vi "单体采集信息.vi"(0 "can卡类型":u8, 1 "设备索引号":u8, 2 "CAN端口":u8, 3 "VIC_Receive":refnum<vi>, 4 "数据":refnum<vi>, 5 "数据位置":refnum<vi>) -> ()   [LabVIEW 2013]
panel:
  out "Life:":dbl=25.0
  in  "213":bool
  in  "一次置位":bool
  in  "刷新":bool
  out "VCI_Receive 2":T1
  in  "板号":u8
  out "电池信息":T2
  in  "电池信息读取":bool
  out "时间":string
  in  "充电均衡":u32(colorbox)=6618880
  in  "放电均衡":u32(colorbox)=16711680
  out "均衡信息":string[][](table)=[["第1串", "1", "单体检测其它故障", "第25串", "1", "单体检测其它故障", "第49串", "1", "单体检测其它故障", "第73串", "1", "单体检测其它故障", "第97串", "1", "单体检测其它故障", "第121串", "1", "单体检测其它故障", "第145串", "1", "单体检测其它故障", "第169串", "1", "单体检测其它故障", "第193串", "1", "单体检测其它故障", "第217串", "1", "单体检测其它故障", "第241串", "1", "单体检测其它故障", "第265串", "1", "单体检测其它故障", "第289串", "1", "单体检测其它故障", ""], ["第2串", "", "", "第26串", "", "", "第50串", "", "", "第74串", "", "", "第98串", "", "", "第122串", "", "", "第146串", "", "", "第170串", "", "", "第194串", "", "", "第218串", "", "", "第242串", "", "", "第266串", "", "", "第290串", "", "", ""], ["第3串", "", "", "第27串", "", "", "第51串", "", "", "第75串", "", "", "第99串", "", "", "第123串", "", "", "第147串", "", "", "第171串", "", "", "第195串", "", "", "第219串", "", "", "第243串", "", "", "第267串", "", "", "第291串", "", "", ""], ["第4串", "", "", "第28串", "", "", "第52串", "", "", "第76串", "", "", "第100串", "", "", "第124串", "", "", "第148串", "", "", "第172串", "", "", "第196串", "", "", "第220串", "", "", "第244串", "", "", "第268串", "", "", "第292串", "", "", ""], ["第5串", "", "", "第29串", "", "", "第53串", "", "", "第77串", "", "", "第101串", "", "", "第125串", "", "", "第149串", "", "", "第173串", "", "", "第197串", "", "", "第221串", "", "", "第245串", "", "", "第269串", "", "", "第293串", "", "", ""], ["第6串", "", "", "第30串", "", "", "第54串", "", "", "第78串", "", "", "第102串", "", "", "第126串", "", "", "第150串", "", "", "第174串", "", "", "第198串", "", "", "第222串", "", "", "第246串", "", "", "第270串", "", "", "第294串", "", "", ""], ["第7串", "", "", "第31串", "", "", "第55串", "", "", "第79串", "", "", "第103串", "", "", "第127串", "", "", "第151串", "", "", "第175串", "", "", "第199串", "", "", "第223串", "", "", "第247串", "", "", "第271串", "", "", "第295串", "", "", ""], ["第8串", "", "", "第32串", "", "", "第56串", "", "", "第80串", "", "", "第104串", "", "", "第128串", "", "", "第152串", "", "", "第176串", "", "", "第200串", "", "", "第224串", "", "", "第248串", "", "", "第272串", "", "", "第296串", "", "", ""], ["第9串", "", "", "第33串", "", "", "第57串", "", "", "第81串", "", "", "第105串", "", "", "第129串", "", "", "第153串", "", "", "第177串", "", "", "第201串", "", "", "第225串", "", "", "第249串", "", "", "第273串", "", "", "第297串", "", "", ""], ["第10串", "", "", "第34串", "", "", "第58串", "", "", "第82串", "", "", "第106串", "", "", "第130串", "", "", "第154串", "", "", "第178串", "", "", "第202串", "", "", "第226串", "", "", "第250串", "", "", "第274串", "", "", "第298串", "", "", ""], ["第11串", "", "", "第35串", "", "", "第59串", "", "", "第83串", "", "", "第107串", "", "", "第131串", "", "", "第155串", "", "", "第179串", "", "", "第203串", "", "", "第227串", "", "", "第251串", "", "", "第275串", "", "", "第299串", "", "", ""], ["第12串", "", "", "第36串", "", "", "第60串", "", "", "第84串", "", "", "第108串", "", "", "第132串", "", "", "第156串", "", "", "第180串", "", "", "第204串", "", "", "第228串", "", "", "第252串", "", "", "第276串", "", "", "第300串", "", "", ""], ["第13串", "", "", "第37串", "", "", "第61串", "", "", "第85串", "", "", "第109串", "", "", "第133串", "", "", "第157串", "", "", "第181串", "", "", "第205串", "", "", "第229串", "", "", "第253串", "", "", "第277串", "", "", "", "", "", ""], ["第14串", "", "", "第38串", "", "", "第62串", "", "", "第86串", "", "", "第110串", "", "", "第134串", "", "", "第158串", "", "", "第182串", "", "", "第206串", "", "", "第230串", "", "", "第254串", "", "", "第278串", "", "", "", "", "", ""], ["第15串", "", "", "第39串", "", "", "第63串", "", "", "第87串", "", "", "第111串", "", "", "第135串", "", "", "第159串", "", "", "第183串", "", "", "第207串", "", "", "第231串", "", "", "第255串", "", "", "第279串", "", "", "", "", "", ""], ["第16串", "", "", "第40串", "", "", "第64串", "", "", "第88串", "", "", "第112串", "", "", "第136串", "", "", "第160串", "", "", "第184串", "", "", "第208串", "", "", "第232串", "", "", "第256串", "", "", "第280串", "", "", "", "", "", ""], ["第17串", "", "", "第41串", "", "", "第65串", "", "", "第89串", "", "", "第113串", "", "", "第137串", "", "", "第161串", "", "", "第185串", "", "", "第209串", "", "", "第233串", "", "", "第257串", "", "", "第281串", "", "", "", "", "", ""], ["第18串", "", "", "第42串", "", "", "第66串", "", "", "第90串", "", "", "第114串", "", "", "第138串", "", "", "第162串", "", "", "第186串", "", "", "第210串", "", "", "第234串", "", "", "第258串", "", "", "第282串", "", "", "", "", "", ""], ["第19串", "", "", "第43串", "", "", "第67串", "", "", "第91串", "", "", "第115串", "", "", "第139串", "", "", "第163串", "", "", "第187串", "", "", "第211串", "", "", "第235串", "", "", "第259串", "", "", "第283串", "", "", "", "", "", ""], ["第20串", "", "", "第44串", "", "", "第68串", "", "", "第92串", "", "", "第116串", "", "", "第140串", "", "", "第164串", "", "", "第188串", "", "", "第212串", "", "", "第236串", "", "", "第260串", "", "", "第284串", "", "", "", "", "", ""], ["第21串", "", "", "第45串", "", "", "第69串", "", "", "第93串", "", "", "第117串", "", "", "第141串", "", "", "第165串", "", "", "第189串", "", "", "第213串", "", "", "第237串", "", "", "第261串", "", "", "第285串", "", "", "", "", "", ""], ["第22串", "", "", "第46串", "", "", "第70串", "", "", "第94串", "", "", "第118串", "", "", "第142串", "", "", "第166串", "", "", "第190串", "", "", "第214串", "", "", "第238串", "", "", "第262串", "", "", "第286串", "", "", "", "", "", ""], ["第23串", "", "", "第47串", "", "", "第71串", "", "", "第95串", "", "", "第119串", "", "", "第143串", "", "", "第167串", "", "", "第191串", "", "", "第215串", "", "", "第239串", "", "", "第263串", "", "", "第287串", "", "", "", "", "", ""], ["第24串", "", "", "第48串", "", "", "第72串", "", "", "第96串", "", "", "第120串", "", "", "第144串", "", "", "第168串", "", "", "第192串", "", "", "第216串", "", "", "第240串", "", "", "第264串", "", "", "第288串", "", "", "", "", "", ""]]
  out "SOC":string[][](table)=[["第1串", "", "", "第25串", "", "", "第49串", "", "", "第73串", "", "", "第97串", "", "", "第121串", "", "", "第145串", "", "", "第169串", "", "", "第193串", "", "", "第217串", "", "", "第241串", "", "", "第265串", "", "", "第289串", "", "", ""], ["第2串", "", "", "第26串", "", "", "第50串", "", "", "第74串", "", "", "第98串", "", "", "第122串", "", "", "第146串", "", "", "第170串", "", "", "第194串", "", "", "第218串", "", "", "第242串", "", "", "第266串", "", "", "第290串", "", "", ""], ["第3串", "", "", "第27串", "", "", "第51串", "", "", "第75串", "", "", "第99串", "", "", "第123串", "", "", "第147串", "", "", "第171串", "", "", "第195串", "", "", "第219串", "", "", "第243串", "", "", "第267串", "", "", "第291串", "", "", ""], ["第4串", "", "", "第28串", "", "", "第52串", "", "", "第76串", "", "", "第100串", "", "", "第124串", "", "", "第148串", "", "", "第172串", "", "", "第196串", "", "", "第220串", "", "", "第244串", "", "", "第268串", "", "", "第292串", "", "", ""], ["第5串", "", "", "第29串", "", "", "第53串", "", "", "第77串", "", "", "第101串", "", "", "第125串", "", "", "第149串", "", "", "第173串", "", "", "第197串", "", "", "第221串", "", "", "第245串", "", "", "第269串", "", "", "第293串", "", "", ""], ["第6串", "", "", "第30串", "", "", "第54串", "", "", "第78串", "", "", "第102串", "", "", "第126串", "", "", "第150串", "", "", "第174串", "", "", "第198串", "", "", "第222串", "", "", "第246串", "", "", "第270串", "", "", "第294串", "", "", ""], ["第7串", "", "", "第31串", "", "", "第55串", "", "", "第79串", "", "", "第103串", "", "", "第127串", "", "", "第151串", "", "", "第175串", "", "", "第199串", "", "", "第223串", "", "", "第247串", "", "", "第271串", "", "", "第295串", "", "", ""], ["第8串", "", "", "第32串", "", "", "第56串", "", "", "第80串", "", "", "第104串", "", "", "第128串", "", "", "第152串", "", "", "第176串", "", "", "第200串", "", "", "第224串", "", "", "第248串", "", "", "第272串", "", "", "第296串", "", "", ""], ["第9串", "", "", "第33串", "", "", "第57串", "", "", "第81串", "", "", "第105串", "", "", "第129串", "", "", "第153串", "", "", "第177串", "", "", "第201串", "", "", "第225串", "", "", "第249串", "", "", "第273串", "", "", "第297串", "", "", ""], ["第10串", "", "", "第34串", "", "", "第58串", "", "", "第82串", "", "", "第106串", "", "", "第130串", "", "", "第154串", "", "", "第178串", "", "", "第202串", "", "", "第226串", "", "", "第250串", "", "", "第274串", "", "", "第298串", "", "", ""], ["第11串", "", "", "第35串", "", "", "第59串", "", "", "第83串", "", "", "第107串", "", "", "第131串", "", "", "第155串", "", "", "第179串", "", "", "第203串", "", "", "第227串", "", "", "第251串", "", "", "第275串", "", "", "第299串", "", "", ""], ["第12串", "", "", "第36串", "", "", "第60串", "", "", "第84串", "", "", "第108串", "", "", "第132串", "", "", "第156串", "", "", "第180串", "", "", "第204串", "", "", "第228串", "", "", "第252串", "", "", "第276串", "", "", "第300串", "", "", ""], ["第13串", "", "", "第37串", "", "", "第61串", "", "", "第85串", "", "", "第109串", "", "", "第133串", "", "", "第157串", "", "", "第181串", "", "", "第205串", "", "", "第229串", "", "", "第253串", "", "", "第277串", "", "", "", "", "", ""], ["第14串", "", "", "第38串", "", "", "第62串", "", "", "第86串", "", "", "第110串", "", "", "第134串", "", "", "第158串", "", "", "第182串", "", "", "第206串", "", "", "第230串", "", "", "第254串", "", "", "第278串", "", "", "", "", "", ""], ["第15串", "", "", "第39串", "", "", "第63串", "", "", "第87串", "", "", "第111串", "", "", "第135串", "", "", "第159串", "", "", "第183串", "", "", "第207串", "", "", "第231串", "", "", "第255串", "", "", "第279串", "", "", "", "", "", ""], ["第16串", "", "", "第40串", "", "", "第64串", "", "", "第88串", "", "", "第112串", "", "", "第136串", "", "", "第160串", "", "", "第184串", "", "", "第208串", "", "", "第232串", "", "", "第256串", "", "", "第280串", "", "", "", "", "", ""], ["第17串", "", "", "第41串", "", "", "第65串", "", "", "第89串", "", "", "第113串", "", "", "第137串", "", "", "第161串", "", "", "第185串", "", "", "第209串", "", "", "第233串", "", "", "第257串", "", "", "第281串", "", "", "", "", "", ""], ["第18串", "", "", "第42串", "", "", "第66串", "", "", "第90串", "", "", "第114串", "", "", "第138串", "", "", "第162串", "", "", "第186串", "", "", "第210串", "", "", "第234串", "", "", "第258串", "", "", "第282串", "", "", "", "", "", ""], ["第19串", "", "", "第43串", "", "", "第67串", "", "", "第91串", "", "", "第115串", "", "", "第139串", "", "", "第163串", "", "", "第187串", "", "", "第211串", "", "", "第235串", "", "", "第259串", "", "", "第283串", "", "", "", "", "", ""], ["第20串", "", "", "第44串", "", "", "第68串", "", "", "第92串", "", "", "第116串", "", "", "第140串", "", "", "第164串", "", "", "第188串", "", "", "第212串", "", "", "第236串", "", "", "第260串", "", "", "第284串", "", "", "", "", "", ""], ["第21串", "", "", "第45串", "", "", "第69串", "", "", "第93串", "", "", "第117串", "", "", "第141串", "", "", "第165串", "", "", "第189串", "", "", "第213串", "", "", "第237串", "", "", "第261串", "", "", "第285串", "", "", "", "", "", ""], ["第22串", "", "", "第46串", "", "", "第70串", "", "", "第94串", "", "", "第118串", "", "", "第142串", "", "", "第166串", "", "", "第190串", "", "", "第214串", "", "", "第238串", "", "", "第262串", "", "", "第286串", "", "", "", "", "", ""], ["第23串", "", "", "第47串", "", "", "第71串", "", "", "第95串", "", "", "第119串", "", "", "第143串", "", "", "第167串", "", "", "第191串", "", "", "第215串", "", "", "第239串", "", "", "第263串", "", "", "第287串", "", "", "", "", "", ""], ["第24串", "", "", "第48串", "", "", "第72串", "", "", "第96串", "", "", "第120串", "", "", "第144串", "", "", "第168串", "", "", "第192串", "", "", "第216串", "", "", "第240串", "", "", "第264串", "", "", "第288串", "", "", "", "", "", ""]]
  out "内阻":string[][](table)=[["第1串", "", "", "第25串", "", "", "第49串", "", "", "第73串", "", "", "第97串", "", "", "第121串", "", "", "第145串", "", "", "第169串", "", "", "第193串", "", "", "第217串", "", "", "第241串", "", "", "第265串", "", "", "第289串", "", "", ""], ["第2串", "", "", "第26串", "", "", "第50串", "", "", "第74串", "", "", "第98串", "", "", "第122串", "", "", "第146串", "", "", "第170串", "", "", "第194串", "", "", "第218串", "", "", "第242串", "", "", "第266串", "", "", "第290串", "", "", ""], ["第3串", "", "", "第27串", "", "", "第51串", "", "", "第75串", "", "", "第99串", "", "", "第123串", "", "", "第147串", "", "", "第171串", "", "", "第195串", "", "", "第219串", "", "", "第243串", "", "", "第267串", "", "", "第291串", "", "", ""], ["第4串", "", "", "第28串", "", "", "第52串", "", "", "第76串", "", "", "第100串", "", "", "第124串", "", "", "第148串", "", "", "第172串", "", "", "第196串", "", "", "第220串", "", "", "第244串", "", "", "第268串", "", "", "第292串", "", "", ""], ["第5串", "", "", "第29串", "", "", "第53串", "", "", "第77串", "", "", "第101串", "", "", "第125串", "", "", "第149串", "", "", "第173串", "", "", "第197串", "", "", "第221串", "", "", "第245串", "", "", "第269串", "", "", "第293串", "", "", ""], ["第6串", "", "", "第30串", "", "", "第54串", "", "", "第78串", "", "", "第102串", "", "", "第126串", "", "", "第150串", "", "", "第174串", "", "", "第198串", "", "", "第222串", "", "", "第246串", "", "", "第270串", "", "", "第294串", "", "", ""], ["第7串", "", "", "第31串", "", "", "第55串", "", "", "第79串", "", "", "第103串", "", "", "第127串", "", "", "第151串", "", "", "第175串", "", "", "第199串", "", "", "第223串", "", "", "第247串", "", "", "第271串", "", "", "第295串", "", "", ""], ["第8串", "", "", "第32串", "", "", "第56串", "", "", "第80串", "", "", "第104串", "", "", "第128串", "", "", "第152串", "", "", "第176串", "", "", "第200串", "", "", "第224串", "", "", "第248串", "", "", "第272串", "", "", "第296串", "", "", ""], ["第9串", "", "", "第33串", "", "", "第57串", "", "", "第81串", "", "", "第105串", "", "", "第129串", "", "", "第153串", "", "", "第177串", "", "", "第201串", "", "", "第225串", "", "", "第249串", "", "", "第273串", "", "", "第297串", "", "", ""], ["第10串", "", "", "第34串", "", "", "第58串", "", "", "第82串", "", "", "第106串", "", "", "第130串", "", "", "第154串", "", "", "第178串", "", "", "第202串", "", "", "第226串", "", "", "第250串", "", "", "第274串", "", "", "第298串", "", "", ""], ["第11串", "", "", "第35串", "", "", "第59串", "", "", "第83串", "", "", "第107串", "", "", "第131串", "", "", "第155串", "", "", "第179串", "", "", "第203串", "", "", "第227串", "", "", "第251串", "", "", "第275串", "", "", "第299串", "", "", ""], ["第12串", "", "", "第36串", "", "", "第60串", "", "", "第84串", "", "", "第108串", "", "", "第132串", "", "", "第156串", "", "", "第180串", "", "", "第204串", "", "", "第228串", "", "", "第252串", "", "", "第276串", "", "", "第300串", "", "", ""], ["第13串", "", "", "第37串", "", "", "第61串", "", "", "第85串", "", "", "第109串", "", "", "第133串", "", "", "第157串", "", "", "第181串", "", "", "第205串", "", "", "第229串", "", "", "第253串", "", "", "第277串", "", "", "", "", "", ""], ["第14串", "", "", "第38串", "", "", "第62串", "", "", "第86串", "", "", "第110串", "", "", "第134串", "", "", "第158串", "", "", "第182串", "", "", "第206串", "", "", "第230串", "", "", "第254串", "", "", "第278串", "", "", "", "", "", ""], ["第15串", "", "", "第39串", "", "", "第63串", "", "", "第87串", "", "", "第111串", "", "", "第135串", "", "", "第159串", "", "", "第183串", "", "", "第207串", "", "", "第231串", "", "", "第255串", "", "", "第279串", "", "", "", "", "", ""], ["第16串", "", "", "第40串", "", "", "第64串", "", "", "第88串", "", "", "第112串", "", "", "第136串", "", "", "第160串", "", "", "第184串", "", "", "第208串", "", "", "第232串", "", "", "第256串", "", "", "第280串", "", "", "", "", "", ""], ["第17串", "", "", "第41串", "", "", "第65串", "", "", "第89串", "", "", "第113串", "", "", "第137串", "", "", "第161串", "", "", "第185串", "", "", "第209串", "", "", "第233串", "", "", "第257串", "", "", "第281串", "", "", "", "", "", ""], ["第18串", "", "", "第42串", "", "", "第66串", "", "", "第90串", "", "", "第114串", "", "", "第138串", "", "", "第162串", "", "", "第186串", "", "", "第210串", "", "", "第234串", "", "", "第258串", "", "", "第282串", "", "", "", "", "", ""], ["第19串", "", "", "第43串", "", "", "第67串", "", "", "第91串", "", "", "第115串", "", "", "第139串", "", "", "第163串", "", "", "第187串", "", "", "第211串", "", "", "第235串", "", "", "第259串", "", "", "第283串", "", "", "", "", "", ""], ["第20串", "", "", "第44串", "", "", "第68串", "", "", "第92串", "", "", "第116串", "", "", "第140串", "", "", "第164串", "", "", "第188串", "", "", "第212串", "", "", "第236串", "", "", "第260串", "", "", "第284串", "", "", "", "", "", ""], ["第21串", "", "", "第45串", "", "", "第69串", "", "", "第93串", "", "", "第117串", "", "", "第141串", "", "", "第165串", "", "", "第189串", "", "", "第213串", "", "", "第237串", "", "", "第261串", "", "", "第285串", "", "", "", "", "", ""], ["第22串", "", "", "第46串", "", "", "第70串", "", "", "第94串", "", "", "第118串", "", "", "第142串", "", "", "第166串", "", "", "第190串", "", "", "第214串", "", "", "第238串", "", "", "第262串", "", "", "第286串", "", "", "", "", "", ""], ["第23串", "", "", "第47串", "", "", "第71串", "", "", "第95串", "", "", "第119串", "", "", "第143串", "", "", "第167串", "", "", "第191串", "", "", "第215串", "", "", "第239串", "", "", "第263串", "", "", "第287串", "", "", "", "", "", ""], ["第24串", "", "", "第48串", "", "", "第72串", "", "", "第96串", "", "", "第120串", "", "", "第144串", "", "", "第168串", "", "", "第192串", "", "", "第216串", "", "", "第240串", "", "", "第264串", "", "", "第288串", "", "", "", "", "", ""]]
  out "温度表格":string[][](table)=[["第1串", "", "", "第25串", "", "", "第49串", "", "", "第73串", "", "", "第97串", "", "", "第121串", "", "", "第145串", "", "", "第169串", "", "", "第193串", "", "", "第217串", "", "", "第241串", "", "", "第265串", "", "", "第289串", "", "", ""], ["第2串", "", "", "第26串", "", "", "第50串", "", "", "第74串", "", "", "第98串", "", "", "第122串", "", "", "第146串", "", "", "第170串", "", "", "第194串", "", "", "第218串", "", "", "第242串", "", "", "第266串", "", "", "第290串", "", "", ""], ["第3串", "", "", "第27串", "", "", "第51串", "", "", "第75串", "", "", "第99串", "", "", "第123串", "", "", "第147串", "", "", "第171串", "", "", "第195串", "", "", "第219串", "", "", "第243串", "", "", "第267串", "", "", "第291串", "", "", ""], ["第4串", "", "", "第28串", "", "", "第52串", "", "", "第76串", "", "", "第100串", "", "", "第124串", "", "", "第148串", "", "", "第172串", "", "", "第196串", "", "", "第220串", "", "", "第244串", "", "", "第268串", "", "", "第292串", "", "", ""], ["第5串", "", "", "第29串", "", "", "第53串", "", "", "第77串", "", "", "第101串", "", "", "第125串", "", "", "第149串", "", "", "第173串", "", "", "第197串", "", "", "第221串", "", "", "第245串", "", "", "第269串", "", "", "第293串", "", "", ""], ["第6串", "", "", "第30串", "", "", "第54串", "", "", "第78串", "", "", "第102串", "", "", "第126串", "", "", "第150串", "", "", "第174串", "", "", "第198串", "", "", "第222串", "", "", "第246串", "", "", "第270串", "", "", "第294串", "", "", ""], ["第7串", "", "", "第31串", "", "", "第55串", "", "", "第79串", "", "", "第103串", "", "", "第127串", "", "", "第151串", "", "", "第175串", "", "", "第199串", "", "", "第223串", "", "", "第247串", "", "", "第271串", "", "", "第295串", "", "", ""], ["第8串", "", "", "第32串", "", "", "第56串", "", "", "第80串", "", "", "第104串", "", "", "第128串", "", "", "第152串", "", "", "第176串", "", "", "第200串", "", "", "第224串", "", "", "第248串", "", "", "第272串", "", "", "第296串", "", "", ""], ["第9串", "", "", "第33串", "", "", "第57串", "", "", "第81串", "", "", "第105串", "", "", "第129串", "", "", "第153串", "", "", "第177串", "", "", "第201串", "", "", "第225串", "", "", "第249串", "", "", "第273串", "", "", "第297串", "", "", ""], ["第10串", "", "", "第34串", "", "", "第58串", "", "", "第82串", "", "", "第106串", "", "", "第130串", "", "", "第154串", "", "", "第178串", "", "", "第202串", "", "", "第226串", "", "", "第250串", "", "", "第274串", "", "", "第298串", "", "", ""], ["第11串", "", "", "第35串", "", "", "第59串", "", "", "第83串", "", "", "第107串", "", "", "第131串", "", "", "第155串", "", "", "第179串", "", "", "第203串", "", "", "第227串", "", "", "第251串", "", "", "第275串", "", "", "第299串", "", "", ""], ["第12串", "", "", "第36串", "", "", "第60串", "", "", "第84串", "", "", "第108串", "", "", "第132串", "", "", "第156串", "", "", "第180串", "", "", "第204串", "", "", "第228串", "", "", "第252串", "", "", "第276串", "", "", "第300串", "", "", ""], ["第13串", "", "", "第37串", "", "", "第61串", "", "", "第85串", "", "", "第109串", "", "", "第133串", "", "", "第157串", "", "", "第181串", "", "", "第205串", "", "", "第229串", "", "", "第253串", "", "", "第277串", "", "", "", "", "", ""], ["第14串", "", "", "第38串", "", "", "第62串", "", "", "第86串", "", "", "第110串", "", "", "第134串", "", "", "第158串", "", "", "第182串", "", "", "第206串", "", "", "第230串", "", "", "第254串", "", "", "第278串", "", "", "", "", "", ""], ["第15串", "", "", "第39串", "", "", "第63串", "", "", "第87串", "", "", "第111串", "", "", "第135串", "", "", "第159串", "", "", "第183串", "", "", "第207串", "", "", "第231串", "", "", "第255串", "", "", "第279串", "", "", "", "", "", ""], ["第16串", "", "", "第40串", "", "", "第64串", "", "", "第88串", "", "", "第112串", "", "", "第136串", "", "", "第160串", "", "", "第184串", "", "", "第208串", "", "", "第232串", "", "", "第256串", "", "", "第280串", "", "", "", "", "", ""], ["第17串", "", "", "第41串", "", "", "第65串", "", "", "第89串", "", "", "第113串", "", "", "第137串", "", "", "第161串", "", "", "第185串", "", "", "第209串", "", "", "第233串", "", "", "第257串", "", "", "第281串", "", "", "", "", "", ""], ["第18串", "", "", "第42串", "", "", "第66串", "", "", "第90串", "", "", "第114串", "", "", "第138串", "", "", "第162串", "", "", "第186串", "", "", "第210串", "", "", "第234串", "", "", "第258串", "", "", "第282串", "", "", "", "", "", ""], ["第19串", "", "", "第43串", "", "", "第67串", "", "", "第91串", "", "", "第115串", "", "", "第139串", "", "", "第163串", "", "", "第187串", "", "", "第211串", "", "", "第235串", "", "", "第259串", "", "", "第283串", "", "", "", "", "", ""], ["第20串", "", "", "第44串", "", "", "第68串", "", "", "第92串", "", "", "第116串", "", "", "第140串", "", "", "第164串", "", "", "第188串", "", "", "第212串", "", "", "第236串", "", "", "第260串", "", "", "第284串", "", "", "", "", "", ""], ["第21串", "", "", "第45串", "", "", "第69串", "", "", "第93串", "", "", "第117串", "", "", "第141串", "", "", "第165串", "", "", "第189串", "", "", "第213串", "", "", "第237串", "", "", "第261串", "", "", "第285串", "", "", "", "", "", ""], ["第22串", "", "", "第46串", "", "", "第70串", "", "", "第94串", "", "", "第118串", "", "", "第142串", "", "", "第166串", "", "", "第190串", "", "", "第214串", "", "", "第238串", "", "", "第262串", "", "", "第286串", "", "", "", "", "", ""], ["第23串", "", "", "第47串", "", "", "第71串", "", "", "第95串", "", "", "第119串", "", "", "第143串", "", "", "第167串", "", "", "第191串", "", "", "第215串", "", "", "第239串", "", "", "第263串", "", "", "第287串", "", "", "", "", "", ""], ["第24串", "", "", "第48串", "", "", "第72串", "", "", "第96串", "", "", "第120串", "", "", "第144串", "", "", "第168串", "", "", "第192串", "", "", "第216串", "", "", "第240串", "", "", "第264串", "", "", "第288串", "", "", "", "", "", ""]]
  in  "主界面选项":T3(radio)
  in  "电池信息选项":enum16{"电池信息", "历史信息"}(ring)
  out "位置":dbl[](array[numeric])
  out "输出数据":dbl[](array[numeric])
  in  "命令":u32=133
  in  "VCI_Receive":T1 {"Rsv3" max=0 format="%x"; "Rsv2" min=101 format="%x"; "Rsv1" format="%x"; "Data8" format="%x"; "Data7" format="%x"; "Data6" format="%x"; "Data5" format="%x"; "Data4" format="%x"; "Data3" format="%x"; "Data2" format="%x"; "Data1" format="%x"; "DataLen" format="%x"; "ExternFlag" format="%x"; "RemoteFlag" format="%x"; "SendType" format="%x"; "TimeFlag" format="%x"; "TimeStamp" format="%x"; "ID" format="%x"}
  out "状态":bool
  in  "停止":bool
  in  "选项卡控件":enum32{"单体电压", "单体温度", "单体内阻", "单体SOC"}(tab)
  in  "偏差":dbl=0.008 format="%.3f"
  in  "基准":dbl=3.3 format="%.3f"
  out "等待均衡":u32(colorbox)=16776770
  in  "故障信息选择按键 2":enum32{"单选选项2", "单选选项2 2", "单选选项2 3", "单选选项1"}(radio)=enum."单选选项1"
  out "电压选择":enum32{"1-96", "97-192", "193-288", "289-300"}(tab)
  out "1":T4={"1 102"={"第1串"=0.0, "第2串"=0.0, "第3串"=0.0, "第4串"=0.0, "第5串"=0.0, "第6串"=0.0, "第7串"=0.0, "第8串"=0.0, "第9串"=0.0, "第10串"=0.0, "第11串"=0.0, "第12串"=0.0, "第一串 2"=0.0, "第一串 4"=0.0, "第一串 6"=0.0, "第一串 8"=0.0, "第一串 10"=0.0, "第一串 12"=0.0, "第一串 14"=0.0, "第一串 16"=0.0, "第一串 18"=0.0, "第一串 20"=0.0, "第一串 22"=0.0, "第一串 24"=0.0}, "1 3"={"第13串"=0.0, "第14串"=0.0, "第15串"=0.0, "第16串"=0.0, "第17串"=0.0, "第18串"=0.0, "第19串"=0.0, "第20串"=0.0, "第21串"=0.0, "第22串"=0.0, "第23串"=0.0, "第24串"=0.0, "第一串 2"=0.0, "第一串 4"=0.0, "第一串 6"=0.0, "第一串 8"=0.0, "第一串 10"=0.0, "第一串 12"=0.0, "第一串 14"=0.0, "第一串 16"=0.0, "第一串 18"=0.0, "第一串 20"=0.0, "第一串 22"=0.0, "第一串 24"=0.0}, "1 4"={"第25串"=0.0, "第26串"=0.0, "第27串"=0.0, "第28串"=0.0, "第29串"=0.0, "第30串"=0.0, "第31串"=0.0, "第32串"=0.0, "第33串"=0.0, "第34串"=0.0, "第35串"=0.0, "第36串"=0.0, "第一串 2"=0.0, "第一串 4"=0.0, "第一串 6"=0.0, "第一串 8"=0.0, "第一串 10"=0.0, "第一串 12"=0.0, "第一串 14"=0.0, "第一串 16"=0.0, "第一串 18"=0.0, "第一串 20"=0.0, "第一串 22"=0.0, "第一串 24"=0.0}, "1 6"={"第37串"=0.0, "第38串"=0.0, "第39串"=0.0, "第40串"=0.0, "第41串"=0.0, "第42串"=0.0, "第43串"=0.0, "第44串"=0.0, "第45串"=0.0, "第46串"=0.0, "第47串"=0.0, "第48串"=0.0, "第一串 2"=0.0, "第一串 4"=0.0, "第一串 6"=0.0, "第一串 8"=0.0, "第一串 10"=0.0, "第一串 12"=0.0, "第一串 14"=0.0, "第一串 16"=0.0, "第一串 18"=0.0, "第一串 20"=0.0, "第一串 22"=0.0, "第一串 24"=0.0}, "1 7"={"第49串"=0.0, "第50串"=0.0, "第51串"=0.0, "第52串"=0.0, "第53串"=0.0, "第54串"=0.0, "第55串"=0.0, "第56串"=0.0, "第57串"=0.0, "第58串"=0.0, "第59串"=0.0, "第60串"=0.0, "第一串 2"=0.0, "第一串 4"=0.0, "第一串 6"=0.0, "第一串 8"=0.0, "第一串 10"=0.0, "第一串 12"=0.0, "第一串 14"=0.0, "第一串 16"=0.0, "第一串 18"=0.0, "第一串 20"=0.0, "第一串 22"=0.0, "第一串 24"=0.0}, "1 8"={"第61串"=0.0, "第62串"=0.0, "第63串"=0.0, "第64串"=0.0, "第65串"=0.0, "第66串"=0.0, "第67串"=0.0, "第68串"=0.0, "第69串"=0.0, "第70串"=0.0, "第71串"=0.0, "第72串"=0.0, "第一串 2"=0.0, "第一串 4"=0.0, "第一串 6"=0.0, "第一串 8"=0.0, "第一串 10"=0.0, "第一串 12"=0.0, "第一串 14"=0.0, "第一串 16"=0.0, "第一串 18"=0.0, "第一串 20"=0.0, "第一串 22"=0.0, "第一串 24"=0.0}, "1 9"={"第73串"=0.0, "第74串"=0.0, "第75串"=0.0, "第76串"=0.0, "第77串"=0.0, "第78串"=0.0, "第79串"=0.0, "第80串"=0.0, "第81串"=0.0, "第82串"=0.0, "第83串"=0.0, "第84串"=0.0, "第一串 2"=0.0, "第一串 4"=0.0, "第一串 6"=0.0, "第一串 8"=0.0, "第一串 10"=0.0, "第一串 12"=0.0, "第一串 14"=0.0, "第一串 16"=0.0, "第一串 18"=0.0, "第一串 20"=0.0, "第一串 22"=0.0, "第一串 24"=0.0}, "1 10"={"第85串"=0.0, "第86串"=0.0, "第87串"=0.0, "第88串"=0.0, "第89串"=0.0, "第90串"=0.0, "第91串"=0.0, "第92串"=0.0, "第93串"=0.0, "第94串"=0.0, "第95串"=0.0, "第96串"=0.0, "第一串 2"=0.0, "第一串 4"=0.0, "第一串 6"=0.0, "第一串 8"=0.0, "第一串 10"=0.0, "第一串 12"=0.0, "第一串 14"=0.0, "第一串 16"=0.0, "第一串 18"=0.0, "第一串 20"=0.0, "第一串 22"=0.0, "第一串 24"=0.0}, "1 12"={"充电1"=13816530, "充电1"=13816530, "充电1"=13816530, "充电1"=13816530, "充电1"=13816530, "充电1"=13816530, "充电1"=13816530, "充电1"=13816530, "充电1"=13816530, "充电1"=13816530, "充电1"=13816530, "充电1"=13816530}, "1 28"={"充电1"=13816530, "充电1"=13816530, "充电1"=13816530, "充电1"=13816530, "充电1"=13816530, "充电1"=13816530, "充电1"=13816530, "充电1"=13816530, "充电1"=13816530, "充电1"=13816530, "充电1"=13816530, "充电1"=13816530}, "1 25"={"充电1"=0, "充电1"=0, "充电1"=0, "充电1"=0, "充电1"=0, "充电1"=0, "充电1"=0, "充电1"=0, "充电1"=0, "充电1"=0, "充电1"=0, "充电1"=0}, "1 31"={"充电1"=0, "充电1"=0, "充电1"=0, "充电1"=0, "充电1"=0, "充电1"=0, "充电1"=0, "充电1"=0, "充电1"=0, "充电1"=0, "充电1"=0, "充电1"=0}, "1 16"={"充电1"=0, "充电1"=0, "充电1"=0, "充电1"=0, "充电1"=0, "充电1"=0, "充电1"=0, "充电1"=0, "充电1"=0, "充电1"=0, "充电1"=0, "充电1"=0}, "1 19"={"充电1"=0, "充电1"=0, "充电1"=0, "充电1"=0, "充电1"=0, "充电1"=0, "充电1"=0, "充电1"=0, "充电1"=0, "充电1"=0, "充电1"=0, "充电1"=0}, "1 22"={"充电1"=0, "充电1"=0, "充电1"=0, "充电1"=0, "充电1"=0, "充电1"=0, "充电1"=0, "充电1"=0, "充电1"=0, "充电1"=0, "充电1"=0, "充电1"=0}, "1 34"={"充电1"=0, "充电1"=0, "充电1"=0, "充电1"=0, "充电1"=0, "充电1"=0, "充电1"=0, "充电1"=0, "充电1"=0, "充电1"=0, "充电1"=0, "充电1"=0}, "1 11"={"充电1"=13816530, "充电1"=13816530, "充电1"=13816530, "充电1"=13816530, "充电1"=13816530, "充电1"=13816530, "充电1"=13816530, "充电1"=13816530, "充电1"=13816530, "充电1"=13816530, "充电1"=13816530, "充电1"=13816530}, "1 27"={"充电1"=0, "充电1"=0, "充电1"=0, "充电1"=0, "充电1"=0, "充电1"=0, "充电1"=0, "充电1"=0, "充电1"=0, "充电1"=0, "充电1"=0, "充电1"=0}, "1 24"={"充电1"=0, "充电1"=0, "充电1"=0, "充电1"=0, "充电1"=0, "充电1"=0, "充电1"=0, "充电1"=0, "充电1"=0, "充电1"=0, "充电1"=0, "充电1"=0}, "1 30"={"充电1"=0, "充电1"=0, "充电1"=0, "充电1"=0, "充电1"=0, "充电1"=0, "充电1"=0, "充电1"=0, "充电1"=0, "充电1"=0, "充电1"=0, "充电1"=0}, "1 15"={"充电1"=0, "充电1"=0, "充电1"=0, "充电1"=0, "充电1"=0, "充电1"=0, "充电1"=0, "充电1"=0, "充电1"=0, "充电1"=0, "充电1"=0, "充电1"=0}, "1 18"={"充电1"=0, "充电1"=0, "充电1"=0, "充电1"=0, "充电1"=0, "充电1"=0, "充电1"=0, "充电1"=0, "充电1"=0, "充电1"=0, "充电1"=0, "充电1"=0}, "1 21"={"充电1"=0, "充电1"=0, "充电1"=0, "充电1"=0, "充电1"=0, "充电1"=0, "充电1"=0, "充电1"=0, "充电1"=0, "充电1"=0, "充电1"=0, "充电1"=0}, "1 33"={"充电1"=0, "充电1"=0, "充电1"=0, "充电1"=0, "充电1"=0, "充电1"=0, "充电1"=0, "充电1"=0, "充电1"=0, "充电1"=0, "充电1"=0, "充电1"=0}, "1 13"={"均衡故障"=0, "均衡故障 2"=0.0, "均衡故障 3"=0.0, "均衡故障 4"=0.0, "均衡故障 5"=0.0, "均衡故障 6"=0.0, "均衡故障 7"=0.0, "均衡故障 8"=0.0, "均衡故障 9"=0.0, "均衡故障 10"=0.0, "均衡故障 11"=0.0, "均衡故障 12"=0.0}, "1 26"={"均衡故障"=0, "均衡故障 2"=0.0, "均衡故障 3"=0.0, "均衡故障 4"=0.0, "均衡故障 5"=0.0, "均衡故障 6"=0.0, "均衡故障 7"=0.0, "均衡故障 8"=0.0, "均衡故障 9"=0.0, "均衡故障 10"=0.0, "均衡故障 11"=0.0, "均衡故障 12"=0.0}, "1 23"={"均衡故障"=0, "均衡故障 2"=0.0, "均衡故障 3"=0.0, "均衡故障 4"=0.0, "均衡故障 5"=0.0, "均衡故障 6"=0.0, "均衡故障 7"=0.0, "均衡故障 8"=0.0, "均衡故障 9"=0.0, "均衡故障 10"=0.0, "均衡故障 11"=0.0, "均衡故障 12"=0.0}, "1 29"={"均衡故障"=0, "均衡故障 2"=0.0, "均衡故障 3"=0.0, "均衡故障 4"=0.0, "均衡故障 5"=0.0, "均衡故障 6"=0.0, "均衡故障 7"=0.0, "均衡故障 8"=0.0, "均衡故障 9"=0.0, "均衡故障 10"=0.0, "均衡故障 11"=0.0, "均衡故障 12"=0.0}, "1 14"={"均衡故障"=0, "均衡故障 2"=0.0, "均衡故障 3"=0.0, "均衡故障 4"=0.0, "均衡故障 5"=0.0, "均衡故障 6"=0.0, "均衡故障 7"=0.0, "均衡故障 8"=0.0, "均衡故障 9"=0.0, "均衡故障 10"=0.0, "均衡故障 11"=0.0, "均衡故障 12"=0.0}, "1 17"={"均衡故障"=0, "均衡故障 2"=0.0, "均衡故障 3"=0.0, "均衡故障 4"=0.0, "均衡故障 5"=0.0, "均衡故障 6"=0.0, "均衡故障 7"=0.0, "均衡故障 8"=0.0, "均衡故障 9"=0.0, "均衡故障 10"=0.0, "均衡故障 11"=0.0, "均衡故障 12"=0.0}, "1 20"={"均衡故障"=0, "均衡故障 2"=0.0, "均衡故障 3"=0.0, "均衡故障 4"=0.0, "均衡故障 5"=0.0, "均衡故障 6"=0.0, "均衡故障 7"=0.0, "均衡故障 8"=0.0, "均衡故障 9"=0.0, "均衡故障 10"=0.0, "均衡故障 11"=0.0, "均衡故障 12"=0.0}, "1 32"={"均衡故障"=0, "均衡故障 2"=0.0, "均衡故障 3"=0.0, "均衡故障 4"=0.0, "均衡故障 5"=0.0, "均衡故障 6"=0.0, "均衡故障 7"=0.0, "均衡故障 8"=0.0, "均衡故障 9"=0.0, "均衡故障 10"=0.0, "均衡故障 11"=0.0, "均衡故障 12"=0.0}} {"1 102"."第一串 24" format="%#.2f"; "1 102"."第12串" format="%.3f"; "1 102"."第一串 22" format="%#.2f"; "1 102"."第11串" format="%.3f"; "1 102"."第一串 20" format="%#.2f"; "1 102"."第10串" format="%.3f"; "1 102"."第一串 18" format="%#.2f"; "1 102"."第9串" format="%.3f"; "1 102"."第一串 16" format="%#.2f"; "1 102"."第8串" format="%.3f"; "1 102"."第一串 14" format="%#.2f"; "1 102"."第7串" format="%.3f"; "1 102"."第一串 12" format="%#.2f"; "1 102"."第6串" format="%.3f"; "1 102"."第一串 10" format="%#.2f"; "1 102"."第5串" format="%.3f"; "1 102"."第一串 8" format="%#.2f"; "1 102"."第4串" format="%.3f"; "1 102"."第一串 6" format="%#.2f"; "1 102"."第3串" format="%.3f"; "1 102"."第一串 4" format="%#.2f"; "1 102"."第2串" format="%.3f"; "1 102"."第一串 2" format="%#.2f"; "1 102"."第1串" format="%.3f"; "1 10"."第96串" format="%.3f"; "1 10"."第95串" format="%.3f"; "1 10"."第94串" format="%.3f"; "1 10"."第93串" format="%.3f"; "1 10"."第92串" format="%.3f"; "1 10"."第91串" format="%.3f"; "1 10"."第90串" format="%.3f"; "1 10"."第89串" format="%.3f"; "1 10"."第88串" format="%.3f"; "1 10"."第87串" format="%.3f"; "1 10"."第86串" format="%.3f"; "1 10"."第85串" format="%.3f"; "1 9"."第84串" format="%.3f"; "1 9"."第83串" format="%.3f"; "1 9"."第82串" format="%.3f"; "1 9"."第81串" format="%.3f"; "1 9"."第80串" format="%.3f"; "1 9"."第79串" format="%.3f"; "1 9"."第78串" format="%.3f"; "1 9"."第77串" format="%.3f"; "1 9"."第76串" format="%.3f"; "1 9"."第75串" format="%.3f"; "1 9"."第74串" format="%.3f"; "1 9"."第73串" format="%.3f"; "1 8"."第72串" format="%.3f"; "1 8"."第71串" format="%.3f"; "1 8"."第70串" format="%.3f"; "1 8"."第69串" format="%.3f"; "1 8"."第68串" format="%.3f"; "1 8"."第67串" format="%.3f"; "1 8"."第66串" format="%.3f"; "1 8"."第65串" format="%.3f"; "1 8"."第64串" format="%.3f"; "1 8"."第63串" format="%.3f"; "1 8"."第62串" format="%.3f"; "1 8"."第61串" format="%.3f"; "1 7"."第60串" format="%.3f"; "1 7"."第59串" format="%.3f"; "1 7"."第58串" format="%.3f"; "1 7"."第57串" format="%.3f"; "1 7"."第56串" format="%.3f"; "1 7"."第55串" format="%.3f"; "1 7"."第54串" format="%.3f"; "1 7"."第53串" format="%.3f"; "1 7"."第52串" format="%.3f"; "1 7"."第51串" format="%.3f"; "1 7"."第50串" format="%.3f"; "1 7"."第49串" format="%.3f"; "1 6"."第48串" format="%.3f"; "1 6"."第47串" format="%.3f"; "1 6"."第46串" format="%.3f"; "1 6"."第45串" format="%.3f"; "1 6"."第44串" format="%.3f"; "1 6"."第43串" format="%.3f"; "1 6"."第42串" format="%.3f"; "1 6"."第41串" format="%.3f"; "1 6"."第40串" format="%.3f"; "1 6"."第39串" format="%.3f"; "1 6"."第38串" format="%.3f"; "1 6"."第37串" format="%.3f"; "1 4"."第36串" format="%.3f"; "1 4"."第35串" format="%.3f"; "1 4"."第34串" format="%.3f"; "1 4"."第33串" format="%.3f"; "1 4"."第32串" format="%.3f"; "1 4"."第31串" format="%.3f"; "1 4"."第30串" format="%.3f"; "1 4"."第29串" format="%.3f"; "1 4"."第28串" format="%.3f"; "1 4"."第27串" format="%.3f"; "1 4"."第26串" format="%.3f"; "1 4"."第25串" format="%.3f"; "1 3"."第24串" format="%.3f"; "1 3"."第23串" format="%.3f"; "1 3"."第22串" format="%.3f"; "1 3"."第21串" format="%.3f"; "1 3"."第20串" format="%.3f"; "1 3"."第19串" format="%.3f"; "1 3"."第18串" format="%.3f"; "1 3"."第17串" format="%.3f"; "1 3"."第16串" format="%.3f"; "1 3"."第15串" format="%.3f"; "1 3"."第14串" format="%.3f"; "1 3"."第13串" format="%.3f"}
  out "2":T5={"1 26"={"第97串"=0.0, "第98串"=0.0, "第99串"=0.0, "第100串"=0.0, "第101串"=0.0, "第102串"=0.0, "第103串"=0.0, "第104串"=0.0, "第105串"=0.0, "第106串"=0.0, "第107串"=0.0, "第108串"=0.0, "第一串 2"=0.0, "第一串 4"=0.0, "第一串 6"=0.0, "第一串 8"=0.0, "第一串 10"=0.0, "第一串 12"=0.0, "第一串 14"=0.0, "第一串 16"=0.0, "第一串 18"=0.0, "第一串 20"=0.0, "第一串 22"=0.0, "第一串 24"=0.0}, "1 27"={"第109串"=0.0, "第110串"=0.0, "第111串"=0.0, "第112串"=0.0, "第113串"=0.0, "第114串"=0.0, "第115串"=0.0, "第116串"=0.0, "第117串"=0.0, "第118串"=0.0, "第119串"=0.0, "第120串"=0.0, "第一串 2"=0.0, "第一串 4"=0.0, "第一串 6"=0.0, "第一串 8"=0.0, "第一串 10"=0.0, "第一串 12"=0.0, "第一串 14"=0.0, "第一串 16"=0.0, "第一串 18"=0.0, "第一串 20"=0.0, "第一串 22"=0.0, "第一串 24"=0.0}, "1 28"={"第121串"=0.0, "第122串"=0.0, "第123串"=0.0, "第124串"=0.0, "第125串"=0.0, "第126串"=0.0, "第127串"=0.0, "第128串"=0.0, "第129串"=0.0, "第130串"=0.0, "第131串"=0.0, "第132串"=0.0, "第一串 2"=0.0, "第一串 4"=0.0, "第一串 6"=0.0, "第一串 8"=0.0, "第一串 10"=0.0, "第一串 12"=0.0, "第一串 14"=0.0, "第一串 16"=0.0, "第一串 18"=0.0, "第一串 20"=0.0, "第一串 22"=0.0, "第一串 24"=0.0}, "1 29"={"第133串"=0.0, "第134串"=0.0, "第135串"=0.0, "第136串"=0.0, "第137串"=0.0, "第138串"=0.0, "第139串"=0.0, "第140串"=0.0, "第141串"=0.0, "第142串"=0.0, "第143串"=0.0, "第144串"=0.0, "第一串 2"=0.0, "第一串 4"=0.0, "第一串 6"=0.0, "第一串 8"=0.0, "第一串 10"=0.0, "第一串 12"=0.0, "第一串 14"=0.0, "第一串 16"=0.0, "第一串 18"=0.0, "第一串 20"=0.0, "第一串 22"=0.0, "第一串 24"=0.0}, "1 30"={"第145串"=0.0, "第146串"=0.0, "第147串"=0.0, "第148串"=0.0, "第149串"=0.0, "第150串"=0.0, "第151串"=0.0, "第152串"=0.0, "第153串"=0.0, "第154串"=0.0, "第155串"=0.0, "第156串"=0.0, "第一串 2"=0.0, "第一串 4"=0.0, "第一串 6"=0.0, "第一串 8"=0.0, "第一串 10"=0.0, "第一串 12"=0.0, "第一串 14"=0.0, "第一串 16"=0.0, "第一串 18"=0.0, "第一串 20"=0.0, "第一串 22"=0.0, "第一串 24"=0.0}, "1 31"={"第157串"=0.0, "第158串"=0.0, "第159串"=0.0, "第160串"=0.0, "第161串"=0.0, "第162串"=0.0, "第163串"=0.0, "第164串"=0.0, "第165串"=0.0, "第166串"=0.0, "第167串"=0.0, "第168串"=0.0, "第一串 2"=0.0, "第一串 4"=0.0, "第一串 6"=0.0, "第一串 8"=0.0, "第一串 10"=0.0, "第一串 12"=0.0, "第一串 14"=0.0, "第一串 16"=0.0, "第一串 18"=0.0, "第一串 20"=0.0, "第一串 22"=0.0, "第一串 24"=0.0}, "1 32"={"第169串"=0.0, "第170串"=0.0, "第171串"=0.0, "第172串"=0.0, "第173串"=0.0, "第174串"=0.0, "第175串"=0.0, "第176串"=0.0, "第177串"=0.0, "第178串"=0.0, "第179串"=0.0, "第180串"=0.0, "第一串 2"=0.0, "第一串 4"=0.0, "第一串 6"=0.0, "第一串 8"=0.0, "第一串 10"=0.0, "第一串 12"=0.0, "第一串 14"=0.0, "第一串 16"=0.0, "第一串 18"=0.0, "第一串 20"=0.0, "第一串 22"=0.0, "第一串 24"=0.0}, "1 33"={"第181串"=0.0, "第182串"=0.0, "第183串"=0.0, "第184串"=0.0, "第185串"=0.0, "第186串"=0.0, "第187串"=0.0, "第188串"=0.0, "第189串"=0.0, "第190串"=0.0, "第191串"=0.0, "第192串"=0.0, "第一串 2"=0.0, "第一串 4"=0.0, "第一串 6"=0.0, "第一串 8"=0.0, "第一串 10"=0.0, "第一串 12"=0.0, "第一串 14"=0.0, "第一串 16"=0.0, "第一串 18"=0.0, "第一串 20"=0.0, "第一串 22"=0.0, "第一串 24"=0.0}, "1 16"={"充电1"=13816530, "充电1"=13816530, "充电1"=13816530, "充电1"=13816530, "充电1"=13816530, "充电1"=13816530, "充电1"=13816530, "充电1"=13816530, "充电1"=13816530, "充电1"=13816530, "充电1"=13816530, "充电1"=13816530}, "1 44"={"充电1"=13816530, "充电1"=13816530, "充电1"=13816530, "充电1"=13816530, "充电1"=13816530, "充电1"=13816530, "充电1"=13816530, "充电1"=13816530, "充电1"=13816530, "充电1"=13816530, "充电1"=13816530, "充电1"=13816530}, "1 36"={"充电1"=13816530, "充电1"=13816530, "充电1"=13816530, "充电1"=13816530, "充电1"=13816530, "充电1"=13816530, "充电1"=13816530, "充电1"=13816530, "充电1"=13816530, "充电1"=13816530, "充电1"=13816530, "充电1"=13816530}, "1 47"={"充电1"=13816530, "充电1"=13816530, "充电1"=13816530, "充电1"=13816530, "充电1"=13816530, "充电1"=13816530, "充电1"=13816530, "充电1"=13816530, "充电1"=13816530, "充电1"=13816530, "充电1"=13816530, "充电1"=13816530}, "1 19"={"充电1"=13816530, "充电1"=13816530, "充电1"=13816530, "充电1"=13816530, "充电1"=13816530, "充电1"=13816530, "充电1"=13816530, "充电1"=13816530, "充电1"=13816530, "充电1"=13816530, "充电1"=13816530, "充电1"=13816530}, "1 38"={"充电1"=13816530, "充电1"=13816530, "充电1"=13816530, "充电1"=13816530, "充电1"=13816530, "充电1"=13816530, "充电1"=13816530, "充电1"=13816530, "充电1"=13816530, "充电1"=13816530, "充电1"=13816530, "充电1"=13816530}, "1 41"={"充电1"=13816530, "充电1"=13816530, "充电1"=13816530, "充电1"=13816530, "充电1"=13816530, "充电1"=13816530, "充电1"=13816530, "充电1"=13816530, "充电1"=13816530, "充电1"=13816530, "充电1"=13816530, "充电1"=13816530}, "1 50"={"充电1"=13816530, "充电1"=13816530, "充电1"=13816530, "充电1"=13816530, "充电1"=13816530, "充电1"=13816530, "充电1"=13816530, "充电1"=13816530, "充电1"=13816530, "充电1"=13816530, "充电1"=13816530, "充电1"=13816530}, "1 15"={"充电1"=13816530, "充电1"=13816530, "充电1"=13816530, "充电1"=13816530, "充电1"=13816530, "充电1"=13816530, "充电1"=13816530, "充电1"=13816530, "充电1"=13816530, "充电1"=13816530, "充电1"=13816530, "充电1"=13816530}, "1 43"={"充电1"=13816530, "充电1"=13816530, "充电1"=13816530, "充电1"=13816530, "充电1"=13816530, "充电1"=13816530, "充电1"=13816530, "充电1"=13816530, "充电1"=13816530, "充电1"=13816530, "充电1"=13816530, "充电1"=13816530}, "1 35"={"充电1"=13816530, "充电1"=13816530, "充电1"=13816530, "充电1"=13816530, "充电1"=13816530, "充电1"=13816530, "充电1"=13816530, "充电1"=13816530, "充电1"=13816530, "充电1"=13816530, "充电1"=13816530, "充电1"=13816530}, "1 46"={"充电1"=13816530, "充电1"=13816530, "充电1"=13816530, "充电1"=13816530, "充电1"=13816530, "充电1"=13816530, "充电1"=13816530, "充电1"=13816530, "充电1"=13816530, "充电1"=13816530, "充电1"=13816530, "充电1"=13816530}, "1 18"={"充电1"=13816530, "充电1"=13816530, "充电1"=13816530, "充电1"=13816530, "充电1"=13816530, "充电1"=13816530, "充电1"=13816530, "充电1"=13816530, "充电1"=13816530, "充电1"=13816530, "充电1"=13816530, "充电1"=13816530}, "1 37"={"充电1"=13816530, "充电1"=13816530, "充电1"=13816530, "充电1"=13816530, "充电1"=13816530, "充电1"=13816530, "充电1"=13816530, "充电1"=13816530, "充电1"=13816530, "充电1"=13816530, "充电1"=13816530, "充电1"=13816530}, "1 40"={"充电1"=13816530, "充电1"=13816530, "充电1"=13816530, "充电1"=13816530, "充电1"=13816530, "充电1"=13816530, "充电1"=13816530, "充电1"=13816530, "充电1"=13816530, "充电1"=13816530, "充电1"=13816530, "充电1"=13816530}, "1 49"={"充电1"=13816530, "充电1"=13816530, "充电1"=13816530, "充电1"=13816530, "充电1"=13816530, "充电1"=13816530, "充电1"=13816530, "充电1"=13816530, "充电1"=13816530, "充电1"=13816530, "充电1"=13816530, "充电1"=13816530}, "1 14"={"均衡故障"=15, "均衡故障 2"=0.0, "均衡故障 3"=0.0, "均衡故障 4"=0.0, "均衡故障 5"=0.0, "均衡故障 6"=0.0, "均衡故障 7"=0.0, "均衡故障 8"=0.0, "均衡故障 9"=0.0, "均衡故障 10"=0.0, "均衡故障 11"=0.0, "均衡故障 12"=0.0}, "1 42"={"均衡故障"=15, "均衡故障 2"=0.0, "均衡故障 3"=0.0, "均衡故障 4"=0.0, "均衡故障 5"=0.0, "均衡故障 6"=0.0, "均衡故障 7"=0.0, "均衡故障 8"=0.0, "均衡故障 9"=0.0, "均衡故障 10"=0.0, "均衡故障 11"=0.0, "均衡故障 12"=0.0}, "1 34"={"均衡故障"=15, "均衡故障 2"=0.0, "均衡故障 3"=0.0, "均衡故障 4"=0.0, "均衡故障 5"=0.0, "均衡故障 6"=0.0, "均衡故障 7"=0.0, "均衡故障 8"=0.0, "均衡故障 9"=0.0, "均衡故障 10"=0.0, "均衡故障 11"=0.0, "均衡故障 12"=0.0}, "1 45"={"均衡故障"=15, "均衡故障 2"=0.0, "均衡故障 3"=0.0, "均衡故障 4"=0.0, "均衡故障 5"=0.0, "均衡故障 6"=0.0, "均衡故障 7"=0.0, "均衡故障 8"=0.0, "均衡故障 9"=0.0, "均衡故障 10"=0.0, "均衡故障 11"=0.0, "均衡故障 12"=0.0}, "1 17"={"均衡故障"=15, "均衡故障 2"=0.0, "均衡故障 3"=0.0, "均衡故障 4"=0.0, "均衡故障 5"=0.0, "均衡故障 6"=0.0, "均衡故障 7"=0.0, "均衡故障 8"=0.0, "均衡故障 9"=0.0, "均衡故障 10"=0.0, "均衡故障 11"=0.0, "均衡故障 12"=0.0}, "1 20"={"均衡故障"=15, "均衡故障 2"=0.0, "均衡故障 3"=0.0, "均衡故障 4"=0.0, "均衡故障 5"=0.0, "均衡故障 6"=0.0, "均衡故障 7"=0.0, "均衡故障 8"=0.0, "均衡故障 9"=0.0, "均衡故障 10"=0.0, "均衡故障 11"=0.0, "均衡故障 12"=0.0}, "1 39"={"均衡故障"=15, "均衡故障 2"=0.0, "均衡故障 3"=0.0, "均衡故障 4"=0.0, "均衡故障 5"=0.0, "均衡故障 6"=0.0, "均衡故障 7"=0.0, "均衡故障 8"=0.0, "均衡故障 9"=0.0, "均衡故障 10"=0.0, "均衡故障 11"=0.0, "均衡故障 12"=0.0}, "1 48"={"均衡故障"=15, "均衡故障 2"=0.0, "均衡故障 3"=0.0, "均衡故障 4"=0.0, "均衡故障 5"=0.0, "均衡故障 6"=0.0, "均衡故障 7"=0.0, "均衡故障 8"=0.0, "均衡故障 9"=0.0, "均衡故障 10"=0.0, "均衡故障 11"=0.0, "均衡故障 12"=0.0}} {"1 33"."第192串" format="%.3f"; "1 33"."第191串" format="%.3f"; "1 33"."第190串" format="%.3f"; "1 33"."第189串" format="%.3f"; "1 33"."第188串" format="%.3f"; "1 33"."第187串" format="%.3f"; "1 33"."第186串" format="%.3f"; "1 33"."第185串" format="%.3f"; "1 33"."第184串" format="%.3f"; "1 33"."第183串" format="%.3f"; "1 33"."第182串" format="%.3f"; "1 33"."第181串" format="%.3f"; "1 32"."第180串" format="%.3f"; "1 32"."第179串" format="%.3f"; "1 32"."第178串" format="%.3f"; "1 32"."第177串" format="%.3f"; "1 32"."第176串" format="%.3f"; "1 32"."第175串" format="%.3f"; "1 32"."第174串" format="%.3f"; "1 32"."第173串" format="%.3f"; "1 32"."第172串" format="%.3f"; "1 32"."第171串" format="%.3f"; "1 32"."第170串" format="%.3f"; "1 32"."第169串" format="%.3f"; "1 31"."第168串" format="%.3f"; "1 31"."第167串" format="%.3f"; "1 31"."第166串" format="%.3f"; "1 31"."第165串" format="%.3f"; "1 31"."第164串" format="%.3f"; "1 31"."第163串" format="%.3f"; "1 31"."第162串" format="%.3f"; "1 31"."第161串" format="%.3f"; "1 31"."第160串" format="%.3f"; "1 31"."第159串" format="%.3f"; "1 31"."第158串" format="%.3f"; "1 31"."第157串" format="%.3f"; "1 30"."第156串" format="%.3f"; "1 30"."第155串" format="%.3f"; "1 30"."第154串" format="%.3f"; "1 30"."第153串" format="%.3f"; "1 30"."第152串" format="%.3f"; "1 30"."第151串" format="%.3f"; "1 30"."第150串" format="%.3f"; "1 30"."第149串" format="%.3f"; "1 30"."第148串" format="%.3f"; "1 30"."第147串" format="%.3f"; "1 30"."第146串" format="%.3f"; "1 30"."第145串" format="%.3f"; "1 29"."第144串" format="%.3f"; "1 29"."第143串" format="%.3f"; "1 29"."第142串" format="%.3f"; "1 29"."第141串" format="%.3f"; "1 29"."第140串" format="%.3f"; "1 29"."第139串" format="%.3f"; "1 29"."第138串" format="%.3f"; "1 29"."第137串" format="%.3f"; "1 29"."第136串" format="%.3f"; "1 29"."第135串" format="%.3f"; "1 29"."第134串" format="%.3f"; "1 29"."第133串" format="%.3f"; "1 28"."第132串" format="%.3f"; "1 28"."第131串" format="%.3f"; "1 28"."第130串" format="%.3f"; "1 28"."第129串" format="%.3f"; "1 28"."第128串" format="%.3f"; "1 28"."第127串" format="%.3f"; "1 28"."第126串" format="%.3f"; "1 28"."第125串" format="%.3f"; "1 28"."第124串" format="%.3f"; "1 28"."第123串" format="%.3f"; "1 28"."第122串" format="%.3f"; "1 28"."第121串" format="%.3f"; "1 27"."第120串" format="%.3f"; "1 27"."第119串" format="%.3f"; "1 27"."第118串" format="%.3f"; "1 27"."第117串" format="%.3f"; "1 27"."第116串" format="%.3f"; "1 27"."第115串" format="%.3f"; "1 27"."第114串" format="%.3f"; "1 27"."第113串" format="%.3f"; "1 27"."第112串" format="%.3f"; "1 27"."第111串" format="%.3f"; "1 27"."第110串" format="%.3f"; "1 27"."第109串" format="%.3f"; "1 26"."第一串 24" format="%#.2f"; "1 26"."第108串" format="%.3f"; "1 26"."第一串 22" format="%#.2f"; "1 26"."第107串" format="%.3f"; "1 26"."第一串 20" format="%#.2f"; "1 26"."第106串" format="%.3f"; "1 26"."第一串 18" format="%#.2f"; "1 26"."第105串" format="%.3f"; "1 26"."第一串 16" format="%#.2f"; "1 26"."第104串" format="%.3f"; "1 26"."第一串 14" format="%#.2f"; "1 26"."第103串" format="%.3f"; "1 26"."第一串 12" format="%#.2f"; "1 26"."第102串" format="%.3f"; "1 26"."第一串 10" format="%#.2f"; "1 26"."第101串" format="%.3f"; "1 26"."第一串 8" format="%#.2f"; "1 26"."第100串" format="%.3f"; "1 26"."第一串 6" format="%#.2f"; "1 26"."第99串" format="%.3f"; "1 26"."第一串 4" format="%#.2f"; "1 26"."第98串" format="%.3f"; "1 26"."第一串 2" format="%#.2f"; "1 26"."第97串" format="%.3f"}
  out "3":T6={"1 18"={"第193串"=0.0, "第194串"=0.0, "第195串"=0.0, "第196串"=0.0, "第197串"=0.0, "第198串"=0.0, "第199串"=0.0, "第200串"=0.0, "第201串"=0.0, "第202串"=0.0, "第203串"=0.0, "第204串"=0.0, "第一串 2"=0.0, "第一串 4"=0.0, "第一串 6"=0.0, "第一串 8"=0.0, "第一串 10"=0.0, "第一串 12"=0.0, "第一串 14"=0.0, "第一串 16"=0.0, "第一串 18"=0.0, "第一串 20"=0.0, "第一串 22"=0.0, "第一串 24"=0.0}, "1 19"={"第205串"=0.0, "第206串"=0.0, "第207串"=0.0, "第208串"=0.0, "第209串"=0.0, "第210串"=0.0, "第211串"=0.0, "第212串"=0.0, "第213串"=0.0, "第214串"=0.0, "第215串"=0.0, "第216串"=0.0, "第一串 2"=0.0, "第一串 4"=0.0, "第一串 6"=0.0, "第一串 8"=0.0, "第一串 10"=0.0, "第一串 12"=0.0, "第一串 14"=0.0, "第一串 16"=0.0, "第一串 18"=0.0, "第一串 20"=0.0, "第一串 22"=0.0, "第一串 24"=0.0}, "1 20"={"第217串"=0.0, "第218串"=0.0, "第219串"=0.0, "第220串"=0.0, "第221串"=0.0, "第222串"=0.0, "第223串"=0.0, "第224串"=0.0, "第225串"=0.0, "第226串"=0.0, "第227串"=0.0, "第228串"=0.0, "第一串 2"=0.0, "第一串 4"=0.0, "第一串 6"=0.0, "第一串 8"=0.0, "第一串 10"=0.0, "第一串 12"=0.0, "第一串 14"=0.0, "第一串 16"=0.0, "第一串 18"=0.0, "第一串 20"=0.0, "第一串 22"=0.0, "第一串 24"=0.0}, "1 21"={"第229串"=0.0, "第230串"=0.0, "第231串"=0.0, "第232串"=0.0, "第233串"=0.0, "第234串"=0.0, "第235串"=0.0, "第236串"=0.0, "第237串"=0.0, "第238串"=0.0, "第239串"=0.0, "第240串"=0.0, "第一串 2"=0.0, "第一串 4"=0.0, "第一串 6"=0.0, "第一串 8"=0.0, "第一串 10"=0.0, "第一串 12"=0.0, "第一串 14"=0.0, "第一串 16"=0.0, "第一串 18"=0.0, "第一串 20"=0.0, "第一串 22"=0.0, "第一串 24"=0.0}, "1 22"={"第241串"=0.0, "第242串"=0.0, "第243串"=0.0, "第244串"=0.0, "第245串"=0.0, "第246串"=0.0, "第247串"=0.0, "第248串"=0.0, "第249串"=0.0, "第250串"=0.0, "第251串"=0.0, "第252串"=0.0, "第一串 2"=0.0, "第一串 4"=0.0, "第一串 6"=0.0, "第一串 8"=0.0, "第一串 10"=0.0, "第一串 12"=0.0, "第一串 14"=0.0, "第一串 16"=0.0, "第一串 18"=0.0, "第一串 20"=0.0, "第一串 22"=0.0, "第一串 24"=0.0}, "1 23"={"第253串"=0.0, "第254串"=0.0, "第255串"=0.0, "第256串"=0.0, "第257串"=0.0, "第258串"=0.0, "第259串"=0.0, "第260串"=0.0, "第261串"=0.0, "第262串"=0.0, "第263串"=0.0, "第264串"=0.0, "第一串 2"=0.0, "第一串 4"=0.0, "第一串 6"=0.0, "第一串 8"=0.0, "第一串 10"=0.0, "第一串 12"=0.0, "第一串 14"=0.0, "第一串 16"=0.0, "第一串 18"=0.0, "第一串 20"=0.0, "第一串 22"=0.0, "第一串 24"=0.0}, "1 24"={"第265串"=0.0, "第266串"=0.0, "第267串"=0.0, "第268串"=0.0, "第269串"=0.0, "第270串"=0.0, "第271串"=0.0, "第272串"=0.0, "第273串"=0.0, "第274串"=0.0, "第275串"=0.0, "第276串"=0.0, "第一串 2"=0.0, "第一串 4"=0.0, "第一串 6"=0.0, "第一串 8"=0.0, "第一串 10"=0.0, "第一串 12"=0.0, "第一串 14"=0.0, "第一串 16"=0.0, "第一串 18"=0.0, "第一串 20"=0.0, "第一串 22"=0.0, "第一串 24"=0.0}, "1 25"={"第277串"=0.0, "第278串"=0.0, "第279串"=0.0, "第280串"=0.0, "第281串"=0.0, "第282串"=0.0, "第283串"=0.0, "第284串"=0.0, "第285串"=0.0, "第286串"=0.0, "第287串"=0.0, "第288串"=0.0, "第一串 2"=0.0, "第一串 4"=0.0, "第一串 6"=0.0, "第一串 8"=0.0, "第一串 10"=0.0, "第一串 12"=0.0, "第一串 14"=0.0, "第一串 16"=0.0, "第一串 18"=0.0, "第一串 20"=0.0, "第一串 22"=0.0, "第一串 24"=0.0}, "1 12"={"充电1"=13816530, "充电1"=13816530, "充电1"=13816530, "充电1"=13816530, "充电1"=13816530, "充电1"=13816530, "充电1"=13816530, "充电1"=13816530, "充电1"=13816530, "充电1"=13816530, "充电1"=13816530, "充电1"=13816530}, "1 39"={"充电1"=13816530, "充电1"=13816530, "充电1"=13816530, "充电1"=13816530, "充电1"=13816530, "充电1"=13816530, "充电1"=13816530, "充电1"=13816530, "充电1"=13816530, "充电1"=13816530, "充电1"=13816530, "充电1"=13816530}, "1 28"={"充电1"=13816530, "充电1"=13816530, "充电1"=13816530, "充电1"=13816530, "充电1"=13816530, "充电1"=13816530, "充电1"=13816530, "充电1"=13816530, "充电1"=13816530, "充电1"=13816530, "充电1"=13816530, "充电1"=13816530}, "1 42"={"充电1"=13816530, "充电1"=13816530, "充电1"=13816530, "充电1"=13816530, "充电1"=13816530, "充电1"=13816530, "充电1"=13816530, "充电1"=13816530, "充电1"=13816530, "充电1"=13816530, "充电1"=13816530, "充电1"=13816530}, "1 16"={"充电1"=13816530, "充电1"=13816530, "充电1"=13816530, "充电1"=13816530, "充电1"=13816530, "充电1"=13816530, "充电1"=13816530, "充电1"=13816530, "充电1"=13816530, "充电1"=13816530, "充电1"=13816530, "充电1"=13816530}, "1 30"={"充电1"=13816530, "充电1"=13816530, "充电1"=13816530, "充电1"=13816530, "充电1"=13816530, "充电1"=13816530, "充电1"=13816530, "充电1"=13816530, "充电1"=13816530, "充电1"=13816530, "充电1"=13816530, "充电1"=13816530}, "1 33"={"充电1"=13816530, "充电1"=13816530, "充电1"=13816530, "充电1"=13816530, "充电1"=13816530, "充电1"=13816530, "充电1"=13816530, "充电1"=13816530, "充电1"=13816530, "充电1"=13816530, "充电1"=13816530, "充电1"=13816530}, "1 36"={"充电1"=13816530, "充电1"=13816530, "充电1"=13816530, "充电1"=13816530, "充电1"=13816530, "充电1"=13816530, "充电1"=13816530, "充电1"=13816530, "充电1"=13816530, "充电1"=13816530, "充电1"=13816530, "充电1"=13816530}, "1 11"={"充电1"=13816530, "充电1"=13816530, "充电1"=13816530, "充电1"=13816530, "充电1"=13816530, "充电1"=13816530, "充电1"=13816530, "充电1"=13816530, "充电1"=13816530, "充电1"=13816530, "充电1"=13816530, "充电1"=13816530}, "1 38"={"充电1"=13816530, "充电1"=13816530, "充电1"=13816530, "充电1"=13816530, "充电1"=13816530, "充电1"=13816530, "充电1"=13816530, "充电1"=13816530, "充电1"=13816530, "充电1"=13816530, "充电1"=13816530, "充电1"=13816530}, "1 27"={"充电1"=13816530, "充电1"=13816530, "充电1"=13816530, "充电1"=13816530, "充电1"=13816530, "充电1"=13816530, "充电1"=13816530, "充电1"=13816530, "充电1"=13816530, "充电1"=13816530, "充电1"=13816530, "充电1"=13816530}, "1 41"={"充电1"=13816530, "充电1"=13816530, "充电1"=13816530, "充电1"=13816530, "充电1"=13816530, "充电1"=13816530, "充电1"=13816530, "充电1"=13816530, "充电1"=13816530, "充电1"=13816530, "充电1"=13816530, "充电1"=13816530}, "1 15"={"充电1"=13816530, "充电1"=13816530, "充电1"=13816530, "充电1"=13816530, "充电1"=13816530, "充电1"=13816530, "充电1"=13816530, "充电1"=13816530, "充电1"=13816530, "充电1"=13816530, "充电1"=13816530, "充电1"=13816530}, "1 29"={"充电1"=13816530, "充电1"=13816530, "充电1"=13816530, "充电1"=13816530, "充电1"=13816530, "充电1"=13816530, "充电1"=13816530, "充电1"=13816530, "充电1"=13816530, "充电1"=13816530, "充电1"=13816530, "充电1"=13816530}, "1 32"={"充电1"=13816530, "充电1"=13816530, "充电1"=13816530, "充电1"=13816530, "充电1"=13816530, "充电1"=13816530, "充电1"=13816530, "充电1"=13816530, "充电1"=13816530, "充电1"=13816530, "充电1"=13816530, "充电1"=13816530}, "1 35"={"充电1"=13816530, "充电1"=13816530, "充电1"=13816530, "充电1"=13816530, "充电1"=13816530, "充电1"=13816530, "充电1"=13816530, "充电1"=13816530, "充电1"=13816530, "充电1"=13816530, "充电1"=13816530, "充电1"=13816530}, "1 13"={"均衡故障"=0, "均衡故障 2"=0.0, "均衡故障 3"=0.0, "均衡故障 4"=0.0, "均衡故障 5"=0.0, "均衡故障 6"=0.0, "均衡故障 7"=0.0, "均衡故障 8"=0.0, "均衡故障 9"=0.0, "均衡故障 10"=0.0, "均衡故障 11"=0.0, "均衡故障 12"=0.0}, "1 37"={"均衡故障"=0, "均衡故障 2"=0.0, "均衡故障 3"=0.0, "均衡故障 4"=0.0, "均衡故障 5"=0.0, "均衡故障 6"=0.0, "均衡故障 7"=0.0, "均衡故障 8"=0.0, "均衡故障 9"=0.0, "均衡故障 10"=0.0, "均衡故障 11"=0.0, "均衡故障 12"=0.0}, "1 26"={"均衡故障"=0, "均衡故障 2"=0.0, "均衡故障 3"=0.0, "均衡故障 4"=0.0, "均衡故障 5"=0.0, "均衡故障 6"=0.0, "均衡故障 7"=0.0, "均衡故障 8"=0.0, "均衡故障 9"=0.0, "均衡故障 10"=0.0, "均衡故障 11"=0.0, "均衡故障 12"=0.0}, "1 40"={"均衡故障"=0, "均衡故障 2"=0.0, "均衡故障 3"=0.0, "均衡故障 4"=0.0, "均衡故障 5"=0.0, "均衡故障 6"=0.0, "均衡故障 7"=0.0, "均衡故障 8"=0.0, "均衡故障 9"=0.0, "均衡故障 10"=0.0, "均衡故障 11"=0.0, "均衡故障 12"=0.0}, "1 14"={"均衡故障"=0, "均衡故障 2"=0.0, "均衡故障 3"=0.0, "均衡故障 4"=0.0, "均衡故障 5"=0.0, "均衡故障 6"=0.0, "均衡故障 7"=0.0, "均衡故障 8"=0.0, "均衡故障 9"=0.0, "均衡故障 10"=0.0, "均衡故障 11"=0.0, "均衡故障 12"=0.0}, "1 17"={"均衡故障"=0, "均衡故障 2"=0.0, "均衡故障 3"=0.0, "均衡故障 4"=0.0, "均衡故障 5"=0.0, "均衡故障 6"=0.0, "均衡故障 7"=0.0, "均衡故障 8"=0.0, "均衡故障 9"=0.0, "均衡故障 10"=0.0, "均衡故障 11"=0.0, "均衡故障 12"=0.0}, "1 31"={"均衡故障"=0, "均衡故障 2"=0.0, "均衡故障 3"=0.0, "均衡故障 4"=0.0, "均衡故障 5"=0.0, "均衡故障 6"=0.0, "均衡故障 7"=0.0, "均衡故障 8"=0.0, "均衡故障 9"=0.0, "均衡故障 10"=0.0, "均衡故障 11"=0.0, "均衡故障 12"=0.0}, "1 34"={"均衡故障"=0, "均衡故障 2"=0.0, "均衡故障 3"=0.0, "均衡故障 4"=0.0, "均衡故障 5"=0.0, "均衡故障 6"=0.0, "均衡故障 7"=0.0, "均衡故障 8"=0.0, "均衡故障 9"=0.0, "均衡故障 10"=0.0, "均衡故障 11"=0.0, "均衡故障 12"=0.0}} {"1 25"."第288串" format="%.3f"; "1 25"."第287串" format="%.3f"; "1 25"."第286串" format="%.3f"; "1 25"."第285串" format="%.3f"; "1 25"."第284串" format="%.3f"; "1 25"."第283串" format="%.3f"; "1 25"."第282串" format="%.3f"; "1 25"."第281串" format="%.3f"; "1 25"."第280串" format="%.3f"; "1 25"."第279串" format="%.3f"; "1 25"."第278串" format="%.3f"; "1 25"."第277串" format="%.3f"; "1 24"."第276串" format="%.3f"; "1 24"."第275串" format="%.3f"; "1 24"."第274串" format="%.3f"; "1 24"."第273串" format="%.3f"; "1 24"."第272串" format="%.3f"; "1 24"."第271串" format="%.3f"; "1 24"."第270串" format="%.3f"; "1 24"."第269串" format="%.3f"; "1 24"."第268串" format="%.3f"; "1 24"."第267串" format="%.3f"; "1 24"."第266串" format="%.3f"; "1 24"."第265串" format="%.3f"; "1 23"."第264串" format="%.3f"; "1 23"."第263串" format="%.3f"; "1 23"."第262串" format="%.3f"; "1 23"."第261串" format="%.3f"; "1 23"."第260串" format="%.3f"; "1 23"."第259串" format="%.3f"; "1 23"."第258串" format="%.3f"; "1 23"."第257串" format="%.3f"; "1 23"."第256串" format="%.3f"; "1 23"."第255串" format="%.3f"; "1 23"."第254串" format="%.3f"; "1 23"."第253串" format="%.3f"; "1 22"."第252串" format="%.3f"; "1 22"."第251串" format="%.3f"; "1 22"."第250串" format="%.3f"; "1 22"."第249串" format="%.3f"; "1 22"."第248串" format="%.3f"; "1 22"."第247串" format="%.3f"; "1 22"."第246串" format="%.3f"; "1 22"."第245串" format="%.3f"; "1 22"."第244串" format="%.3f"; "1 22"."第243串" format="%.3f"; "1 22"."第242串" format="%.3f"; "1 22"."第241串" format="%.3f"; "1 21"."第240串" format="%.3f"; "1 21"."第239串" format="%.3f"; "1 21"."第238串" format="%.3f"; "1 21"."第237串" format="%.3f"; "1 21"."第236串" format="%.3f"; "1 21"."第235串" format="%.3f"; "1 21"."第234串" format="%.3f"; "1 21"."第233串" format="%.3f"; "1 21"."第232串" format="%.3f"; "1 21"."第231串" format="%.3f"; "1 21"."第230串" format="%.3f"; "1 21"."第229串" format="%.3f"; "1 20"."第228串" format="%.3f"; "1 20"."第227串" format="%.3f"; "1 20"."第226串" format="%.3f"; "1 20"."第225串" format="%.3f"; "1 20"."第224串" format="%.3f"; "1 20"."第223串" format="%.3f"; "1 20"."第222串" format="%.3f"; "1 20"."第221串" format="%.3f"; "1 20"."第220串" format="%.3f"; "1 20"."第219串" format="%.3f"; "1 20"."第218串" format="%.3f"; "1 20"."第217串" format="%.3f"; "1 19"."第216串" format="%.3f"; "1 19"."第215串" format="%.3f"; "1 19"."第214串" format="%.3f"; "1 19"."第213串" format="%.3f"; "1 19"."第212串" format="%.3f"; "1 19"."第211串" format="%.3f"; "1 19"."第210串" format="%.3f"; "1 19"."第209串" format="%.3f"; "1 19"."第208串" format="%.3f"; "1 19"."第207串" format="%.3f"; "1 19"."第206串" format="%.3f"; "1 19"."第205串" format="%.3f"; "1 18"."第一串 24" format="%#.2f"; "1 18"."第204串" format="%.3f"; "1 18"."第一串 22" format="%#.2f"; "1 18"."第203串" format="%.3f"; "1 18"."第一串 20" format="%#.2f"; "1 18"."第202串" format="%.3f"; "1 18"."第一串 18" format="%#.2f"; "1 18"."第201串" format="%.3f"; "1 18"."第一串 16" format="%#.2f"; "1 18"."第200串" format="%.3f"; "1 18"."第一串 14" format="%#.2f"; "1 18"."第199串" format="%.3f"; "1 18"."第一串 12" format="%#.2f"; "1 18"."第198串" format="%.3f"; "1 18"."第一串 10" format="%#.2f"; "1 18"."第197串" format="%.3f"; "1 18"."第一串 8" format="%#.2f"; "1 18"."第196串" format="%.3f"; "1 18"."第一串 6" format="%#.2f"; "1 18"."第195串" format="%.3f"; "1 18"."第一串 4" format="%#.2f"; "1 18"."第194串" format="%.3f"; "1 18"."第一串 2" format="%#.2f"; "1 18"."第193串" format="%.3f"}
  out "1 5":T7 {"第一串 24" format="%#.2f"; "第300串" format="%.3f"; "第一串 22" format="%#.2f"; "第299串" format="%.3f"; "第一串 20" format="%#.2f"; "第298串" format="%.3f"; "第一串 18" format="%#.2f"; "第297串" format="%.3f"; "第一串 16" format="%#.2f"; "第296串" format="%.3f"; "第一串 14" format="%#.2f"; "第295串" format="%.3f"; "第一串 12" format="%#.2f"; "第294串" format="%.3f"; "第一串 10" format="%#.2f"; "第293串" format="%.3f"; "第一串 8" format="%#.2f"; "第292串" format="%.3f"; "第一串 6" format="%#.2f"; "第291串" format="%.3f"; "第一串 4" format="%#.2f"; "第290串" format="%.3f"; "第一串 2" format="%#.2f"; "第289串" format="%.3f"}
  out "1 13":T8
  out "放电均衡":T9={"充电1"=13816530, "充电1"=13816530, "充电1"=13816530, "充电1"=13816530, "充电1"=13816530, "充电1"=13816530, "充电1"=13816530, "充电1"=13816530, "充电1"=13816530, "充电1"=13816530, "充电1"=13816530, "充电1"=13816530}
  out "充电均衡":T9={"充电1"=13816530, "充电1"=13816530, "充电1"=13816530, "充电1"=13816530, "充电1"=13816530, "充电1"=13816530, "充电1"=13816530, "充电1"=13816530, "充电1"=13816530, "充电1"=13816530, "充电1"=13816530, "充电1"=13816530}
  out "放电均衡":u32(colorbox)=6618880
  out "充电均衡":u32(colorbox)=16860
  in  "布尔":bool caption="判定"
  in  "故障信息选择按键 3":enum32{"单选选项2", "单选选项2 2", "单选选项2 3", "单选选项1"}(radio)=enum."单选选项1"
  out "电压选择 2":enum32{"1-96", "97-192", "193-288", "289-300"}(tab)
  out "4":T10 {"1 102"."第一串 24" format="%#.2f"; "1 102"."第12串" format="%#.2f"; "1 102"."第一串 22" format="%#.2f"; "1 102"."第11串" format="%#.2f"; "1 102"."第一串 20" format="%#.2f"; "1 102"."第10串" format="%#.2f"; "1 102"."第一串 18" format="%#.2f"; "1 102"."第9串" format="%#.2f"; "1 102"."第一串 16" format="%#.2f"; "1 102"."第8串" format="%#.2f"; "1 102"."第一串 14" format="%#.2f"; "1 102"."第7串" format="%#.2f"; "1 102"."第一串 12" format="%#.2f"; "1 102"."第6串" format="%#.2f"; "1 102"."第一串 10" format="%#.2f"; "1 102"."第5串" format="%#.2f"; "1 102"."第一串 8" format="%#.2f"; "1 102"."第4串" format="%#.2f"; "1 102"."第一串 6" format="%#.2f"; "1 102"."第3串" format="%#.2f"; "1 102"."第一串 4" format="%#.2f"; "1 102"."第2串" format="%#.2f"; "1 102"."第一串 2" format="%#.2f"; "1 102"."第1串" format="%#.2f"}
  out "5":T11 {"1 26"."第一串 24" format="%#.2f"; "1 26"."第108串" format="%#.2f"; "1 26"."第一串 22" format="%#.2f"; "1 26"."第107串" format="%#.2f"; "1 26"."第一串 20" format="%#.2f"; "1 26"."第106串" format="%#.2f"; "1 26"."第一串 18" format="%#.2f"; "1 26"."第105串" format="%#.2f"; "1 26"."第一串 16" format="%#.2f"; "1 26"."第104串" format="%#.2f"; "1 26"."第一串 14" format="%#.2f"; "1 26"."第103串" format="%#.2f"; "1 26"."第一串 12" format="%#.2f"; "1 26"."第102串" format="%#.2f"; "1 26"."第一串 10" format="%#.2f"; "1 26"."第101串" format="%#.2f"; "1 26"."第一串 8" format="%#.2f"; "1 26"."第100串" format="%#.2f"; "1 26"."第一串 6" format="%#.2f"; "1 26"."第99串" format="%#.2f"; "1 26"."第一串 4" format="%#.2f"; "1 26"."第98串" format="%#.2f"; "1 26"."第一串 2" format="%#.2f"; "1 26"."第97串" format="%#.2f"}
  out "6":T12 {"1 18"."第一串 24" format="%#.2f"; "1 18"."第204串" format="%#.2f"; "1 18"."第一串 22" format="%#.2f"; "1 18"."第203串" format="%#.2f"; "1 18"."第一串 20" format="%#.2f"; "1 18"."第202串" format="%#.2f"; "1 18"."第一串 18" format="%#.2f"; "1 18"."第201串" format="%#.2f"; "1 18"."第一串 16" format="%#.2f"; "1 18"."第200串" format="%#.2f"; "1 18"."第一串 14" format="%#.2f"; "1 18"."第199串" format="%#.2f"; "1 18"."第一串 12" format="%#.2f"; "1 18"."第198串" format="%#.2f"; "1 18"."第一串 10" format="%#.2f"; "1 18"."第197串" format="%#.2f"; "1 18"."第一串 8" format="%#.2f"; "1 18"."第196串" format="%#.2f"; "1 18"."第一串 6" format="%#.2f"; "1 18"."第195串" format="%#.2f"; "1 18"."第一串 4" format="%#.2f"; "1 18"."第194串" format="%#.2f"; "1 18"."第一串 2" format="%#.2f"; "1 18"."第193串" format="%#.2f"}
  out "1 6":T7 {"第一串 24" format="%#.2f"; "第300串" format="%#.2f"; "第一串 22" format="%#.2f"; "第299串" format="%#.2f"; "第一串 20" format="%#.2f"; "第298串" format="%#.2f"; "第一串 18" format="%#.2f"; "第297串" format="%#.2f"; "第一串 16" format="%#.2f"; "第296串" format="%#.2f"; "第一串 14" format="%#.2f"; "第295串" format="%#.2f"; "第一串 12" format="%#.2f"; "第294串" format="%#.2f"; "第一串 10" format="%#.2f"; "第293串" format="%#.2f"; "第一串 8" format="%#.2f"; "第292串" format="%#.2f"; "第一串 6" format="%#.2f"; "第291串" format="%#.2f"; "第一串 4" format="%#.2f"; "第290串" format="%#.2f"; "第一串 2" format="%#.2f"; "第289串" format="%#.2f"}
  in  "偏差":dbl=2.0 format="%#.0f"
  in  "基准":dbl=25.0 format="%#.0f"
  in  "布尔 2":bool caption="判定"
  in  "故障信息选择按键 4":enum32{"单选选项2", "单选选项2 2", "单选选项2 3", "单选选项1"}(radio)=enum."单选选项1"
  out "电压选择 3":enum32{"1-96", "97-192", "193-288", "289-300"}(tab)
  out "1 106":T13 {"1 102"."第一串 24" format="%#.2f"; "1 102"."第12串" format="%#.2f"; "1 102"."第一串 22" format="%#.2f"; "1 102"."第11串" format="%#.2f"; "1 102"."第一串 20" format="%#.2f"; "1 102"."第10串" format="%#.2f"; "1 102"."第一串 18" format="%#.2f"; "1 102"."第9串" format="%#.2f"; "1 102"."第一串 16" format="%#.2f"; "1 102"."第8串" format="%#.2f"; "1 102"."第一串 14" format="%#.2f"; "1 102"."第7串" format="%#.2f"; "1 102"."第一串 12" format="%#.2f"; "1 102"."第6串" format="%#.2f"; "1 102"."第一串 10" format="%#.2f"; "1 102"."第5串" format="%#.2f"; "1 102"."第一串 8" format="%#.2f"; "1 102"."第4串" format="%#.2f"; "1 102"."第一串 6" format="%#.2f"; "1 102"."第3串" format="%#.2f"; "1 102"."第一串 4" format="%#.2f"; "1 102"."第2串" format="%#.2f"; "1 102"."第一串 2" format="%#.2f"; "1 102"."第1串" format="%#.2f"}
  out "1 107":T11 {"1 26"."第一串 24" format="%#.2f"; "1 26"."第108串" format="%#.2f"; "1 26"."第一串 22" format="%#.2f"; "1 26"."第107串" format="%#.2f"; "1 26"."第一串 20" format="%#.2f"; "1 26"."第106串" format="%#.2f"; "1 26"."第一串 18" format="%#.2f"; "1 26"."第105串" format="%#.2f"; "1 26"."第一串 16" format="%#.2f"; "1 26"."第104串" format="%#.2f"; "1 26"."第一串 14" format="%#.2f"; "1 26"."第103串" format="%#.2f"; "1 26"."第一串 12" format="%#.2f"; "1 26"."第102串" format="%#.2f"; "1 26"."第一串 10" format="%#.2f"; "1 26"."第101串" format="%#.2f"; "1 26"."第一串 8" format="%#.2f"; "1 26"."第100串" format="%#.2f"; "1 26"."第一串 6" format="%#.2f"; "1 26"."第99串" format="%#.2f"; "1 26"."第一串 4" format="%#.2f"; "1 26"."第98串" format="%#.2f"; "1 26"."第一串 2" format="%#.2f"; "1 26"."第97串" format="%#.2f"}
  out "1 28":T12 {"1 18"."第一串 24" format="%#.2f"; "1 18"."第204串" format="%#.2f"; "1 18"."第一串 22" format="%#.2f"; "1 18"."第203串" format="%#.2f"; "1 18"."第一串 20" format="%#.2f"; "1 18"."第202串" format="%#.2f"; "1 18"."第一串 18" format="%#.2f"; "1 18"."第201串" format="%#.2f"; "1 18"."第一串 16" format="%#.2f"; "1 18"."第200串" format="%#.2f"; "1 18"."第一串 14" format="%#.2f"; "1 18"."第199串" format="%#.2f"; "1 18"."第一串 12" format="%#.2f"; "1 18"."第198串" format="%#.2f"; "1 18"."第一串 10" format="%#.2f"; "1 18"."第197串" format="%#.2f"; "1 18"."第一串 8" format="%#.2f"; "1 18"."第196串" format="%#.2f"; "1 18"."第一串 6" format="%#.2f"; "1 18"."第195串" format="%#.2f"; "1 18"."第一串 4" format="%#.2f"; "1 18"."第194串" format="%#.2f"; "1 18"."第一串 2" format="%#.2f"; "1 18"."第193串" format="%#.2f"}
  out "1 7":T7 {"第一串 24" format="%#.2f"; "第300串" format="%#.2f"; "第一串 22" format="%#.2f"; "第299串" format="%#.2f"; "第一串 20" format="%#.2f"; "第298串" format="%#.2f"; "第一串 18" format="%#.2f"; "第297串" format="%#.2f"; "第一串 16" format="%#.2f"; "第296串" format="%#.2f"; "第一串 14" format="%#.2f"; "第295串" format="%#.2f"; "第一串 12" format="%#.2f"; "第294串" format="%#.2f"; "第一串 10" format="%#.2f"; "第293串" format="%#.2f"; "第一串 8" format="%#.2f"; "第292串" format="%#.2f"; "第一串 6" format="%#.2f"; "第291串" format="%#.2f"; "第一串 4" format="%#.2f"; "第290串" format="%#.2f"; "第一串 2" format="%#.2f"; "第289串" format="%#.2f"}
  in  "故障信息选择按键 5":enum32{"单选选项2", "单选选项2 2", "单选选项2 3", "单选选项1"}(radio)=enum."单选选项1"
  out "电压选择 4":enum32{"1-96", "97-192", "193-288", "289-300"}(tab)
  out "1 108":T13 {"1 102"."第一串 24" format="%#.2f"; "1 102"."第12串" format="%#.2f"; "1 102"."第一串 22" format="%#.2f"; "1 102"."第11串" format="%#.2f"; "1 102"."第一串 20" format="%#.2f"; "1 102"."第10串" format="%#.2f"; "1 102"."第一串 18" format="%#.2f"; "1 102"."第9串" format="%#.2f"; "1 102"."第一串 16" format="%#.2f"; "1 102"."第8串" format="%#.2f"; "1 102"."第一串 14" format="%#.2f"; "1 102"."第7串" format="%#.2f"; "1 102"."第一串 12" format="%#.2f"; "1 102"."第6串" format="%#.2f"; "1 102"."第一串 10" format="%#.2f"; "1 102"."第5串" format="%#.2f"; "1 102"."第一串 8" format="%#.2f"; "1 102"."第4串" format="%#.2f"; "1 102"."第一串 6" format="%#.2f"; "1 102"."第3串" format="%#.2f"; "1 102"."第一串 4" format="%#.2f"; "1 102"."第2串" format="%#.2f"; "1 102"."第一串 2" format="%#.2f"; "1 102"."第1串" format="%#.2f"}
  out "1 109":T11 {"1 26"."第一串 24" format="%#.2f"; "1 26"."第108串" format="%#.2f"; "1 26"."第一串 22" format="%#.2f"; "1 26"."第107串" format="%#.2f"; "1 26"."第一串 20" format="%#.2f"; "1 26"."第106串" format="%#.2f"; "1 26"."第一串 18" format="%#.2f"; "1 26"."第105串" format="%#.2f"; "1 26"."第一串 16" format="%#.2f"; "1 26"."第104串" format="%#.2f"; "1 26"."第一串 14" format="%#.2f"; "1 26"."第103串" format="%#.2f"; "1 26"."第一串 12" format="%#.2f"; "1 26"."第102串" format="%#.2f"; "1 26"."第一串 10" format="%#.2f"; "1 26"."第101串" format="%#.2f"; "1 26"."第一串 8" format="%#.2f"; "1 26"."第100串" format="%#.2f"; "1 26"."第一串 6" format="%#.2f"; "1 26"."第99串" format="%#.2f"; "1 26"."第一串 4" format="%#.2f"; "1 26"."第98串" format="%#.2f"; "1 26"."第一串 2" format="%#.2f"; "1 26"."第97串" format="%#.2f"}
  out "1 29":T12 {"1 18"."第一串 24" format="%#.2f"; "1 18"."第204串" format="%#.2f"; "1 18"."第一串 22" format="%#.2f"; "1 18"."第203串" format="%#.2f"; "1 18"."第一串 20" format="%#.2f"; "1 18"."第202串" format="%#.2f"; "1 18"."第一串 18" format="%#.2f"; "1 18"."第201串" format="%#.2f"; "1 18"."第一串 16" format="%#.2f"; "1 18"."第200串" format="%#.2f"; "1 18"."第一串 14" format="%#.2f"; "1 18"."第199串" format="%#.2f"; "1 18"."第一串 12" format="%#.2f"; "1 18"."第198串" format="%#.2f"; "1 18"."第一串 10" format="%#.2f"; "1 18"."第197串" format="%#.2f"; "1 18"."第一串 8" format="%#.2f"; "1 18"."第196串" format="%#.2f"; "1 18"."第一串 6" format="%#.2f"; "1 18"."第195串" format="%#.2f"; "1 18"."第一串 4" format="%#.2f"; "1 18"."第194串" format="%#.2f"; "1 18"."第一串 2" format="%#.2f"; "1 18"."第193串" format="%#.2f"}
  out "1 8":T7 {"第一串 24" format="%#.2f"; "第300串" format="%#.2f"; "第一串 22" format="%#.2f"; "第299串" format="%#.2f"; "第一串 20" format="%#.2f"; "第298串" format="%#.2f"; "第一串 18" format="%#.2f"; "第297串" format="%#.2f"; "第一串 16" format="%#.2f"; "第296串" format="%#.2f"; "第一串 14" format="%#.2f"; "第295串" format="%#.2f"; "第一串 12" format="%#.2f"; "第294串" format="%#.2f"; "第一串 10" format="%#.2f"; "第293串" format="%#.2f"; "第一串 8" format="%#.2f"; "第292串" format="%#.2f"; "第一串 6" format="%#.2f"; "第291串" format="%#.2f"; "第一串 4" format="%#.2f"; "第290串" format="%#.2f"; "第一串 2" format="%#.2f"; "第289串" format="%#.2f"}
  out "单选选项2":bool
  # "主板详细信息"
  # "主板详细信息"
  # "监控上位机"
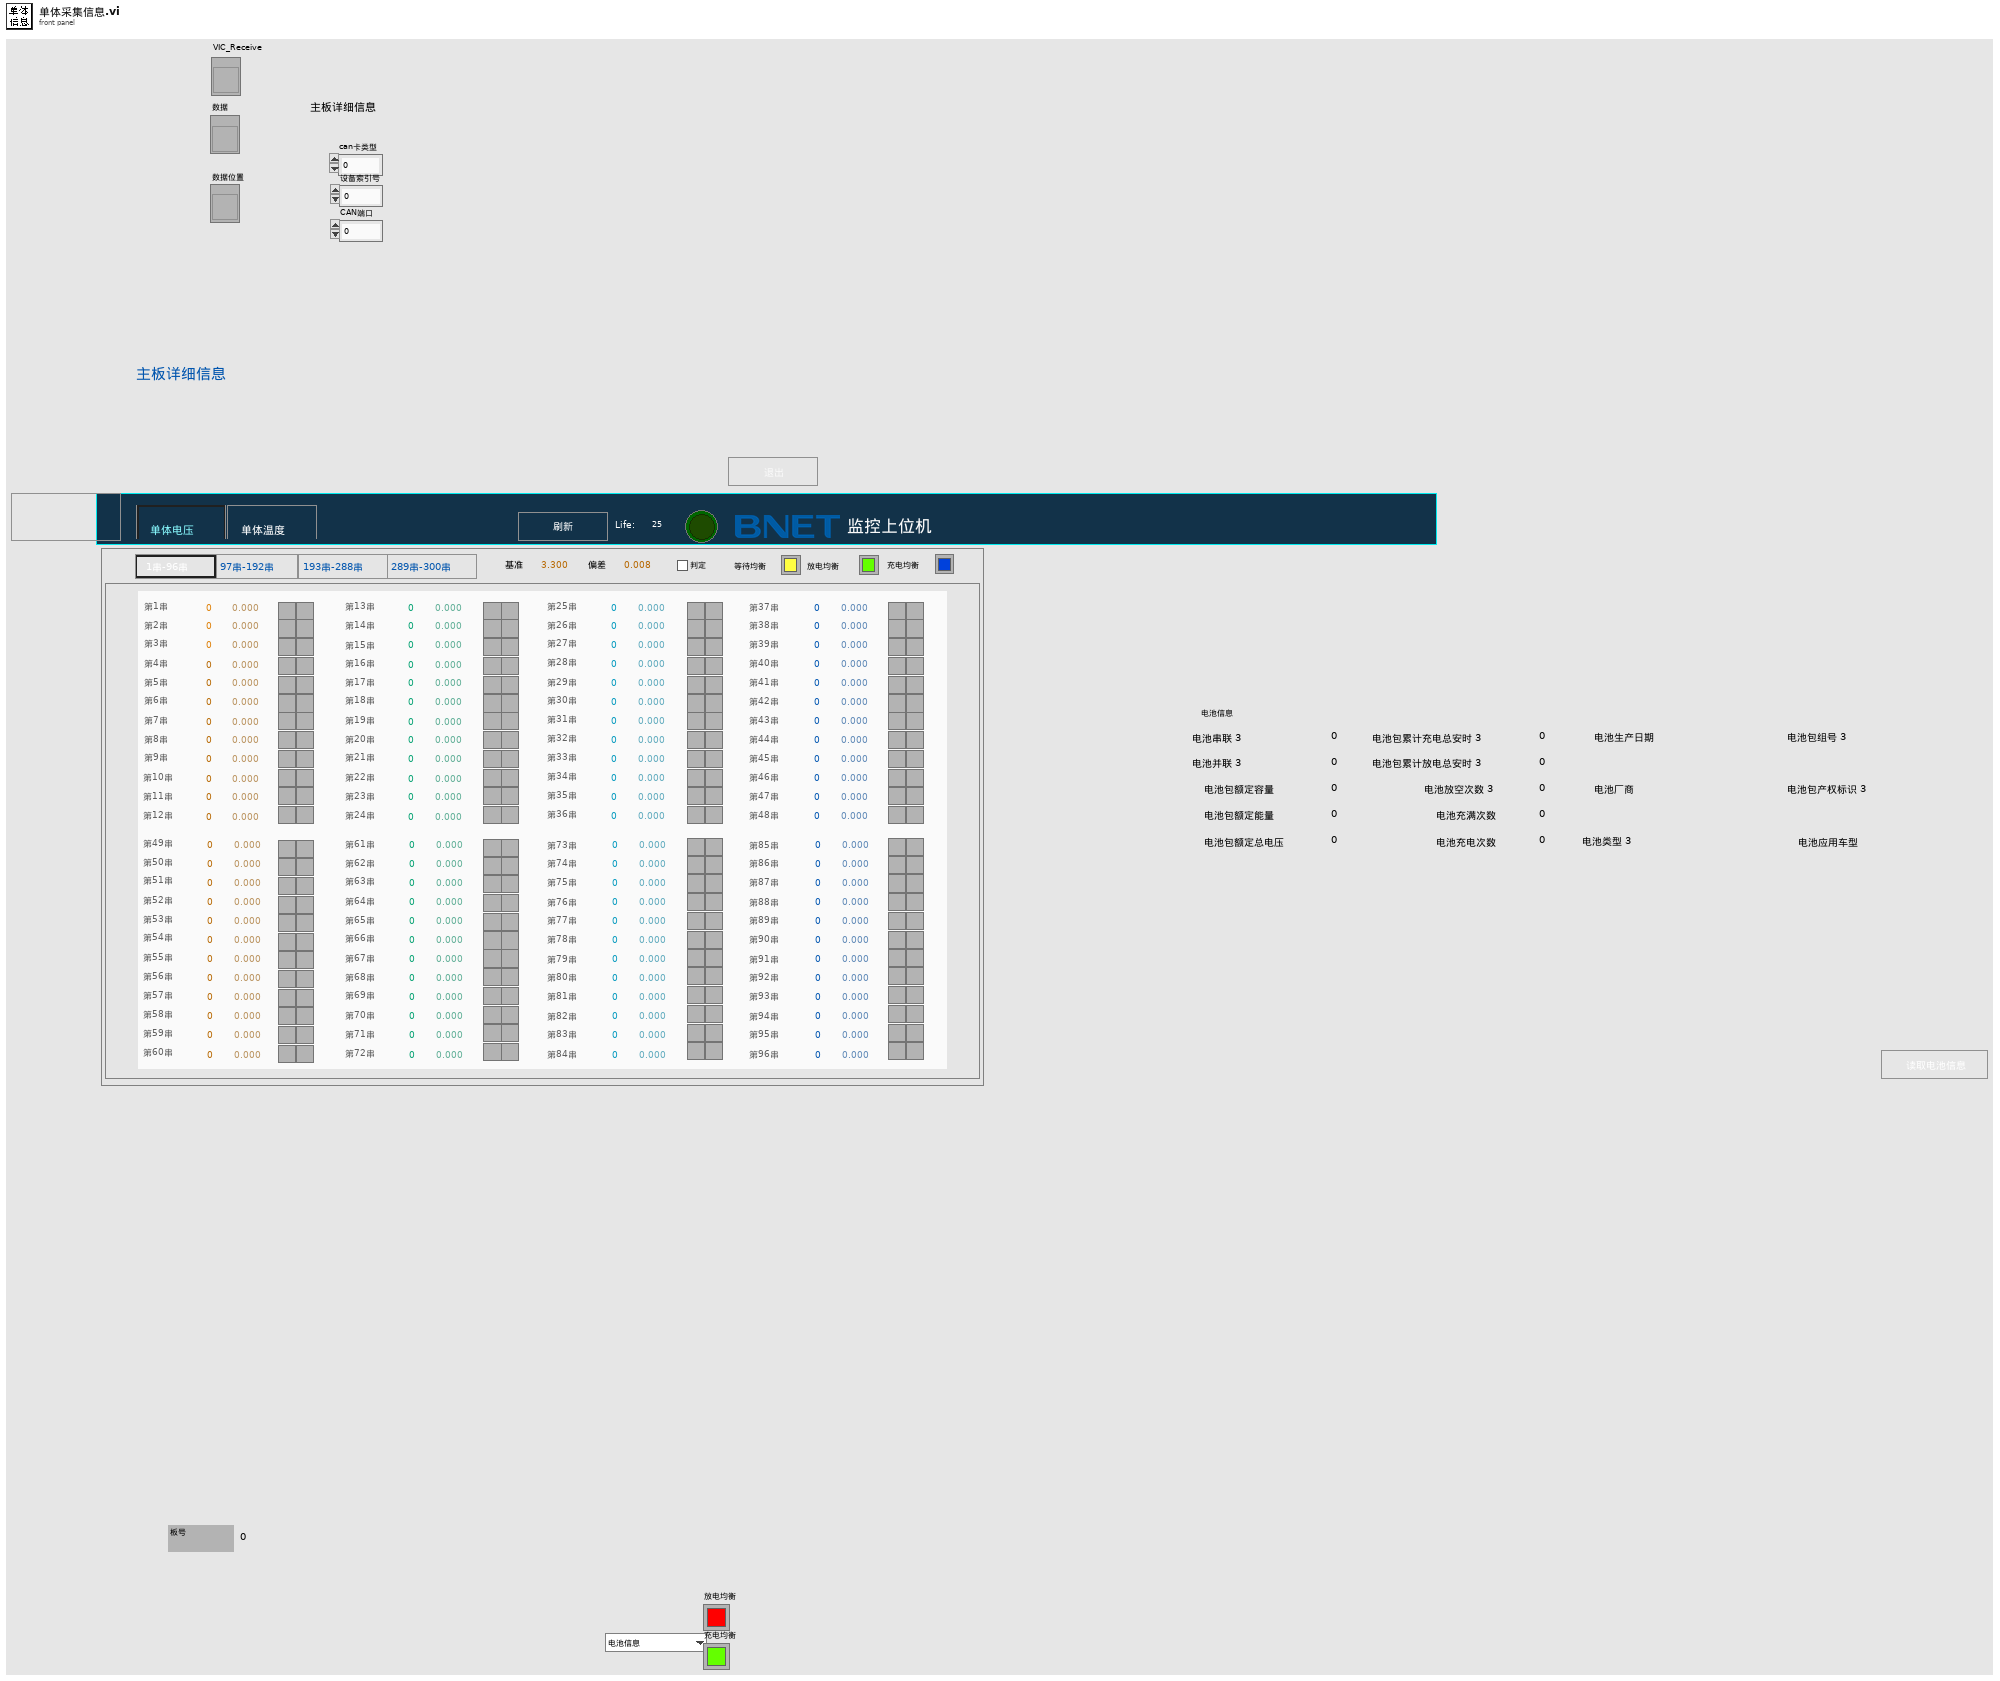
[diagram p1: front panel]
types:
  T1 = cluster{"ID":u32, "TimeStamp":u32, "TimeFlag":u8, "SendType":u8, "RemoteFlag":u8, "ExternFlag":u8, "DataLen":u8, "Data1":u8, "Data2":u8, "Data3":u8, "Data4":u8, "Data5":u8, "Data6":u8, "Data7":u8, "Data8":u8, "Rsv1":u8, "Rsv2":u8, "Rsv3":u8}
  T2 = cluster{"电池串联 3":dbl, "电池并联 3":dbl, "电池包累计放电总安时 3":dbl, "电池包额定容量":dbl, "电池包额定能量":dbl, "电池包额定总电压":dbl, "电池包累计充电总安时 3":dbl, "电池充满次数":dbl, "电池放空次数 3":dbl, "电池充电次数":dbl, "电池生产日期":string, "电池厂商":string, "电池类型 3":string, "电池包组号 3":string, "电池包产权标识 3":string, "电池应用车型":string}
  T3 = enum32{"单选选项2 5", "单选选项2 6", "单选选项2 7", "单选选项2 8"}
  T4 = cluster{"1 102":cluster{"第1串":dbl, "第2串":dbl, "第3串":dbl, "第4串":dbl, "第5串":dbl, "第6串":dbl, "第7串":dbl, "第8串":dbl, "第9串":dbl, "第10串":dbl, "第11串":dbl, "第12串":dbl, "第一串 2":dbl, "第一串 4":dbl, "第一串 6":dbl, "第一串 8":dbl, "第一串 10":dbl, "第一串 12":dbl, "第一串 14":dbl, "第一串 16":dbl, "第一串 18":dbl, "第一串 20":dbl, "第一串 22":dbl, "第一串 24":dbl}, "1 3":cluster{"第13串":dbl, "第14串":dbl, "第15串":dbl, "第16串":dbl, "第17串":dbl, "第18串":dbl, "第19串":dbl, "第20串":dbl, "第21串":dbl, "第22串":dbl, "第23串":dbl, "第24串":dbl, "第一串 2":dbl, "第一串 4":dbl, "第一串 6":dbl, "第一串 8":dbl, "第一串 10":dbl, "第一串 12":dbl, "第一串 14":dbl, "第一串 16":dbl, "第一串 18":dbl, "第一串 20":dbl, "第一串 22":dbl, "第一串 24":dbl}, "1 4":cluster{"第25串":dbl, "第26串":dbl, "第27串":dbl, "第28串":dbl, "第29串":dbl, "第30串":dbl, "第31串":dbl, "第32串":dbl, "第33串":dbl, "第34串":dbl, "第35串":dbl, "第36串":dbl, "第一串 2":dbl, "第一串 4":dbl, "第一串 6":dbl, "第一串 8":dbl, "第一串 10":dbl, "第一串 12":dbl, "第一串 14":dbl, "第一串 16":dbl, "第一串 18":dbl, "第一串 20":dbl, "第一串 22":dbl, "第一串 24":dbl}, "1 6":cluster{"第37串":dbl, "第38串":dbl, "第39串":dbl, "第40串":dbl, "第41串":dbl, "第42串":dbl, "第43串":dbl, "第44串":dbl, "第45串":dbl, "第46串":dbl, "第47串":dbl, "第48串":dbl, "第一串 2":dbl, "第一串 4":dbl, "第一串 6":dbl, "第一串 8":dbl, "第一串 10":dbl, "第一串 12":dbl, "第一串 14":dbl, "第一串 16":dbl, "第一串 18":dbl, "第一串 20":dbl, "第一串 22":dbl, "第一串 24":dbl}, "1 7":cluster{"第49串":dbl, "第50串":dbl, "第51串":dbl, "第52串":dbl, "第53串":dbl, "第54串":dbl, "第55串":dbl, "第56串":dbl, "第57串":dbl, "第58串":dbl, "第59串":dbl, "第60串":dbl, "第一串 2":dbl, "第一串 4":dbl, "第一串 6":dbl, "第一串 8":dbl, "第一串 10":dbl, "第一串 12":dbl, "第一串 14":dbl, "第一串 16":dbl, "第一串 18":dbl, "第一串 20":dbl, "第一串 22":dbl, "第一串 24":dbl}, "1 8":cluster{"第61串":dbl, "第62串":dbl, "第63串":dbl, "第64串":dbl, "第65串":dbl, "第66串":dbl, "第67串":dbl, "第68串":dbl, "第69串":dbl, "第70串":dbl, "第71串":dbl, "第72串":dbl, "第一串 2":dbl, "第一串 4":dbl, "第一串 6":dbl, "第一串 8":dbl, "第一串 10":dbl, "第一串 12":dbl, "第一串 14":dbl, "第一串 16":dbl, "第一串 18":dbl, "第一串 20":dbl, "第一串 22":dbl, "第一串 24":dbl}, "1 9":cluster{"第73串":dbl, "第74串":dbl, "第75串":dbl, "第76串":dbl, "第77串":dbl, "第78串":dbl, "第79串":dbl, "第80串":dbl, "第81串":dbl, "第82串":dbl, "第83串":dbl, "第84串":dbl, "第一串 2":dbl, "第一串 4":dbl, "第一串 6":dbl, "第一串 8":dbl, "第一串 10":dbl, "第一串 12":dbl, "第一串 14":dbl, "第一串 16":dbl, "第一串 18":dbl, "第一串 20":dbl, "第一串 22":dbl, "第一串 24":dbl}, "1 10":cluster{"第85串":dbl, "第86串":dbl, "第87串":dbl, "第88串":dbl, "第89串":dbl, "第90串":dbl, "第91串":dbl, "第92串":dbl, "第93串":dbl, "第94串":dbl, "第95串":dbl, "第96串":dbl, "第一串 2":dbl, "第一串 4":dbl, "第一串 6":dbl, "第一串 8":dbl, "第一串 10":dbl, "第一串 12":dbl, "第一串 14":dbl, "第一串 16":dbl, "第一串 18":dbl, "第一串 20":dbl, "第一串 22":dbl, "第一串 24":dbl}, "1 12":cluster{"充电1":u32, "充电1":u32, "充电1":u32, "充电1":u32, "充电1":u32, "充电1":u32, "充电1":u32, "充电1":u32, "充电1":u32, "充电1":u32, "充电1":u32, "充电1":u32}, "1 28":cluster{"充电1":u32, "充电1":u32, "充电1":u32, "充电1":u32, "充电1":u32, "充电1":u32, "充电1":u32, "充电1":u32, "充电1":u32, "充电1":u32, "充电1":u32, "充电1":u32}, "1 25":cluster{"充电1":u32, "充电1":u32, "充电1":u32, "充电1":u32, "充电1":u32, "充电1":u32, "充电1":u32, "充电1":u32, "充电1":u32, "充电1":u32, "充电1":u32, "充电1":u32}, "1 31":cluster{"充电1":u32, "充电1":u32, "充电1":u32, "充电1":u32, "充电1":u32, "充电1":u32, "充电1":u32, "充电1":u32, "充电1":u32, "充电1":u32, "充电1":u32, "充电1":u32}, "1 16":cluster{"充电1":u32, "充电1":u32, "充电1":u32, "充电1":u32, "充电1":u32, "充电1":u32, "充电1":u32, "充电1":u32, "充电1":u32, "充电1":u32, "充电1":u32, "充电1":u32}, "1 19":cluster{"充电1":u32, "充电1":u32, "充电1":u32, "充电1":u32, "充电1":u32, "充电1":u32, "充电1":u32, "充电1":u32, "充电1":u32, "充电1":u32, "充电1":u32, "充电1":u32}, "1 22":cluster{"充电1":u32, "充电1":u32, "充电1":u32, "充电1":u32, "充电1":u32, "充电1":u32, "充电1":u32, "充电1":u32, "充电1":u32, "充电1":u32, "充电1":u32, "充电1":u32}, "1 34":cluster{"充电1":u32, "充电1":u32, "充电1":u32, "充电1":u32, "充电1":u32, "充电1":u32, "充电1":u32, "充电1":u32, "充电1":u32, "充电1":u32, "充电1":u32, "充电1":u32}, "1 11":cluster{"充电1":u32, "充电1":u32, "充电1":u32, "充电1":u32, "充电1":u32, "充电1":u32, "充电1":u32, "充电1":u32, "充电1":u32, "充电1":u32, "充电1":u32, "充电1":u32}, "1 27":cluster{"充电1":u32, "充电1":u32, "充电1":u32, "充电1":u32, "充电1":u32, "充电1":u32, "充电1":u32, "充电1":u32, "充电1":u32, "充电1":u32, "充电1":u32, "充电1":u32}, "1 24":cluster{"充电1":u32, "充电1":u32, "充电1":u32, "充电1":u32, "充电1":u32, "充电1":u32, "充电1":u32, "充电1":u32, "充电1":u32, "充电1":u32, "充电1":u32, "充电1":u32}, "1 30":cluster{"充电1":u32, "充电1":u32, "充电1":u32, "充电1":u32, "充电1":u32, "充电1":u32, "充电1":u32, "充电1":u32, "充电1":u32, "充电1":u32, "充电1":u32, "充电1":u32}, "1 15":cluster{"充电1":u32, "充电1":u32, "充电1":u32, "充电1":u32, "充电1":u32, "充电1":u32, "充电1":u32, "充电1":u32, "充电1":u32, "充电1":u32, "充电1":u32, "充电1":u32}, "1 18":cluster{"充电1":u32, "充电1":u32, "充电1":u32, "充电1":u32, "充电1":u32, "充电1":u32, "充电1":u32, "充电1":u32, "充电1":u32, "充电1":u32, "充电1":u32, "充电1":u32}, "1 21":cluster{"充电1":u32, "充电1":u32, "充电1":u32, "充电1":u32, "充电1":u32, "充电1":u32, "充电1":u32, "充电1":u32, "充电1":u32, "充电1":u32, "充电1":u32, "充电1":u32}, "1 33":cluster{"充电1":u32, "充电1":u32, "充电1":u32, "充电1":u32, "充电1":u32, "充电1":u32, "充电1":u32, "充电1":u32, "充电1":u32, "充电1":u32, "充电1":u32, "充电1":u32}, "1 13":cluster{"均衡故障":i32, "均衡故障 2":dbl, "均衡故障 3":dbl, "均衡故障 4":dbl, "均衡故障 5":dbl, "均衡故障 6":dbl, "均衡故障 7":dbl, "均衡故障 8":dbl, "均衡故障 9":dbl, "均衡故障 10":dbl, "均衡故障 11":dbl, "均衡故障 12":dbl}, "1 26":cluster{"均衡故障":i32, "均衡故障 2":dbl, "均衡故障 3":dbl, "均衡故障 4":dbl, "均衡故障 5":dbl, "均衡故障 6":dbl, "均衡故障 7":dbl, "均衡故障 8":dbl, "均衡故障 9":dbl, "均衡故障 10":dbl, "均衡故障 11":dbl, "均衡故障 12":dbl}, "1 23":cluster{"均衡故障":i32, "均衡故障 2":dbl, "均衡故障 3":dbl, "均衡故障 4":dbl, "均衡故障 5":dbl, "均衡故障 6":dbl, "均衡故障 7":dbl, "均衡故障 8":dbl, "均衡故障 9":dbl, "均衡故障 10":dbl, "均衡故障 11":dbl, "均衡故障 12":dbl}, "1 29":cluster{"均衡故障":i32, "均衡故障 2":dbl, "均衡故障 3":dbl, "均衡故障 4":dbl, "均衡故障 5":dbl, "均衡故障 6":dbl, "均衡故障 7":dbl, "均衡故障 8":dbl, "均衡故障 9":dbl, "均衡故障 10":dbl, "均衡故障 11":dbl, "均衡故障 12":dbl}, "1 14":cluster{"均衡故障":i32, "均衡故障 2":dbl, "均衡故障 3":dbl, "均衡故障 4":dbl, "均衡故障 5":dbl, "均衡故障 6":dbl, "均衡故障 7":dbl, "均衡故障 8":dbl, "均衡故障 9":dbl, "均衡故障 10":dbl, "均衡故障 11":dbl, "均衡故障 12":dbl}, "1 17":cluster{"均衡故障":i32, "均衡故障 2":dbl, "均衡故障 3":dbl, "均衡故障 4":dbl, "均衡故障 5":dbl, "均衡故障 6":dbl, "均衡故障 7":dbl, "均衡故障 8":dbl, "均衡故障 9":dbl, "均衡故障 10":dbl, "均衡故障 11":dbl, "均衡故障 12":dbl}, "1 20":cluster{"均衡故障":i32, "均衡故障 2":dbl, "均衡故障 3":dbl, "均衡故障 4":dbl, "均衡故障 5":dbl, "均衡故障 6":dbl, "均衡故障 7":dbl, "均衡故障 8":dbl, "均衡故障 9":dbl, "均衡故障 10":dbl, "均衡故障 11":dbl, "均衡故障 12":dbl}, "1 32":cluster{"均衡故障":i32, "均衡故障 2":dbl, "均衡故障 3":dbl, "均衡故障 4":dbl, "均衡故障 5":dbl, "均衡故障 6":dbl, "均衡故障 7":dbl, "均衡故障 8":dbl, "均衡故障 9":dbl, "均衡故障 10":dbl, "均衡故障 11":dbl, "均衡故障 12":dbl}}
  T5 = cluster{"1 26":cluster{"第97串":dbl, "第98串":dbl, "第99串":dbl, "第100串":dbl, "第101串":dbl, "第102串":dbl, "第103串":dbl, "第104串":dbl, "第105串":dbl, "第106串":dbl, "第107串":dbl, "第108串":dbl, "第一串 2":dbl, "第一串 4":dbl, "第一串 6":dbl, "第一串 8":dbl, "第一串 10":dbl, "第一串 12":dbl, "第一串 14":dbl, "第一串 16":dbl, "第一串 18":dbl, "第一串 20":dbl, "第一串 22":dbl, "第一串 24":dbl}, "1 27":cluster{"第109串":dbl, "第110串":dbl, "第111串":dbl, "第112串":dbl, "第113串":dbl, "第114串":dbl, "第115串":dbl, "第116串":dbl, "第117串":dbl, "第118串":dbl, "第119串":dbl, "第120串":dbl, "第一串 2":dbl, "第一串 4":dbl, "第一串 6":dbl, "第一串 8":dbl, "第一串 10":dbl, "第一串 12":dbl, "第一串 14":dbl, "第一串 16":dbl, "第一串 18":dbl, "第一串 20":dbl, "第一串 22":dbl, "第一串 24":dbl}, "1 28":cluster{"第121串":dbl, "第122串":dbl, "第123串":dbl, "第124串":dbl, "第125串":dbl, "第126串":dbl, "第127串":dbl, "第128串":dbl, "第129串":dbl, "第130串":dbl, "第131串":dbl, "第132串":dbl, "第一串 2":dbl, "第一串 4":dbl, "第一串 6":dbl, "第一串 8":dbl, "第一串 10":dbl, "第一串 12":dbl, "第一串 14":dbl, "第一串 16":dbl, "第一串 18":dbl, "第一串 20":dbl, "第一串 22":dbl, "第一串 24":dbl}, "1 29":cluster{"第133串":dbl, "第134串":dbl, "第135串":dbl, "第136串":dbl, "第137串":dbl, "第138串":dbl, "第139串":dbl, "第140串":dbl, "第141串":dbl, "第142串":dbl, "第143串":dbl, "第144串":dbl, "第一串 2":dbl, "第一串 4":dbl, "第一串 6":dbl, "第一串 8":dbl, "第一串 10":dbl, "第一串 12":dbl, "第一串 14":dbl, "第一串 16":dbl, "第一串 18":dbl, "第一串 20":dbl, "第一串 22":dbl, "第一串 24":dbl}, "1 30":cluster{"第145串":dbl, "第146串":dbl, "第147串":dbl, "第148串":dbl, "第149串":dbl, "第150串":dbl, "第151串":dbl, "第152串":dbl, "第153串":dbl, "第154串":dbl, "第155串":dbl, "第156串":dbl, "第一串 2":dbl, "第一串 4":dbl, "第一串 6":dbl, "第一串 8":dbl, "第一串 10":dbl, "第一串 12":dbl, "第一串 14":dbl, "第一串 16":dbl, "第一串 18":dbl, "第一串 20":dbl, "第一串 22":dbl, "第一串 24":dbl}, "1 31":cluster{"第157串":dbl, "第158串":dbl, "第159串":dbl, "第160串":dbl, "第161串":dbl, "第162串":dbl, "第163串":dbl, "第164串":dbl, "第165串":dbl, "第166串":dbl, "第167串":dbl, "第168串":dbl, "第一串 2":dbl, "第一串 4":dbl, "第一串 6":dbl, "第一串 8":dbl, "第一串 10":dbl, "第一串 12":dbl, "第一串 14":dbl, "第一串 16":dbl, "第一串 18":dbl, "第一串 20":dbl, "第一串 22":dbl, "第一串 24":dbl}, "1 32":cluster{"第169串":dbl, "第170串":dbl, "第171串":dbl, "第172串":dbl, "第173串":dbl, "第174串":dbl, "第175串":dbl, "第176串":dbl, "第177串":dbl, "第178串":dbl, "第179串":dbl, "第180串":dbl, "第一串 2":dbl, "第一串 4":dbl, "第一串 6":dbl, "第一串 8":dbl, "第一串 10":dbl, "第一串 12":dbl, "第一串 14":dbl, "第一串 16":dbl, "第一串 18":dbl, "第一串 20":dbl, "第一串 22":dbl, "第一串 24":dbl}, "1 33":cluster{"第181串":dbl, "第182串":dbl, "第183串":dbl, "第184串":dbl, "第185串":dbl, "第186串":dbl, "第187串":dbl, "第188串":dbl, "第189串":dbl, "第190串":dbl, "第191串":dbl, "第192串":dbl, "第一串 2":dbl, "第一串 4":dbl, "第一串 6":dbl, "第一串 8":dbl, "第一串 10":dbl, "第一串 12":dbl, "第一串 14":dbl, "第一串 16":dbl, "第一串 18":dbl, "第一串 20":dbl, "第一串 22":dbl, "第一串 24":dbl}, "1 16":cluster{"充电1":u32, "充电1":u32, "充电1":u32, "充电1":u32, "充电1":u32, "充电1":u32, "充电1":u32, "充电1":u32, "充电1":u32, "充电1":u32, "充电1":u32, "充电1":u32}, "1 44":cluster{"充电1":u32, "充电1":u32, "充电1":u32, "充电1":u32, "充电1":u32, "充电1":u32, "充电1":u32, "充电1":u32, "充电1":u32, "充电1":u32, "充电1":u32, "充电1":u32}, "1 36":cluster{"充电1":u32, "充电1":u32, "充电1":u32, "充电1":u32, "充电1":u32, "充电1":u32, "充电1":u32, "充电1":u32, "充电1":u32, "充电1":u32, "充电1":u32, "充电1":u32}, "1 47":cluster{"充电1":u32, "充电1":u32, "充电1":u32, "充电1":u32, "充电1":u32, "充电1":u32, "充电1":u32, "充电1":u32, "充电1":u32, "充电1":u32, "充电1":u32, "充电1":u32}, "1 19":cluster{"充电1":u32, "充电1":u32, "充电1":u32, "充电1":u32, "充电1":u32, "充电1":u32, "充电1":u32, "充电1":u32, "充电1":u32, "充电1":u32, "充电1":u32, "充电1":u32}, "1 38":cluster{"充电1":u32, "充电1":u32, "充电1":u32, "充电1":u32, "充电1":u32, "充电1":u32, "充电1":u32, "充电1":u32, "充电1":u32, "充电1":u32, "充电1":u32, "充电1":u32}, "1 41":cluster{"充电1":u32, "充电1":u32, "充电1":u32, "充电1":u32, "充电1":u32, "充电1":u32, "充电1":u32, "充电1":u32, "充电1":u32, "充电1":u32, "充电1":u32, "充电1":u32}, "1 50":cluster{"充电1":u32, "充电1":u32, "充电1":u32, "充电1":u32, "充电1":u32, "充电1":u32, "充电1":u32, "充电1":u32, "充电1":u32, "充电1":u32, "充电1":u32, "充电1":u32}, "1 15":cluster{"充电1":u32, "充电1":u32, "充电1":u32, "充电1":u32, "充电1":u32, "充电1":u32, "充电1":u32, "充电1":u32, "充电1":u32, "充电1":u32, "充电1":u32, "充电1":u32}, "1 43":cluster{"充电1":u32, "充电1":u32, "充电1":u32, "充电1":u32, "充电1":u32, "充电1":u32, "充电1":u32, "充电1":u32, "充电1":u32, "充电1":u32, "充电1":u32, "充电1":u32}, "1 35":cluster{"充电1":u32, "充电1":u32, "充电1":u32, "充电1":u32, "充电1":u32, "充电1":u32, "充电1":u32, "充电1":u32, "充电1":u32, "充电1":u32, "充电1":u32, "充电1":u32}, "1 46":cluster{"充电1":u32, "充电1":u32, "充电1":u32, "充电1":u32, "充电1":u32, "充电1":u32, "充电1":u32, "充电1":u32, "充电1":u32, "充电1":u32, "充电1":u32, "充电1":u32}, "1 18":cluster{"充电1":u32, "充电1":u32, "充电1":u32, "充电1":u32, "充电1":u32, "充电1":u32, "充电1":u32, "充电1":u32, "充电1":u32, "充电1":u32, "充电1":u32, "充电1":u32}, "1 37":cluster{"充电1":u32, "充电1":u32, "充电1":u32, "充电1":u32, "充电1":u32, "充电1":u32, "充电1":u32, "充电1":u32, "充电1":u32, "充电1":u32, "充电1":u32, "充电1":u32}, "1 40":cluster{"充电1":u32, "充电1":u32, "充电1":u32, "充电1":u32, "充电1":u32, "充电1":u32, "充电1":u32, "充电1":u32, "充电1":u32, "充电1":u32, "充电1":u32, "充电1":u32}, "1 49":cluster{"充电1":u32, "充电1":u32, "充电1":u32, "充电1":u32, "充电1":u32, "充电1":u32, "充电1":u32, "充电1":u32, "充电1":u32, "充电1":u32, "充电1":u32, "充电1":u32}, "1 14":cluster{"均衡故障":i32, "均衡故障 2":dbl, "均衡故障 3":dbl, "均衡故障 4":dbl, "均衡故障 5":dbl, "均衡故障 6":dbl, "均衡故障 7":dbl, "均衡故障 8":dbl, "均衡故障 9":dbl, "均衡故障 10":dbl, "均衡故障 11":dbl, "均衡故障 12":dbl}, "1 42":cluster{"均衡故障":i32, "均衡故障 2":dbl, "均衡故障 3":dbl, "均衡故障 4":dbl, "均衡故障 5":dbl, "均衡故障 6":dbl, "均衡故障 7":dbl, "均衡故障 8":dbl, "均衡故障 9":dbl, "均衡故障 10":dbl, "均衡故障 11":dbl, "均衡故障 12":dbl}, "1 34":cluster{"均衡故障":i32, "均衡故障 2":dbl, "均衡故障 3":dbl, "均衡故障 4":dbl, "均衡故障 5":dbl, "均衡故障 6":dbl, "均衡故障 7":dbl, "均衡故障 8":dbl, "均衡故障 9":dbl, "均衡故障 10":dbl, "均衡故障 11":dbl, "均衡故障 12":dbl}, "1 45":cluster{"均衡故障":i32, "均衡故障 2":dbl, "均衡故障 3":dbl, "均衡故障 4":dbl, "均衡故障 5":dbl, "均衡故障 6":dbl, "均衡故障 7":dbl, "均衡故障 8":dbl, "均衡故障 9":dbl, "均衡故障 10":dbl, "均衡故障 11":dbl, "均衡故障 12":dbl}, "1 17":cluster{"均衡故障":i32, "均衡故障 2":dbl, "均衡故障 3":dbl, "均衡故障 4":dbl, "均衡故障 5":dbl, "均衡故障 6":dbl, "均衡故障 7":dbl, "均衡故障 8":dbl, "均衡故障 9":dbl, "均衡故障 10":dbl, "均衡故障 11":dbl, "均衡故障 12":dbl}, "1 20":cluster{"均衡故障":i32, "均衡故障 2":dbl, "均衡故障 3":dbl, "均衡故障 4":dbl, "均衡故障 5":dbl, "均衡故障 6":dbl, "均衡故障 7":dbl, "均衡故障 8":dbl, "均衡故障 9":dbl, "均衡故障 10":dbl, "均衡故障 11":dbl, "均衡故障 12":dbl}, "1 39":cluster{"均衡故障":i32, "均衡故障 2":dbl, "均衡故障 3":dbl, "均衡故障 4":dbl, "均衡故障 5":dbl, "均衡故障 6":dbl, "均衡故障 7":dbl, "均衡故障 8":dbl, "均衡故障 9":dbl, "均衡故障 10":dbl, "均衡故障 11":dbl, "均衡故障 12":dbl}, "1 48":cluster{"均衡故障":i32, "均衡故障 2":dbl, "均衡故障 3":dbl, "均衡故障 4":dbl, "均衡故障 5":dbl, "均衡故障 6":dbl, "均衡故障 7":dbl, "均衡故障 8":dbl, "均衡故障 9":dbl, "均衡故障 10":dbl, "均衡故障 11":dbl, "均衡故障 12":dbl}}
  T6 = cluster{"1 18":cluster{"第193串":dbl, "第194串":dbl, "第195串":dbl, "第196串":dbl, "第197串":dbl, "第198串":dbl, "第199串":dbl, "第200串":dbl, "第201串":dbl, "第202串":dbl, "第203串":dbl, "第204串":dbl, "第一串 2":dbl, "第一串 4":dbl, "第一串 6":dbl, "第一串 8":dbl, "第一串 10":dbl, "第一串 12":dbl, "第一串 14":dbl, "第一串 16":dbl, "第一串 18":dbl, "第一串 20":dbl, "第一串 22":dbl, "第一串 24":dbl}, "1 19":cluster{"第205串":dbl, "第206串":dbl, "第207串":dbl, "第208串":dbl, "第209串":dbl, "第210串":dbl, "第211串":dbl, "第212串":dbl, "第213串":dbl, "第214串":dbl, "第215串":dbl, "第216串":dbl, "第一串 2":dbl, "第一串 4":dbl, "第一串 6":dbl, "第一串 8":dbl, "第一串 10":dbl, "第一串 12":dbl, "第一串 14":dbl, "第一串 16":dbl, "第一串 18":dbl, "第一串 20":dbl, "第一串 22":dbl, "第一串 24":dbl}, "1 20":cluster{"第217串":dbl, "第218串":dbl, "第219串":dbl, "第220串":dbl, "第221串":dbl, "第222串":dbl, "第223串":dbl, "第224串":dbl, "第225串":dbl, "第226串":dbl, "第227串":dbl, "第228串":dbl, "第一串 2":dbl, "第一串 4":dbl, "第一串 6":dbl, "第一串 8":dbl, "第一串 10":dbl, "第一串 12":dbl, "第一串 14":dbl, "第一串 16":dbl, "第一串 18":dbl, "第一串 20":dbl, "第一串 22":dbl, "第一串 24":dbl}, "1 21":cluster{"第229串":dbl, "第230串":dbl, "第231串":dbl, "第232串":dbl, "第233串":dbl, "第234串":dbl, "第235串":dbl, "第236串":dbl, "第237串":dbl, "第238串":dbl, "第239串":dbl, "第240串":dbl, "第一串 2":dbl, "第一串 4":dbl, "第一串 6":dbl, "第一串 8":dbl, "第一串 10":dbl, "第一串 12":dbl, "第一串 14":dbl, "第一串 16":dbl, "第一串 18":dbl, "第一串 20":dbl, "第一串 22":dbl, "第一串 24":dbl}, "1 22":cluster{"第241串":dbl, "第242串":dbl, "第243串":dbl, "第244串":dbl, "第245串":dbl, "第246串":dbl, "第247串":dbl, "第248串":dbl, "第249串":dbl, "第250串":dbl, "第251串":dbl, "第252串":dbl, "第一串 2":dbl, "第一串 4":dbl, "第一串 6":dbl, "第一串 8":dbl, "第一串 10":dbl, "第一串 12":dbl, "第一串 14":dbl, "第一串 16":dbl, "第一串 18":dbl, "第一串 20":dbl, "第一串 22":dbl, "第一串 24":dbl}, "1 23":cluster{"第253串":dbl, "第254串":dbl, "第255串":dbl, "第256串":dbl, "第257串":dbl, "第258串":dbl, "第259串":dbl, "第260串":dbl, "第261串":dbl, "第262串":dbl, "第263串":dbl, "第264串":dbl, "第一串 2":dbl, "第一串 4":dbl, "第一串 6":dbl, "第一串 8":dbl, "第一串 10":dbl, "第一串 12":dbl, "第一串 14":dbl, "第一串 16":dbl, "第一串 18":dbl, "第一串 20":dbl, "第一串 22":dbl, "第一串 24":dbl}, "1 24":cluster{"第265串":dbl, "第266串":dbl, "第267串":dbl, "第268串":dbl, "第269串":dbl, "第270串":dbl, "第271串":dbl, "第272串":dbl, "第273串":dbl, "第274串":dbl, "第275串":dbl, "第276串":dbl, "第一串 2":dbl, "第一串 4":dbl, "第一串 6":dbl, "第一串 8":dbl, "第一串 10":dbl, "第一串 12":dbl, "第一串 14":dbl, "第一串 16":dbl, "第一串 18":dbl, "第一串 20":dbl, "第一串 22":dbl, "第一串 24":dbl}, "1 25":cluster{"第277串":dbl, "第278串":dbl, "第279串":dbl, "第280串":dbl, "第281串":dbl, "第282串":dbl, "第283串":dbl, "第284串":dbl, "第285串":dbl, "第286串":dbl, "第287串":dbl, "第288串":dbl, "第一串 2":dbl, "第一串 4":dbl, "第一串 6":dbl, "第一串 8":dbl, "第一串 10":dbl, "第一串 12":dbl, "第一串 14":dbl, "第一串 16":dbl, "第一串 18":dbl, "第一串 20":dbl, "第一串 22":dbl, "第一串 24":dbl}, "1 12":cluster{"充电1":u32, "充电1":u32, "充电1":u32, "充电1":u32, "充电1":u32, "充电1":u32, "充电1":u32, "充电1":u32, "充电1":u32, "充电1":u32, "充电1":u32, "充电1":u32}, "1 39":cluster{"充电1":u32, "充电1":u32, "充电1":u32, "充电1":u32, "充电1":u32, "充电1":u32, "充电1":u32, "充电1":u32, "充电1":u32, "充电1":u32, "充电1":u32, "充电1":u32}, "1 28":cluster{"充电1":u32, "充电1":u32, "充电1":u32, "充电1":u32, "充电1":u32, "充电1":u32, "充电1":u32, "充电1":u32, "充电1":u32, "充电1":u32, "充电1":u32, "充电1":u32}, "1 42":cluster{"充电1":u32, "充电1":u32, "充电1":u32, "充电1":u32, "充电1":u32, "充电1":u32, "充电1":u32, "充电1":u32, "充电1":u32, "充电1":u32, "充电1":u32, "充电1":u32}, "1 16":cluster{"充电1":u32, "充电1":u32, "充电1":u32, "充电1":u32, "充电1":u32, "充电1":u32, "充电1":u32, "充电1":u32, "充电1":u32, "充电1":u32, "充电1":u32, "充电1":u32}, "1 30":cluster{"充电1":u32, "充电1":u32, "充电1":u32, "充电1":u32, "充电1":u32, "充电1":u32, "充电1":u32, "充电1":u32, "充电1":u32, "充电1":u32, "充电1":u32, "充电1":u32}, "1 33":cluster{"充电1":u32, "充电1":u32, "充电1":u32, "充电1":u32, "充电1":u32, "充电1":u32, "充电1":u32, "充电1":u32, "充电1":u32, "充电1":u32, "充电1":u32, "充电1":u32}, "1 36":cluster{"充电1":u32, "充电1":u32, "充电1":u32, "充电1":u32, "充电1":u32, "充电1":u32, "充电1":u32, "充电1":u32, "充电1":u32, "充电1":u32, "充电1":u32, "充电1":u32}, "1 11":cluster{"充电1":u32, "充电1":u32, "充电1":u32, "充电1":u32, "充电1":u32, "充电1":u32, "充电1":u32, "充电1":u32, "充电1":u32, "充电1":u32, "充电1":u32, "充电1":u32}, "1 38":cluster{"充电1":u32, "充电1":u32, "充电1":u32, "充电1":u32, "充电1":u32, "充电1":u32, "充电1":u32, "充电1":u32, "充电1":u32, "充电1":u32, "充电1":u32, "充电1":u32}, "1 27":cluster{"充电1":u32, "充电1":u32, "充电1":u32, "充电1":u32, "充电1":u32, "充电1":u32, "充电1":u32, "充电1":u32, "充电1":u32, "充电1":u32, "充电1":u32, "充电1":u32}, "1 41":cluster{"充电1":u32, "充电1":u32, "充电1":u32, "充电1":u32, "充电1":u32, "充电1":u32, "充电1":u32, "充电1":u32, "充电1":u32, "充电1":u32, "充电1":u32, "充电1":u32}, "1 15":cluster{"充电1":u32, "充电1":u32, "充电1":u32, "充电1":u32, "充电1":u32, "充电1":u32, "充电1":u32, "充电1":u32, "充电1":u32, "充电1":u32, "充电1":u32, "充电1":u32}, "1 29":cluster{"充电1":u32, "充电1":u32, "充电1":u32, "充电1":u32, "充电1":u32, "充电1":u32, "充电1":u32, "充电1":u32, "充电1":u32, "充电1":u32, "充电1":u32, "充电1":u32}, "1 32":cluster{"充电1":u32, "充电1":u32, "充电1":u32, "充电1":u32, "充电1":u32, "充电1":u32, "充电1":u32, "充电1":u32, "充电1":u32, "充电1":u32, "充电1":u32, "充电1":u32}, "1 35":cluster{"充电1":u32, "充电1":u32, "充电1":u32, "充电1":u32, "充电1":u32, "充电1":u32, "充电1":u32, "充电1":u32, "充电1":u32, "充电1":u32, "充电1":u32, "充电1":u32}, "1 13":cluster{"均衡故障":i32, "均衡故障 2":dbl, "均衡故障 3":dbl, "均衡故障 4":dbl, "均衡故障 5":dbl, "均衡故障 6":dbl, "均衡故障 7":dbl, "均衡故障 8":dbl, "均衡故障 9":dbl, "均衡故障 10":dbl, "均衡故障 11":dbl, "均衡故障 12":dbl}, "1 37":cluster{"均衡故障":i32, "均衡故障 2":dbl, "均衡故障 3":dbl, "均衡故障 4":dbl, "均衡故障 5":dbl, "均衡故障 6":dbl, "均衡故障 7":dbl, "均衡故障 8":dbl, "均衡故障 9":dbl, "均衡故障 10":dbl, "均衡故障 11":dbl, "均衡故障 12":dbl}, "1 26":cluster{"均衡故障":i32, "均衡故障 2":dbl, "均衡故障 3":dbl, "均衡故障 4":dbl, "均衡故障 5":dbl, "均衡故障 6":dbl, "均衡故障 7":dbl, "均衡故障 8":dbl, "均衡故障 9":dbl, "均衡故障 10":dbl, "均衡故障 11":dbl, "均衡故障 12":dbl}, "1 40":cluster{"均衡故障":i32, "均衡故障 2":dbl, "均衡故障 3":dbl, "均衡故障 4":dbl, "均衡故障 5":dbl, "均衡故障 6":dbl, "均衡故障 7":dbl, "均衡故障 8":dbl, "均衡故障 9":dbl, "均衡故障 10":dbl, "均衡故障 11":dbl, "均衡故障 12":dbl}, "1 14":cluster{"均衡故障":i32, "均衡故障 2":dbl, "均衡故障 3":dbl, "均衡故障 4":dbl, "均衡故障 5":dbl, "均衡故障 6":dbl, "均衡故障 7":dbl, "均衡故障 8":dbl, "均衡故障 9":dbl, "均衡故障 10":dbl, "均衡故障 11":dbl, "均衡故障 12":dbl}, "1 17":cluster{"均衡故障":i32, "均衡故障 2":dbl, "均衡故障 3":dbl, "均衡故障 4":dbl, "均衡故障 5":dbl, "均衡故障 6":dbl, "均衡故障 7":dbl, "均衡故障 8":dbl, "均衡故障 9":dbl, "均衡故障 10":dbl, "均衡故障 11":dbl, "均衡故障 12":dbl}, "1 31":cluster{"均衡故障":i32, "均衡故障 2":dbl, "均衡故障 3":dbl, "均衡故障 4":dbl, "均衡故障 5":dbl, "均衡故障 6":dbl, "均衡故障 7":dbl, "均衡故障 8":dbl, "均衡故障 9":dbl, "均衡故障 10":dbl, "均衡故障 11":dbl, "均衡故障 12":dbl}, "1 34":cluster{"均衡故障":i32, "均衡故障 2":dbl, "均衡故障 3":dbl, "均衡故障 4":dbl, "均衡故障 5":dbl, "均衡故障 6":dbl, "均衡故障 7":dbl, "均衡故障 8":dbl, "均衡故障 9":dbl, "均衡故障 10":dbl, "均衡故障 11":dbl, "均衡故障 12":dbl}}
  T7 = cluster{"第289串":dbl, "第290串":dbl, "第291串":dbl, "第292串":dbl, "第293串":dbl, "第294串":dbl, "第295串":dbl, "第296串":dbl, "第297串":dbl, "第298串":dbl, "第299串":dbl, "第300串":dbl, "第一串 2":dbl, "第一串 4":dbl, "第一串 6":dbl, "第一串 8":dbl, "第一串 10":dbl, "第一串 12":dbl, "第一串 14":dbl, "第一串 16":dbl, "第一串 18":dbl, "第一串 20":dbl, "第一串 22":dbl, "第一串 24":dbl}
  T8 = cluster{"均衡故障":i32, "均衡故障 2":dbl, "均衡故障 3":dbl, "均衡故障 4":dbl, "均衡故障 5":dbl, "均衡故障 6":dbl, "均衡故障 7":dbl, "均衡故障 8":dbl, "均衡故障 9":dbl, "均衡故障 10":dbl, "均衡故障 11":dbl, "均衡故障 12":dbl}
  T9 = cluster{"充电1":u32, "充电1":u32, "充电1":u32, "充电1":u32, "充电1":u32, "充电1":u32, "充电1":u32, "充电1":u32, "充电1":u32, "充电1":u32, "充电1":u32, "充电1":u32}
  T10 = cluster{"1 102":cluster{"第1串":dbl, "第2串":dbl, "第3串":dbl, "第4串":dbl, "第5串":dbl, "第6串":dbl, "第7串":dbl, "第8串":dbl, "第9串":dbl, "第10串":dbl, "第11串":dbl, "第12串":dbl, "第一串 2":dbl, "第一串 4":dbl, "第一串 6":dbl, "第一串 8":dbl, "第一串 10":dbl, "第一串 12":dbl, "第一串 14":dbl, "第一串 16":dbl, "第一串 18":dbl, "第一串 20":dbl, "第一串 22":dbl, "第一串 24":dbl}, "1 3":cluster{"第13串":dbl, "第14串":dbl, "第15串":dbl, "第16串":dbl, "第17串":dbl, "第18串":dbl, "第19串":dbl, "第20串":dbl, "第21串":dbl, "第22串":dbl, "第23串":dbl, "第24串":dbl, "第一串 2":dbl, "第一串 4":dbl, "第一串 6":dbl, "第一串 8":dbl, "第一串 10":dbl, "第一串 12":dbl, "第一串 14":dbl, "第一串 16":dbl, "第一串 18":dbl, "第一串 20":dbl, "第一串 22":dbl, "第一串 24":dbl}, "1 4":cluster{"第25串":dbl, "第26串":dbl, "第27串":dbl, "第28串":dbl, "第29串":dbl, "第30串":dbl, "第31串":dbl, "第32串":dbl, "第33串":dbl, "第34串":dbl, "第35串":dbl, "第36串":dbl, "第一串 2":dbl, "第一串 4":dbl, "第一串 6":dbl, "第一串 8":dbl, "第一串 10":dbl, "第一串 12":dbl, "第一串 14":dbl, "第一串 16":dbl, "第一串 18":dbl, "第一串 20":dbl, "第一串 22":dbl, "第一串 24":dbl}, "1 6":cluster{"第37串":dbl, "第38串":dbl, "第39串":dbl, "第40串":dbl, "第41串":dbl, "第42串":dbl, "第43串":dbl, "第44串":dbl, "第45串":dbl, "第46串":dbl, "第47串":dbl, "第48串":dbl, "第一串 2":dbl, "第一串 4":dbl, "第一串 6":dbl, "第一串 8":dbl, "第一串 10":dbl, "第一串 12":dbl, "第一串 14":dbl, "第一串 16":dbl, "第一串 18":dbl, "第一串 20":dbl, "第一串 22":dbl, "第一串 24":dbl}, "1 7":cluster{"第49串":dbl, "第50串":dbl, "第51串":dbl, "第52串":dbl, "第53串":dbl, "第54串":dbl, "第55串":dbl, "第56串":dbl, "第57串":dbl, "第58串":dbl, "第59串":dbl, "第60串":dbl, "第一串 2":dbl, "第一串 4":dbl, "第一串 6":dbl, "第一串 8":dbl, "第一串 10":dbl, "第一串 12":dbl, "第一串 14":dbl, "第一串 16":dbl, "第一串 18":dbl, "第一串 20":dbl, "第一串 22":dbl, "第一串 24":dbl}, "1 8":cluster{"第61串":dbl, "第62串":dbl, "第63串":dbl, "第64串":dbl, "第65串":dbl, "第66串":dbl, "第67串":dbl, "第68串":dbl, "第69串":dbl, "第70串":dbl, "第71串":dbl, "第72串":dbl, "第一串 2":dbl, "第一串 4":dbl, "第一串 6":dbl, "第一串 8":dbl, "第一串 10":dbl, "第一串 12":dbl, "第一串 14":dbl, "第一串 16":dbl, "第一串 18":dbl, "第一串 20":dbl, "第一串 22":dbl, "第一串 24":dbl}, "1 9":cluster{"第73串":dbl, "第74串":dbl, "第75串":dbl, "第76串":dbl, "第77串":dbl, "第78串":dbl, "第79串":dbl, "第80串":dbl, "第81串":dbl, "第82串":dbl, "第83串":dbl, "第84串":dbl, "第一串 2":dbl, "第一串 4":dbl, "第一串 6":dbl, "第一串 8":dbl, "第一串 10":dbl, "第一串 12":dbl, "第一串 14":dbl, "第一串 16":dbl, "第一串 18":dbl, "第一串 20":dbl, "第一串 22":dbl, "第一串 24":dbl}, "1 10":cluster{"第85串":dbl, "第86串":dbl, "第87串":dbl, "第88串":dbl, "第89串":dbl, "第90串":dbl, "第91串":dbl, "第92串":dbl, "第93串":dbl, "第94串":dbl, "第95串":dbl, "第96串":dbl, "第一串 2":dbl, "第一串 4":dbl, "第一串 6":dbl, "第一串 8":dbl, "第一串 10":dbl, "第一串 12":dbl, "第一串 14":dbl, "第一串 16":dbl, "第一串 18":dbl, "第一串 20":dbl, "第一串 22":dbl, "第一串 24":dbl}}
  T11 = cluster{"1 26":cluster{"第97串":dbl, "第98串":dbl, "第99串":dbl, "第100串":dbl, "第101串":dbl, "第102串":dbl, "第103串":dbl, "第104串":dbl, "第105串":dbl, "第106串":dbl, "第107串":dbl, "第108串":dbl, "第一串 2":dbl, "第一串 4":dbl, "第一串 6":dbl, "第一串 8":dbl, "第一串 10":dbl, "第一串 12":dbl, "第一串 14":dbl, "第一串 16":dbl, "第一串 18":dbl, "第一串 20":dbl, "第一串 22":dbl, "第一串 24":dbl}, "1 27":cluster{"第109串":dbl, "第110串":dbl, "第111串":dbl, "第112串":dbl, "第113串":dbl, "第114串":dbl, "第115串":dbl, "第116串":dbl, "第117串":dbl, "第118串":dbl, "第119串":dbl, "第120串":dbl, "第一串 2":dbl, "第一串 4":dbl, "第一串 6":dbl, "第一串 8":dbl, "第一串 10":dbl, "第一串 12":dbl, "第一串 14":dbl, "第一串 16":dbl, "第一串 18":dbl, "第一串 20":dbl, "第一串 22":dbl, "第一串 24":dbl}, "1 28":cluster{"第121串":dbl, "第122串":dbl, "第123串":dbl, "第124串":dbl, "第125串":dbl, "第126串":dbl, "第127串":dbl, "第128串":dbl, "第129串":dbl, "第130串":dbl, "第131串":dbl, "第132串":dbl, "第一串 2":dbl, "第一串 4":dbl, "第一串 6":dbl, "第一串 8":dbl, "第一串 10":dbl, "第一串 12":dbl, "第一串 14":dbl, "第一串 16":dbl, "第一串 18":dbl, "第一串 20":dbl, "第一串 22":dbl, "第一串 24":dbl}, "1 29":cluster{"第133串":dbl, "第134串":dbl, "第135串":dbl, "第136串":dbl, "第137串":dbl, "第138串":dbl, "第139串":dbl, "第140串":dbl, "第141串":dbl, "第142串":dbl, "第143串":dbl, "第144串":dbl, "第一串 2":dbl, "第一串 4":dbl, "第一串 6":dbl, "第一串 8":dbl, "第一串 10":dbl, "第一串 12":dbl, "第一串 14":dbl, "第一串 16":dbl, "第一串 18":dbl, "第一串 20":dbl, "第一串 22":dbl, "第一串 24":dbl}, "1 30":cluster{"第145串":dbl, "第146串":dbl, "第147串":dbl, "第148串":dbl, "第149串":dbl, "第150串":dbl, "第151串":dbl, "第152串":dbl, "第153串":dbl, "第154串":dbl, "第155串":dbl, "第156串":dbl, "第一串 2":dbl, "第一串 4":dbl, "第一串 6":dbl, "第一串 8":dbl, "第一串 10":dbl, "第一串 12":dbl, "第一串 14":dbl, "第一串 16":dbl, "第一串 18":dbl, "第一串 20":dbl, "第一串 22":dbl, "第一串 24":dbl}, "1 31":cluster{"第157串":dbl, "第158串":dbl, "第159串":dbl, "第160串":dbl, "第161串":dbl, "第162串":dbl, "第163串":dbl, "第164串":dbl, "第165串":dbl, "第166串":dbl, "第167串":dbl, "第168串":dbl, "第一串 2":dbl, "第一串 4":dbl, "第一串 6":dbl, "第一串 8":dbl, "第一串 10":dbl, "第一串 12":dbl, "第一串 14":dbl, "第一串 16":dbl, "第一串 18":dbl, "第一串 20":dbl, "第一串 22":dbl, "第一串 24":dbl}, "1 32":cluster{"第169串":dbl, "第170串":dbl, "第171串":dbl, "第172串":dbl, "第173串":dbl, "第174串":dbl, "第175串":dbl, "第176串":dbl, "第177串":dbl, "第178串":dbl, "第179串":dbl, "第180串":dbl, "第一串 2":dbl, "第一串 4":dbl, "第一串 6":dbl, "第一串 8":dbl, "第一串 10":dbl, "第一串 12":dbl, "第一串 14":dbl, "第一串 16":dbl, "第一串 18":dbl, "第一串 20":dbl, "第一串 22":dbl, "第一串 24":dbl}, "1 33":cluster{"第181串":dbl, "第182串":dbl, "第183串":dbl, "第184串":dbl, "第185串":dbl, "第186串":dbl, "第187串":dbl, "第188串":dbl, "第189串":dbl, "第190串":dbl, "第191串":dbl, "第192串":dbl, "第一串 2":dbl, "第一串 4":dbl, "第一串 6":dbl, "第一串 8":dbl, "第一串 10":dbl, "第一串 12":dbl, "第一串 14":dbl, "第一串 16":dbl, "第一串 18":dbl, "第一串 20":dbl, "第一串 22":dbl, "第一串 24":dbl}}
  T12 = cluster{"1 18":cluster{"第193串":dbl, "第194串":dbl, "第195串":dbl, "第196串":dbl, "第197串":dbl, "第198串":dbl, "第199串":dbl, "第200串":dbl, "第201串":dbl, "第202串":dbl, "第203串":dbl, "第204串":dbl, "第一串 2":dbl, "第一串 4":dbl, "第一串 6":dbl, "第一串 8":dbl, "第一串 10":dbl, "第一串 12":dbl, "第一串 14":dbl, "第一串 16":dbl, "第一串 18":dbl, "第一串 20":dbl, "第一串 22":dbl, "第一串 24":dbl}, "1 19":cluster{"第205串":dbl, "第206串":dbl, "第207串":dbl, "第208串":dbl, "第209串":dbl, "第210串":dbl, "第211串":dbl, "第212串":dbl, "第213串":dbl, "第214串":dbl, "第215串":dbl, "第216串":dbl, "第一串 2":dbl, "第一串 4":dbl, "第一串 6":dbl, "第一串 8":dbl, "第一串 10":dbl, "第一串 12":dbl, "第一串 14":dbl, "第一串 16":dbl, "第一串 18":dbl, "第一串 20":dbl, "第一串 22":dbl, "第一串 24":dbl}, "1 20":cluster{"第217串":dbl, "第218串":dbl, "第219串":dbl, "第220串":dbl, "第221串":dbl, "第222串":dbl, "第223串":dbl, "第224串":dbl, "第225串":dbl, "第226串":dbl, "第227串":dbl, "第228串":dbl, "第一串 2":dbl, "第一串 4":dbl, "第一串 6":dbl, "第一串 8":dbl, "第一串 10":dbl, "第一串 12":dbl, "第一串 14":dbl, "第一串 16":dbl, "第一串 18":dbl, "第一串 20":dbl, "第一串 22":dbl, "第一串 24":dbl}, "1 21":cluster{"第229串":dbl, "第230串":dbl, "第231串":dbl, "第232串":dbl, "第233串":dbl, "第234串":dbl, "第235串":dbl, "第236串":dbl, "第237串":dbl, "第238串":dbl, "第239串":dbl, "第240串":dbl, "第一串 2":dbl, "第一串 4":dbl, "第一串 6":dbl, "第一串 8":dbl, "第一串 10":dbl, "第一串 12":dbl, "第一串 14":dbl, "第一串 16":dbl, "第一串 18":dbl, "第一串 20":dbl, "第一串 22":dbl, "第一串 24":dbl}, "1 22":cluster{"第241串":dbl, "第242串":dbl, "第243串":dbl, "第244串":dbl, "第245串":dbl, "第246串":dbl, "第247串":dbl, "第248串":dbl, "第249串":dbl, "第250串":dbl, "第251串":dbl, "第252串":dbl, "第一串 2":dbl, "第一串 4":dbl, "第一串 6":dbl, "第一串 8":dbl, "第一串 10":dbl, "第一串 12":dbl, "第一串 14":dbl, "第一串 16":dbl, "第一串 18":dbl, "第一串 20":dbl, "第一串 22":dbl, "第一串 24":dbl}, "1 23":cluster{"第253串":dbl, "第254串":dbl, "第255串":dbl, "第256串":dbl, "第257串":dbl, "第258串":dbl, "第259串":dbl, "第260串":dbl, "第261串":dbl, "第262串":dbl, "第263串":dbl, "第264串":dbl, "第一串 2":dbl, "第一串 4":dbl, "第一串 6":dbl, "第一串 8":dbl, "第一串 10":dbl, "第一串 12":dbl, "第一串 14":dbl, "第一串 16":dbl, "第一串 18":dbl, "第一串 20":dbl, "第一串 22":dbl, "第一串 24":dbl}, "1 24":cluster{"第265串":dbl, "第266串":dbl, "第267串":dbl, "第268串":dbl, "第269串":dbl, "第270串":dbl, "第271串":dbl, "第272串":dbl, "第273串":dbl, "第274串":dbl, "第275串":dbl, "第276串":dbl, "第一串 2":dbl, "第一串 4":dbl, "第一串 6":dbl, "第一串 8":dbl, "第一串 10":dbl, "第一串 12":dbl, "第一串 14":dbl, "第一串 16":dbl, "第一串 18":dbl, "第一串 20":dbl, "第一串 22":dbl, "第一串 24":dbl}, "1 25":cluster{"第277串":dbl, "第278串":dbl, "第279串":dbl, "第280串":dbl, "第281串":dbl, "第282串":dbl, "第283串":dbl, "第284串":dbl, "第285串":dbl, "第286串":dbl, "第287串":dbl, "第288串":dbl, "第一串 2":dbl, "第一串 4":dbl, "第一串 6":dbl, "第一串 8":dbl, "第一串 10":dbl, "第一串 12":dbl, "第一串 14":dbl, "第一串 16":dbl, "第一串 18":dbl, "第一串 20":dbl, "第一串 22":dbl, "第一串 24":dbl}}
  T13 = cluster{"1 3":cluster{"第13串":dbl, "第14串":dbl, "第15串":dbl, "第16串":dbl, "第17串":dbl, "第18串":dbl, "第19串":dbl, "第20串":dbl, "第21串":dbl, "第22串":dbl, "第23串":dbl, "第24串":dbl, "第一串 2":dbl, "第一串 4":dbl, "第一串 6":dbl, "第一串 8":dbl, "第一串 10":dbl, "第一串 12":dbl, "第一串 14":dbl, "第一串 16":dbl, "第一串 18":dbl, "第一串 20":dbl, "第一串 22":dbl, "第一串 24":dbl}, "1 4":cluster{"第25串":dbl, "第26串":dbl, "第27串":dbl, "第28串":dbl, "第29串":dbl, "第30串":dbl, "第31串":dbl, "第32串":dbl, "第33串":dbl, "第34串":dbl, "第35串":dbl, "第36串":dbl, "第一串 2":dbl, "第一串 4":dbl, "第一串 6":dbl, "第一串 8":dbl, "第一串 10":dbl, "第一串 12":dbl, "第一串 14":dbl, "第一串 16":dbl, "第一串 18":dbl, "第一串 20":dbl, "第一串 22":dbl, "第一串 24":dbl}, "1 6":cluster{"第37串":dbl, "第38串":dbl, "第39串":dbl, "第40串":dbl, "第41串":dbl, "第42串":dbl, "第43串":dbl, "第44串":dbl, "第45串":dbl, "第46串":dbl, "第47串":dbl, "第48串":dbl, "第一串 2":dbl, "第一串 4":dbl, "第一串 6":dbl, "第一串 8":dbl, "第一串 10":dbl, "第一串 12":dbl, "第一串 14":dbl, "第一串 16":dbl, "第一串 18":dbl, "第一串 20":dbl, "第一串 22":dbl, "第一串 24":dbl}, "1 7":cluster{"第49串":dbl, "第50串":dbl, "第51串":dbl, "第52串":dbl, "第53串":dbl, "第54串":dbl, "第55串":dbl, "第56串":dbl, "第57串":dbl, "第58串":dbl, "第59串":dbl, "第60串":dbl, "第一串 2":dbl, "第一串 4":dbl, "第一串 6":dbl, "第一串 8":dbl, "第一串 10":dbl, "第一串 12":dbl, "第一串 14":dbl, "第一串 16":dbl, "第一串 18":dbl, "第一串 20":dbl, "第一串 22":dbl, "第一串 24":dbl}, "1 8":cluster{"第61串":dbl, "第62串":dbl, "第63串":dbl, "第64串":dbl, "第65串":dbl, "第66串":dbl, "第67串":dbl, "第68串":dbl, "第69串":dbl, "第70串":dbl, "第71串":dbl, "第72串":dbl, "第一串 2":dbl, "第一串 4":dbl, "第一串 6":dbl, "第一串 8":dbl, "第一串 10":dbl, "第一串 12":dbl, "第一串 14":dbl, "第一串 16":dbl, "第一串 18":dbl, "第一串 20":dbl, "第一串 22":dbl, "第一串 24":dbl}, "1 9":cluster{"第73串":dbl, "第74串":dbl, "第75串":dbl, "第76串":dbl, "第77串":dbl, "第78串":dbl, "第79串":dbl, "第80串":dbl, "第81串":dbl, "第82串":dbl, "第83串":dbl, "第84串":dbl, "第一串 2":dbl, "第一串 4":dbl, "第一串 6":dbl, "第一串 8":dbl, "第一串 10":dbl, "第一串 12":dbl, "第一串 14":dbl, "第一串 16":dbl, "第一串 18":dbl, "第一串 20":dbl, "第一串 22":dbl, "第一串 24":dbl}, "1 10":cluster{"第85串":dbl, "第86串":dbl, "第87串":dbl, "第88串":dbl, "第89串":dbl, "第90串":dbl, "第91串":dbl, "第92串":dbl, "第93串":dbl, "第94串":dbl, "第95串":dbl, "第96串":dbl, "第一串 2":dbl, "第一串 4":dbl, "第一串 6":dbl, "第一串 8":dbl, "第一串 10":dbl, "第一串 12":dbl, "第一串 14":dbl, "第一串 16":dbl, "第一串 18":dbl, "第一串 20":dbl, "第一串 22":dbl, "第一串 24":dbl}, "1 102":cluster{"第1串":dbl, "第2串":dbl, "第3串":dbl, "第4串":dbl, "第5串":dbl, "第6串":dbl, "第7串":dbl, "第8串":dbl, "第9串":dbl, "第10串":dbl, "第11串":dbl, "第12串":dbl, "第一串 2":dbl, "第一串 4":dbl, "第一串 6":dbl, "第一串 8":dbl, "第一串 10":dbl, "第一串 12":dbl, "第一串 14":dbl, "第一串 16":dbl, "第一串 18":dbl, "第一串 20":dbl, "第一串 22":dbl, "第一串 24":dbl}}
  T14 = enum32{"Invalid", "Standard", "Closed", "Hidden", "Minimized", "Maximized"}
  T15 = cluster{"[0]":u32, "[1]":u32, "[2]":u32, "[3]":u32, "[4]":u32, "[5]":u32, "[6]":u32, "[7]":u32, "[8]":u32, "[9]":u32, "[10]":u32, "[11]":u32}
  T16 = cluster{"[0]":dbl, "[1]":dbl, "[2]":dbl, "[3]":dbl, "[4]":dbl, "[5]":dbl, "[6]":dbl, "[7]":dbl, "[8]":dbl, "[9]":dbl, "[10]":dbl, "[11]":dbl}
  T17 = cluster{"[0]":dbl, "[1]":dbl, "[2]":dbl, "[3]":dbl, "[4]":dbl, "[5]":dbl, "[6]":dbl, "[7]":dbl, "[8]":dbl, "[9]":dbl, "[10]":dbl, "[11]":dbl, "[12]":dbl, "[13]":dbl, "[14]":dbl, "[15]":dbl, "[16]":dbl, "[17]":dbl, "[18]":dbl, "[19]":dbl, "[20]":dbl, "[21]":dbl, "[22]":dbl, "[23]":dbl}
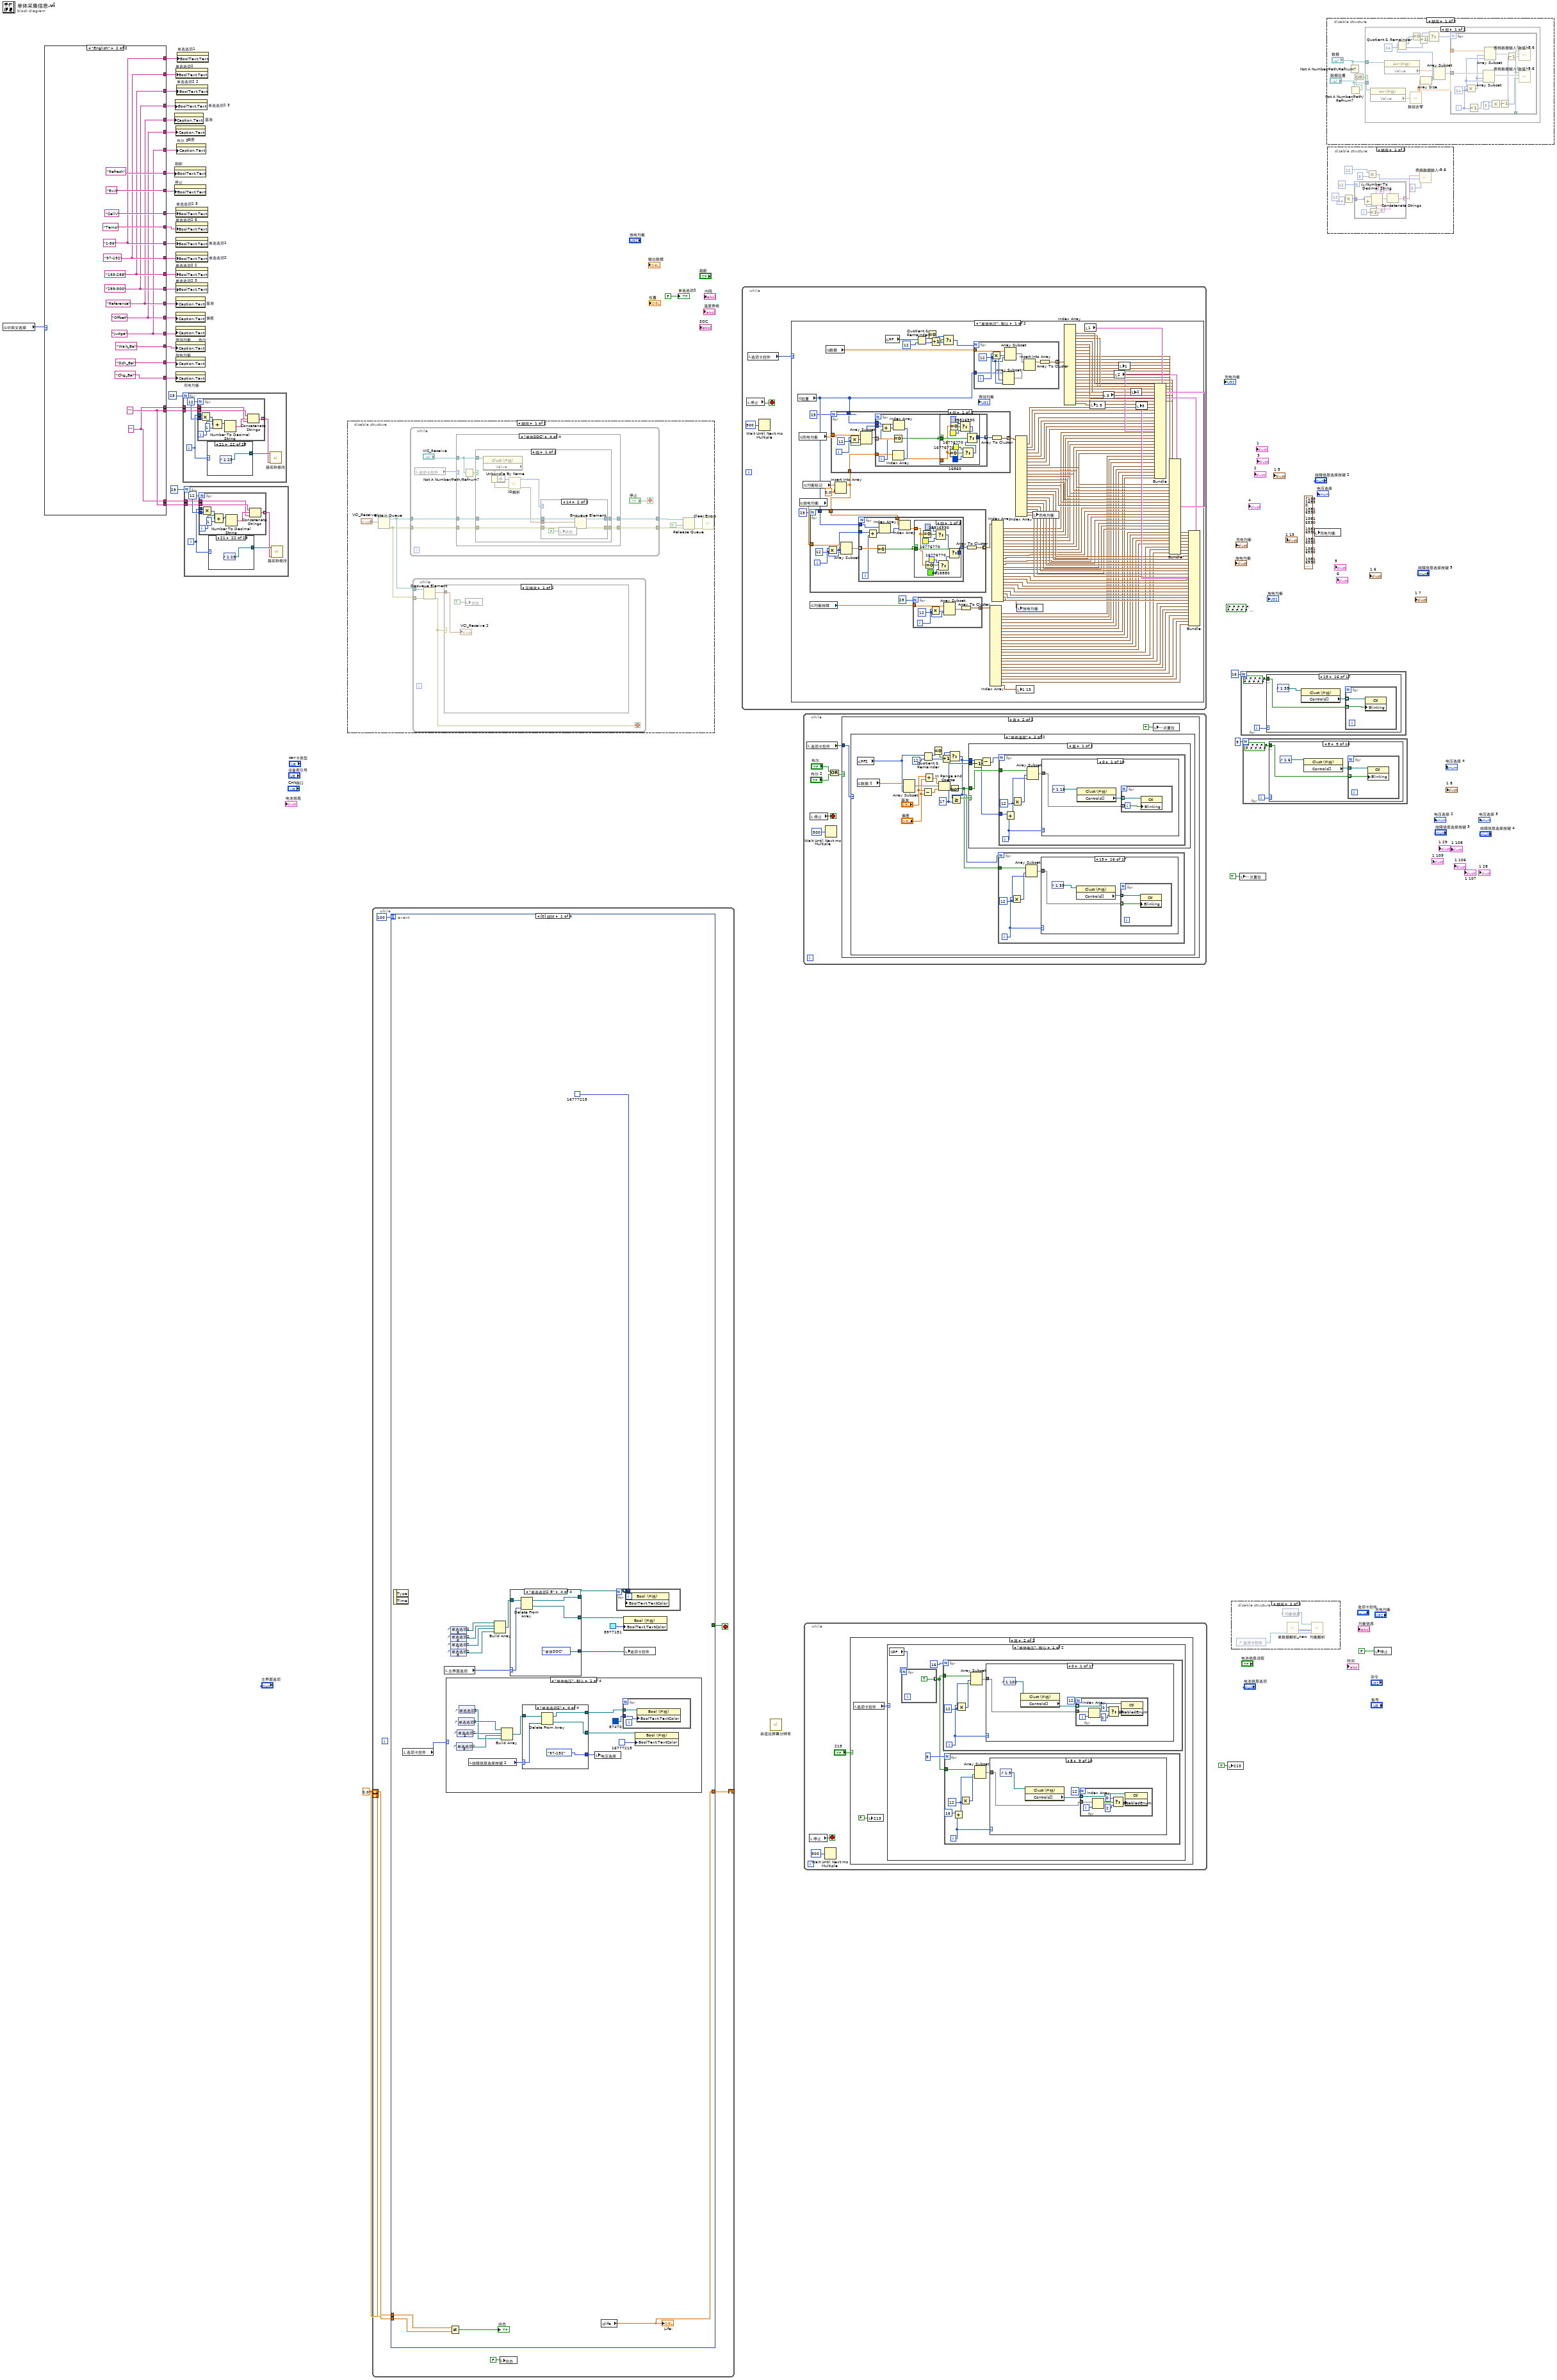
[diagram p0: block diagram]
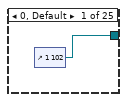
[diagram p2: hidden frame]
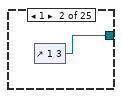
[diagram p3: hidden frame]
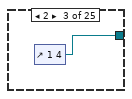
[diagram p4: hidden frame]
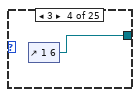
[diagram p5: hidden frame]
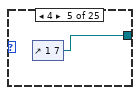
[diagram p6: hidden frame]
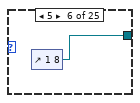
[diagram p7: hidden frame]
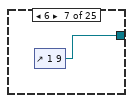
[diagram p8: hidden frame]
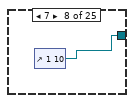
[diagram p9: hidden frame]
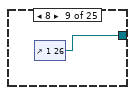
[diagram p10: hidden frame]
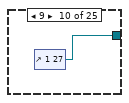
[diagram p11: hidden frame]
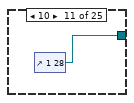
[diagram p12: hidden frame]
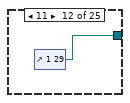
[diagram p13: hidden frame]
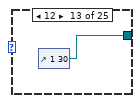
[diagram p14: hidden frame]
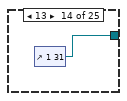
[diagram p15: hidden frame]
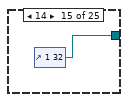
[diagram p16: hidden frame]
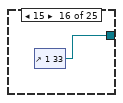
[diagram p17: hidden frame]
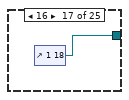
[diagram p18: hidden frame]
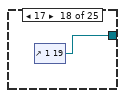
[diagram p19: hidden frame]
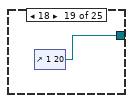
[diagram p20: hidden frame]
diagram:
  w29 = 0.0 ("life")
  (unwired) bool[] [FALSE, FALSE, FALSE, FALSE, FALSE, FALSE, FALSE, FALSE, FALSE, FALSE, FALSE, FALSE, FALSE]
  n1 = global read "中英文全局.vi" "中英文选择"() -> (w28:enum32{"中文", "English"})
  n2 = case shown="\"English\"" w28 {
    tunnel: ["单体电压" "CellV"] -> w27
    tunnel: ["单体温度" "Temp"] -> w26
    tunnel: [w43 w59] -> w25
    tunnel: [w42 w58] -> w24
    tunnel: [w41 w57] -> w23
    tunnel: [w40 w56] -> w22
    tunnel: [w39 w55] -> w21
    tunnel: [w38 w54] -> w20
    tunnel: [w37 w53] -> w19
    tunnel: ["等待均衡" "Wait_Bal"] -> w18
    tunnel: ["放电均衡" "Dch_Bal"] -> w17
    tunnel: ["充电均衡" "Chg_Bal"] -> w16
    tunnel: [w47 w63] -> w14
    tunnel: [w46 w62] -> w13
    tunnel: [w47 w63] -> w11
    tunnel: [w46 w62] -> w12
    tunnel: ["刷新" "Refresh"] -> w9
    tunnel: ["退出" "Exit"] -> w8
    tunnel: [w43 w59] -> w7
    tunnel: [w42 w58] -> w6
    tunnel: [w41 w57] -> w5
    tunnel: [w40 w56] -> w4
    tunnel: [w39 w55] -> w3
    tunnel: [w38 w54] -> w2
    tunnel: [w37 w53] -> w1
    frame "中文", Default {
      w46 = "串"
      w47 = "第"
      w37 = "判定"
      w38 = "偏差"
      w39 = "基准"
      w40 = "289串-300串"
      w41 = "193串-288串"
      w42 = "97串-192串"
      w43 = "1串-96串"
    }
    frame "English" {
      w62 = ""
      w63 = ""
      w53 = "Judge"
      w54 = "Offset"
      w55 = "Reference"
      w56 = "289-300"
      w57 = "193-288"
      w58 = "97-192"
      w59 = "1-96"
    }
  }
  n3 = property on="基准" class="DigNum (严格)"("Caption.Text"=w3) -> ()  [unwired: 2 in, 2 out]
  n4 = property on="刷新" class="Bool (严格)"("BoolText.Text"=w9) -> ()  [unwired: 2 in, 2 out]
  n5 = property on="停止" class="Bool (严格)"("BoolText.Text"=w8) -> ()  [unwired: 2 in, 2 out]
  n6 = property on="单选选项2 3" class="Bool (严格)"("BoolText.Text"=w4) -> ()  [unwired: 2 in, 2 out]
  n7 = property on="偏差" class="DigNum (严格)"("Caption.Text"=w2) -> ()  [unwired: 2 in, 2 out]
  n8 = property on="基准" class="DigNum (严格)"("Caption.Text"=w21) -> ()  [unwired: 2 in, 2 out]
  n9 = property on="偏差" class="DigNum (严格)"("Caption.Text"=w20) -> ()  [unwired: 2 in, 2 out]
  n10 = property on="布尔" class="Bool (严格)"("Caption.Text"=w19) -> ()  [unwired: 2 in, 2 out]
  n11 = property on="等待均衡" class="ColBox"("Caption.Text"=w18) -> ()  [unwired: 2 in, 2 out]
  n12 = property on="放电均衡" class="ColBox"("Caption.Text"=w17) -> ()  [unwired: 2 in, 2 out]
  n13 = property on="充电均衡" class="ColBox"("Caption.Text"=w16) -> ()  [unwired: 2 in, 2 out]
  n14 = property on="单选选项2" class="Bool (严格)"("BoolText.Text"=w6) -> ()  [unwired: 2 in, 2 out]
  n15 = property on="单选选项2 5" class="Bool (严格)"("BoolText.Text"=w27) -> ()  [unwired: 2 in, 2 out]
  n16 = property on="单选选项2 6" class="Bool (严格)"("BoolText.Text"=w26) -> ()  [unwired: 2 in, 2 out]
  n17 = property on="单选选项1" class="Bool (严格)"("BoolText.Text"=w25) -> ()  [unwired: 2 in, 2 out]
  n18 = property on="单选选项2" class="Bool (严格)"("BoolText.Text"=w24) -> ()  [unwired: 2 in, 2 out]
  n19 = property on="单选选项2 2" class="Bool (严格)"("BoolText.Text"=w23) -> ()  [unwired: 2 in, 2 out]
  n20 = property on="单选选项2 3" class="Bool (严格)"("BoolText.Text"=w22) -> ()  [unwired: 2 in, 2 out]
  n21 = property on="单选选项2 2" class="Bool (严格)"("BoolText.Text"=w5) -> ()  [unwired: 2 in, 2 out]
  n22 = property on="布尔 2" class="Bool (严格)"("Caption.Text"=w1) -> ()  [unwired: 2 in, 2 out]
  n23 = property on="单选选项1" class="Bool (严格)"("BoolText.Text"=w7) -> ()  [unwired: 2 in, 2 out]
  n24 = for {
    N: 25 -> [_]
    tunnel: w14 -> [w70]
    tunnel: w13 -> [w69]
    i -> [w71]
    w74 = 12
    n25 = for {
      N: w74 -> [_]
      tunnel: [w108] -> w72 mode=indexing
      tunnel: w71 -> [w105]
      tunnel: w74 -> [w104]
      tunnel: w70 -> [w101]
      tunnel: w69 -> [w100]
      i -> [w107]
      n26 = Multiply(x=w105, y=w104) -> (x*y=w106:i32)
      n27 = Compound Arithmetic op=ADD(w107, w106, 1 ("值")) -> (w102:i32)
      n28 = Number To Decimal String(number=w102) -> (decimal integer string=w109:string)  [unwired: 1 in]
      n29 = Concatenate Strings(w101, w109, w100) -> (w108:string)
    }
    n30 = case shown="21" w71 {
      tunnel: [w75 w76 w77 w78 w79 w80 w81 w82 w83 w84 w85 w86 w87 w88 w89 w90 w91 w92 w93 w94 w95 w96 w97 w98 w99] -> w73
      frame 0, Default {
        n31 = control-ref of="1 102"() -> (w75:refnum<vi>)
      }
      frame 1 {
        n32 = control-ref of="1 3"() -> (w76:refnum<vi>)
      }
      frame 2 {
        n33 = control-ref of="1 4"() -> (w77:refnum<vi>)
      }
      frame 3 {
        n34 = control-ref of="1 6"() -> (w78:refnum<vi>)
      }
      frame 4 {
        n35 = control-ref of="1 7"() -> (w79:refnum<vi>)
      }
      frame 5 {
        n36 = control-ref of="1 8"() -> (w80:refnum<vi>)
      }
      frame 6 {
        n37 = control-ref of="1 9"() -> (w81:refnum<vi>)
      }
      frame 7 {
        n38 = control-ref of="1 10"() -> (w82:refnum<vi>)
      }
      frame 8 {
        n39 = control-ref of="1 26"() -> (w83:refnum<vi>)
      }
      frame 9 {
        n40 = control-ref of="1 27"() -> (w84:refnum<vi>)
      }
      frame 10 {
        n41 = control-ref of="1 28"() -> (w85:refnum<vi>)
      }
      frame 11 {
        n42 = control-ref of="1 29"() -> (w86:refnum<vi>)
      }
      frame 12 {
        n43 = control-ref of="1 30"() -> (w87:refnum<vi>)
      }
      frame 13 {
        n44 = control-ref of="1 31"() -> (w88:refnum<vi>)
      }
      frame 14 {
        n45 = control-ref of="1 32"() -> (w89:refnum<vi>)
      }
      frame 15 {
        n46 = control-ref of="1 33"() -> (w90:refnum<vi>)
      }
      frame 16 {
        n47 = control-ref of="1 18"() -> (w91:refnum<vi>)
      }
      frame 17 {
        n48 = control-ref of="1 19"() -> (w92:refnum<vi>)
      }
      frame 18 {
        n49 = control-ref of="1 20"() -> (w93:refnum<vi>)
      }
      frame 19 {
        n50 = control-ref of="1 21"() -> (w94:refnum<vi>)
      }
      frame 20 {
        n51 = control-ref of="1 22"() -> (w95:refnum<vi>)
      }
      frame 21 {
        n52 = control-ref of="1 23"() -> (w96:refnum<vi>)
      }
      frame 22 {
        n53 = control-ref of="1 24"() -> (w97:refnum<vi>)
      }
      frame 23 {
        n54 = control-ref of="1 25"() -> (w98:refnum<vi>)
      }
      frame 24 {
        n55 = control-ref of="1 5"() -> (w99:refnum<vi>)
      }
    }
    n56 = call "簇名称修改.vi"("输入名称"=w72, "簇引用"=w73) -> ()  [unwired: 10 in]
  }
  n57 = for {
    N: 25 -> [_]
    tunnel: w11 -> [w111]
    tunnel: w12 -> [w110]
    i -> [w112]
    w115 = 12
    n58 = for {
      N: w115 -> [_]
      tunnel: [w149] -> w113 mode=indexing
      tunnel: w112 -> [w146]
      tunnel: w115 -> [w145]
      tunnel: w111 -> [w142]
      tunnel: w110 -> [w141]
      i -> [w148]
      n59 = Multiply(x=w146, y=w145) -> (x*y=w147:i32)
      n60 = Compound Arithmetic op=ADD(w148, w147, 1 ("值")) -> (w143:i32)
      n61 = Number To Decimal String(number=w143) -> (decimal integer string=w150:string)  [unwired: 1 in]
      n62 = Concatenate Strings(w142, w150, w141) -> (w149:string)
    }
    n63 = case shown="21" w112 {
      tunnel: [w116 w117 w118 w119 w120 w121 w122 w123 w124 w125 w126 w127 w128 w129 w130 w131 w132 w133 w134 w135 w136 w137 w138 w139 w140] -> w114
      frame 0, Default {
        n64 = control-ref of="1 102"() -> (w116:refnum<vi>)
      }
      frame 1 {
        n65 = control-ref of="1 3"() -> (w117:refnum<vi>)
      }
      frame 2 {
        n66 = control-ref of="1 4"() -> (w118:refnum<vi>)
      }
      frame 3 {
        n67 = control-ref of="1 6"() -> (w119:refnum<vi>)
      }
      frame 4 {
        n68 = control-ref of="1 7"() -> (w120:refnum<vi>)
      }
      frame 5 {
        n69 = control-ref of="1 8"() -> (w121:refnum<vi>)
      }
      frame 6 {
        n70 = control-ref of="1 9"() -> (w122:refnum<vi>)
      }
      frame 7 {
        n71 = control-ref of="1 10"() -> (w123:refnum<vi>)
      }
      frame 8 {
        n72 = control-ref of="1 26"() -> (w124:refnum<vi>)
      }
      frame 9 {
        n73 = control-ref of="1 27"() -> (w125:refnum<vi>)
      }
      frame 10 {
        n74 = control-ref of="1 28"() -> (w126:refnum<vi>)
      }
      frame 11 {
        n75 = control-ref of="1 29"() -> (w127:refnum<vi>)
      }
      frame 12 {
        n76 = control-ref of="1 30"() -> (w128:refnum<vi>)
      }
      frame 13 {
        n77 = control-ref of="1 31"() -> (w129:refnum<vi>)
      }
      frame 14 {
        n78 = control-ref of="1 32"() -> (w130:refnum<vi>)
      }
      frame 15 {
        n79 = control-ref of="1 33"() -> (w131:refnum<vi>)
      }
      frame 16 {
        n80 = control-ref of="1 18"() -> (w132:refnum<vi>)
      }
      frame 17 {
        n81 = control-ref of="1 19"() -> (w133:refnum<vi>)
      }
      frame 18 {
        n82 = control-ref of="1 20"() -> (w134:refnum<vi>)
      }
      frame 19 {
        n83 = control-ref of="1 21"() -> (w135:refnum<vi>)
      }
      frame 20 {
        n84 = control-ref of="1 22"() -> (w136:refnum<vi>)
      }
      frame 21 {
        n85 = control-ref of="1 23"() -> (w137:refnum<vi>)
      }
      frame 22 {
        n86 = control-ref of="1 24"() -> (w138:refnum<vi>)
      }
      frame 23 {
        n87 = control-ref of="1 25"() -> (w139:refnum<vi>)
      }
      frame 24 {
        n88 = control-ref of="1 6"() -> (w140:refnum<vi>)
      }
    }
    n89 = call "簇名称修改.vi"("输入名称"=w113, "簇引用"=w114) -> ()  [unwired: 10 in]
  }
  n90 = disable-structure shown="禁用" {
    frame Disabled {
      n91 = Obtain Queue(element data type="VCI_Receive") -> (queue out=w156:refnum<queue>, error out=w155:errorcluster)  [unwired: 4 in, 1 out]
      n92 = while {
        tunnel: w156 -> [w167]
        tunnel: w155 -> [w166]
        tunnel: [w165] -> w154
        tunnel: [w164] -> w153
        stop <- "停止" stop-if-true
        n93 = local read "选项卡控件"() -> (w168:enum32{"单体电压", "单体温度", "单体内阻", "单体SOC"})
        n94 = case shown="\"单体SOC\"" w168 {
          tunnel: "VIC_Receive" -> [w172 w196 w220 w244]
          tunnel: w167 -> [w176 w200 w224 w248]
          tunnel: w166 -> [w175 w199 w223 w247]
          tunnel: [w174 w198 w222 w246] -> w165
          tunnel: [w173 w197 w221 w245] -> w164
          frame "单体电压", Default {
            n95 = Not A Number/Path/Refnum?(number/path/refnum=w172) -> (NaN/Path/Refnum?=w171:bool)
            n96 = case shown="假" w171 {
              tunnel: w176 -> [w183 w194]
              tunnel: w175 -> [w182 w193]
              tunnel: [w180 w194] -> w174
              tunnel: [w179 w193] -> w173
              tunnel: w172 -> [w178 _]
              frame False {
                n97 = property class="Clust (严格)"(reference=w178) -> ("Value"=w181:T1)  [unwired: 1 in, 2 out]
                n98 = Unbundle By Name(w181) -> ("ID"=w184:u32)
                n99 = call "ID解析.vi"("ID"=w184) -> ("PDU(1)"=w177:i32)  [unwired: 10 out]
                n100 = case shown="8" w177 {
                  tunnel: w183 -> [w186 w192]
                  tunnel: w182 -> [w185 w191]
                  tunnel: w181 -> [_ w190]
                  tunnel: [w186 w189] -> w180
                  tunnel: [w185 w188] -> w179
                  frame 0, Default {
                  }
                  frame 8 {
                    n101 = local write "状态"(FALSE ("状态")) -> ()
                    n102 = Enqueue Element(queue=w192, element=w190, error in (no error)=w191) -> (queue out=w189:refnum<queue>, error out=w188:errorcluster)  [unwired: 2 out]
                  }
                }
              }
              frame True {
              }
            }
          }
          frame "单体温度" {
            n103 = Not A Number/Path/Refnum?(number/path/refnum=w196) -> (NaN/Path/Refnum?=w195:bool)
            n104 = case shown="假" w195 {
              tunnel: w200 -> [w207 w218]
              tunnel: w199 -> [w206 w217]
              tunnel: [w205 w218] -> w198
              tunnel: [w204 w217] -> w197
              tunnel: w196 -> [w203 _]
              frame False {
                n105 = property class="Clust (严格)"(reference=w203) -> ("Value"=w201:T1)  [unwired: 1 in, 2 out]
                n106 = Unbundle By Name(w201) -> ("ID"=w208:u32)
                n107 = call "ID解析.vi"("ID"=w208) -> ("PDU(1)"=w202:i32)  [unwired: 10 out]
                n108 = case shown="10" w202 {
                  tunnel: w207 -> [w210 w216]
                  tunnel: w206 -> [w209 w215]
                  tunnel: w201 -> [_ w214]
                  tunnel: [w210 w213] -> w205
                  tunnel: [w209 w212] -> w204
                  frame 0, Default {
                  }
                  frame 16 {
                    n109 = local write "状态"(FALSE ("状态")) -> ()
                    n110 = Enqueue Element(queue=w216, element=w214, error in (no error)=w215) -> (queue out=w213:refnum<queue>, error out=w212:errorcluster)  [unwired: 2 out]
                  }
                }
              }
              frame True {
              }
            }
          }
          frame "单体内阻" {
            n111 = Not A Number/Path/Refnum?(number/path/refnum=w220) -> (NaN/Path/Refnum?=w219:bool)
            n112 = case shown="假" w219 {
              tunnel: w224 -> [w231 w242]
              tunnel: w223 -> [w230 w241]
              tunnel: [w228 w242] -> w222
              tunnel: [w227 w241] -> w221
              tunnel: w220 -> [w226 _]
              frame False {
                n113 = property class="Clust (严格)"(reference=w226) -> ("Value"=w229:T1)  [unwired: 1 in, 2 out]
                n114 = Unbundle By Name(w229) -> ("ID"=w232:u32)
                n115 = call "ID解析.vi"("ID"=w232) -> ("PDU(1)"=w225:i32)  [unwired: 10 out]
                n116 = case shown="C" w225 {
                  tunnel: w231 -> [w234 w240]
                  tunnel: w230 -> [w233 w239]
                  tunnel: w229 -> [_ w238]
                  tunnel: [w234 w237] -> w228
                  tunnel: [w233 w236] -> w227
                  frame 0, Default {
                  }
                  frame 12 {
                    n117 = local write "状态"(FALSE ("状态")) -> ()
                    n118 = Enqueue Element(queue=w240, element=w238, error in (no error)=w239) -> (queue out=w237:refnum<queue>, error out=w236:errorcluster)  [unwired: 2 out]
                  }
                }
              }
              frame True {
              }
            }
          }
          frame "单体SOC" {
            n119 = Not A Number/Path/Refnum?(number/path/refnum=w244) -> (NaN/Path/Refnum?=w243:bool)
            n120 = case shown="假" w243 {
              tunnel: w248 -> [w255 w266]
              tunnel: w247 -> [w254 w265]
              tunnel: [w252 w266] -> w246
              tunnel: [w251 w265] -> w245
              tunnel: w244 -> [w250 _]
              frame False {
                n121 = property class="Clust (严格)"(reference=w250) -> ("Value"=w253:T1)  [unwired: 1 in, 2 out]
                n122 = Unbundle By Name(w253) -> ("ID"=w256:u32)
                n123 = call "ID解析.vi"("ID"=w256) -> ("PDU(1)"=w249:i32)  [unwired: 10 out]
                n124 = case shown="14" w249 {
                  tunnel: w255 -> [w258 w264]
                  tunnel: w254 -> [w257 w263]
                  tunnel: w253 -> [_ w262]
                  tunnel: [w258 w261] -> w252
                  tunnel: [w257 w260] -> w251
                  frame 0, Default {
                  }
                  frame 20 {
                    n125 = local write "状态"(FALSE ("状态")) -> ()
                    n126 = Enqueue Element(queue=w264, element=w262, error in (no error)=w263) -> (queue out=w261:refnum<queue>, error out=w260:errorcluster)  [unwired: 2 out]
                  }
                }
              }
              frame True {
              }
            }
          }
        }
      }
      n127 = while {
        tunnel: w156 -> [w160]
        tunnel: w155 -> [w159]
        stop <- w161 stop-if-true
        n128 = Dequeue Element(queue=w160, error in (no error)=w159) -> (element=w158:T1, error out=w161:errorcluster)  [unwired: 3 out]
        n129 = case shown="无错误" w161 {
          tunnel: w158 -> [w162 _]
          frame No Error {
            n130 = local write "状态"(TRUE ("状态")) -> ()
            "VCI_Receive 2" <- w162
          }
          frame Error {
          }
        }
      }
      n131 = Release Queue(queue=w154, force destroy? (F)=TRUE ("强制销毁？(F)"), error in (no error)=w153) -> (error out=w152:errorcluster)  [unwired: 2 out]
      n132 = call <vilib>:"Clear Errors.vi"("error in (no error)"=w152) -> ()  [unwired: 7 out]
    }
    frame Enabled {
    }
  }
  n133 = while {
    shift-right: [w270] -> _
    shift-left: w29 -> [w269]
    shift-left: w29 -> [w268]
    stop <- w271 stop-if-true
    n134 = event shown="[0] 超时" {
      selector: _ -> [_ _ _ _]
      dyn-events: _ -> [_ _ _ _]
      timeout: 100 -> [_ _ _ _]
      tunnel: [_ _ w462 w468] -> w271
      tunnel: [w276 _ _ _] -> w270
      tunnel: w269 -> [w275 _ _ _]
      tunnel: w268 -> [w274 _ _ _]
      event Timeout {
        n135 = event-data() -> ()  [unwired: 3 out]
        n136 = local read "选项卡控件"() -> (w278:enum32{"单体电压", "单体温度", "单体内阻", "单体SOC"})
        n137 = local read "主界面选项"() -> (w288:T3)
        n138 = case shown="\"单体电压\", 默认" w278 {
          frame "单体电压", Default {
            n139 = control-ref of="单选选项2 3"() -> (w290:refnum<vi>)
            n140 = control-ref of="单选选项2 2"() -> (w291:refnum<vi>)
            n141 = control-ref of="单选选项2"() -> (w292:refnum<vi>)
            n142 = control-ref of="单选选项1"() -> (w289:refnum<vi>)
            n143 = local read "故障信息选择按键 2"() -> (w293:enum32{"单选选项2", "单选选项2 2", "单选选项2 3", "单选选项1"})
            n144 = Build Array(w292, w291, w290, w289) -> (w298:refnum<vi>[])
            n145 = case shown="\"单选选项2\"" w293 {
              selector: w293 -> [w305 w310 w315 w320]
              tunnel: [w304 w309 w314 w319] -> w295
              tunnel: [w303 w308 w313 w318] -> w297
              tunnel: w298 -> [w306 w311 w316 w321]
              tunnel: [enum32{"1-96", "97-192", "193-288", "289-300"}."1-96" ("电压选择") enum32{"1-96", "97-192", "193-288", "289-300"}."289-300" ("电压选择") enum32{"1-96", "97-192", "193-288", "289-300"}."193-288" ("电压选择") enum32{"1-96", "97-192", "193-288", "289-300"}."97-192" ("电压选择")] -> w294
              frame "单选选项1", Default {
                n146 = Delete From Array(array=w306, index=w305) -> (deleted portion=w303:refnum<vi>, array with subset deleted=w304:refnum<vi>[])  [unwired: 1 in]
              }
              frame "单选选项2 3" {
                n147 = Delete From Array(array=w311, index=w310) -> (deleted portion=w308:refnum<vi>, array with subset deleted=w309:refnum<vi>[])  [unwired: 1 in]
              }
              frame "单选选项2 2" {
                n148 = Delete From Array(array=w316, index=w315) -> (deleted portion=w313:refnum<vi>, array with subset deleted=w314:refnum<vi>[])  [unwired: 1 in]
              }
              frame "单选选项2" {
                n149 = Delete From Array(array=w321, index=w320) -> (deleted portion=w318:refnum<vi>, array with subset deleted=w319:refnum<vi>[])  [unwired: 1 in]
              }
            }
            n150 = local write "电压选择"(w294) -> ()
            n151 = for {
              tunnel: u32 87470 -> [w301]
              tunnel: w295 -> [w300] mode=indexing
              n152 = property class="Bool (严格)"(reference=w300, "BoolText.TextColor"=w301) -> ()  [unwired: 1 in, 2 out]
            }
            n153 = property class="Bool (严格)"(reference=w297, "BoolText.TextColor"=u32 16777215) -> ()  [unwired: 1 in, 2 out]
          }
          frame "单体温度" {
            n154 = control-ref of="单选选项1"() -> (w326:refnum<vi>)
            n155 = control-ref of="单选选项2"() -> (w324:refnum<vi>)
            n156 = control-ref of="单选选项2 3"() -> (w327:refnum<vi>)
            n157 = control-ref of="单选选项2 2"() -> (w325:refnum<vi>)
            n158 = local read "故障信息选择按键 3"() -> (w323:enum32{"单选选项2", "单选选项2 2", "单选选项2 3", "单选选项1"})
            n159 = Build Array(w324, w325, w327, w326) -> (w331:refnum<vi>[])
            n160 = case shown="\"单选选项2\"" w323 {
              selector: w323 -> [w338 w343 w348 w353]
              tunnel: [w337 w342 w347 w352] -> w328
              tunnel: [w336 w341 w346 w351] -> w330
              tunnel: w331 -> [w339 w344 w349 w354]
              tunnel: [enum32{"1-96", "97-192", "193-288", "289-300"}."1-96" ("电压选择") enum32{"1-96", "97-192", "193-288", "289-300"}."289-300" ("电压选择") enum32{"1-96", "97-192", "193-288", "289-300"}."193-288" ("电压选择") enum32{"1-96", "97-192", "193-288", "289-300"}."97-192" ("电压选择")] -> w322
              frame "单选选项1", Default {
                n161 = Delete From Array(array=w339, index=w338) -> (deleted portion=w336:refnum<vi>, array with subset deleted=w337:refnum<vi>[])  [unwired: 1 in]
              }
              frame "单选选项2 3" {
                n162 = Delete From Array(array=w344, index=w343) -> (deleted portion=w341:refnum<vi>, array with subset deleted=w342:refnum<vi>[])  [unwired: 1 in]
              }
              frame "单选选项2 2" {
                n163 = Delete From Array(array=w349, index=w348) -> (deleted portion=w346:refnum<vi>, array with subset deleted=w347:refnum<vi>[])  [unwired: 1 in]
              }
              frame "单选选项2" {
                n164 = Delete From Array(array=w354, index=w353) -> (deleted portion=w351:refnum<vi>, array with subset deleted=w352:refnum<vi>[])  [unwired: 1 in]
              }
            }
            n165 = local write "电压选择 2"(w322) -> ()
            n166 = for {
              tunnel: u32 87470 -> [w334]
              tunnel: w328 -> [w333] mode=indexing
              n167 = property class="Bool (严格)"(reference=w333, "BoolText.TextColor"=w334) -> ()  [unwired: 1 in, 2 out]
            }
            n168 = property class="Bool (严格)"(reference=w330, "BoolText.TextColor"=u32 16777215) -> ()  [unwired: 1 in, 2 out]
          }
          frame "单体内阻" {
            n169 = control-ref of="单选选项2 3"() -> (w360:refnum<vi>)
            n170 = control-ref of="单选选项2"() -> (w357:refnum<vi>)
            n171 = control-ref of="单选选项2 2"() -> (w358:refnum<vi>)
            n172 = control-ref of="单选选项1"() -> (w359:refnum<vi>)
            n173 = local read "故障信息选择按键 4"() -> (w356:enum32{"单选选项2", "单选选项2 2", "单选选项2 3", "单选选项1"})
            n174 = Build Array(w357, w358, w360, w359) -> (w364:refnum<vi>[])
            n175 = case shown="\"单选选项2\"" w356 {
              selector: w356 -> [w371 w376 w381 w386]
              tunnel: [w370 w375 w380 w385] -> w361
              tunnel: [w369 w374 w379 w384] -> w363
              tunnel: w364 -> [w372 w377 w382 w387]
              tunnel: [enum32{"1-96", "97-192", "193-288", "289-300"}."1-96" ("电压选择") enum32{"1-96", "97-192", "193-288", "289-300"}."289-300" ("电压选择") enum32{"1-96", "97-192", "193-288", "289-300"}."193-288" ("电压选择") enum32{"1-96", "97-192", "193-288", "289-300"}."97-192" ("电压选择")] -> w355
              frame "单选选项1", Default {
                n176 = Delete From Array(array=w372, index=w371) -> (deleted portion=w369:refnum<vi>, array with subset deleted=w370:refnum<vi>[])  [unwired: 1 in]
              }
              frame "单选选项2 3" {
                n177 = Delete From Array(array=w377, index=w376) -> (deleted portion=w374:refnum<vi>, array with subset deleted=w375:refnum<vi>[])  [unwired: 1 in]
              }
              frame "单选选项2 2" {
                n178 = Delete From Array(array=w382, index=w381) -> (deleted portion=w379:refnum<vi>, array with subset deleted=w380:refnum<vi>[])  [unwired: 1 in]
              }
              frame "单选选项2" {
                n179 = Delete From Array(array=w387, index=w386) -> (deleted portion=w384:refnum<vi>, array with subset deleted=w385:refnum<vi>[])  [unwired: 1 in]
              }
            }
            n180 = local write "电压选择 3"(w355) -> ()
            n181 = for {
              tunnel: u32 87470 -> [w367]
              tunnel: w361 -> [w366] mode=indexing
              n182 = property class="Bool (严格)"(reference=w366, "BoolText.TextColor"=w367) -> ()  [unwired: 1 in, 2 out]
            }
            n183 = property class="Bool (严格)"(reference=w363, "BoolText.TextColor"=u32 16777215) -> ()  [unwired: 1 in, 2 out]
          }
          frame "单体SOC" {
            n184 = control-ref of="单选选项1"() -> (w393:refnum<vi>)
            n185 = control-ref of="单选选项2 2"() -> (w391:refnum<vi>)
            n186 = control-ref of="单选选项2 3"() -> (w392:refnum<vi>)
            n187 = control-ref of="单选选项2"() -> (w390:refnum<vi>)
            n188 = local read "故障信息选择按键 5"() -> (w389:enum32{"单选选项2", "单选选项2 2", "单选选项2 3", "单选选项1"})
            n189 = Build Array(w390, w391, w392, w393) -> (w397:refnum<vi>[])
            n190 = case shown="\"单选选项2\"" w389 {
              selector: w389 -> [w404 w409 w414 w419]
              tunnel: [w403 w408 w413 w418] -> w394
              tunnel: [w402 w407 w412 w417] -> w396
              tunnel: w397 -> [w405 w410 w415 w420]
              tunnel: [enum32{"1-96", "97-192", "193-288", "289-300"}."1-96" ("电压选择") enum32{"1-96", "97-192", "193-288", "289-300"}."289-300" ("电压选择") enum32{"1-96", "97-192", "193-288", "289-300"}."193-288" ("电压选择") enum32{"1-96", "97-192", "193-288", "289-300"}."97-192" ("电压选择")] -> w388
              frame "单选选项1", Default {
                n191 = Delete From Array(array=w405, index=w404) -> (deleted portion=w402:refnum<vi>, array with subset deleted=w403:refnum<vi>[])  [unwired: 1 in]
              }
              frame "单选选项2 3" {
                n192 = Delete From Array(array=w410, index=w409) -> (deleted portion=w407:refnum<vi>, array with subset deleted=w408:refnum<vi>[])  [unwired: 1 in]
              }
              frame "单选选项2 2" {
                n193 = Delete From Array(array=w415, index=w414) -> (deleted portion=w412:refnum<vi>, array with subset deleted=w413:refnum<vi>[])  [unwired: 1 in]
              }
              frame "单选选项2" {
                n194 = Delete From Array(array=w420, index=w419) -> (deleted portion=w417:refnum<vi>, array with subset deleted=w418:refnum<vi>[])  [unwired: 1 in]
              }
            }
            n195 = local write "电压选择 4"(w388) -> ()
            n196 = for {
              tunnel: u32 87470 -> [w400]
              tunnel: w394 -> [w399] mode=indexing
              n197 = property class="Bool (严格)"(reference=w399, "BoolText.TextColor"=w400) -> ()  [unwired: 1 in, 2 out]
            }
            n198 = property class="Bool (严格)"(reference=w396, "BoolText.TextColor"=u32 16777215) -> ()  [unwired: 1 in, 2 out]
          }
        }
        n199 = Not Equal?(x=w275, y=w274) -> (x != y?=→"状态":bool)
        n200 = control-ref of="单选选项2 5"() -> (w282:refnum<vi>)
        n201 = control-ref of="单选选项2 6"() -> (w281:refnum<vi>)
        n202 = control-ref of="单选选项2 7"() -> (w280:refnum<vi>)
        n203 = control-ref of="单选选项2 8"() -> (w279:refnum<vi>)
        n204 = Build Array(w282, w281, w280, w279) -> (w283:refnum<vi>[])
        n205 = case shown="\"单选选项2 8\"" w288 {
          selector: w288 -> [w427 w432 w437 w442]
          tunnel: [w426 w431 w436 w441] -> w285
          tunnel: [w425 w430 w435 w440] -> w284
          tunnel: w283 -> [w424 w429 w434 w439]
          tunnel: [enum32{"单体电压", "单体温度", "单体内阻", "单体SOC"}."单体电压" ("选项卡控件") enum32{"单体电压", "单体温度", "单体内阻", "单体SOC"}."单体温度" ("选项卡控件") enum32{"单体电压", "单体温度", "单体内阻", "单体SOC"}."单体内阻" ("选项卡控件") enum32{"单体电压", "单体温度", "单体内阻", "单体SOC"}."单体SOC" ("选项卡控件")] -> w277
          frame "单选选项2 5" {
            n206 = Delete From Array(array=w424, index=w427) -> (deleted portion=w425:refnum<vi>, array with subset deleted=w426:refnum<vi>[])  [unwired: 1 in]
          }
          frame "单选选项2 6" {
            n207 = Delete From Array(array=w429, index=w432) -> (deleted portion=w430:refnum<vi>, array with subset deleted=w431:refnum<vi>[])  [unwired: 1 in]
          }
          frame "单选选项2 7" {
            n208 = Delete From Array(array=w434, index=w437) -> (deleted portion=w435:refnum<vi>, array with subset deleted=w436:refnum<vi>[])  [unwired: 1 in]
          }
          frame "单选选项2 8" {
            n209 = Delete From Array(array=w439, index=w442) -> (deleted portion=w440:refnum<vi>, array with subset deleted=w441:refnum<vi>[])  [unwired: 1 in]
          }
        }
        n210 = global read "EV05全局变量1.vi" "life"() -> (w276:dbl)
        "Life:" <- w276
        n211 = for {
          tunnel: w285 -> [w422] mode=indexing
          tunnel: u32 16777215 -> [w421]
          n212 = property class="Bool (严格)"(reference=w422, "BoolText.TextColor"=w421) -> ()  [unwired: 1 in, 2 out]
        }
        n213 = property class="Bool (严格)"(reference=w284, "BoolText.TextColor"=u32 8977151) -> ()  [unwired: 1 in, 2 out]
        n214 = local write "选项卡控件"(w277) -> ()
      }
      event "刷新": Value Change {
        n215 = event-data() -> ("NewVal"=w443:bool)  [unwired: 6 out]
        n216 = case shown="真" w443 {
          frame False {
          }
          frame True {
            n217 = local read "选项卡控件"() -> (w445:enum32{"单体电压", "单体温度", "单体内阻", "单体SOC"})
            n218 = case shown="\"单体温度\"" w445 {
              frame "单体电压", Default {
                n219 = Initialize Array(0.0 ("(hi.lo)"), 300 ("维数大小")) -> (w447:dbl[])
                n220 = Initialize Array(0 ("(hi.lo)"), 300 ("维数大小")) -> (w446:i32[])
                n221 = global write "单体信息全局.vi" "SOC位置"(w446) -> ()
                n222 = global write "单体信息全局.vi" "数据"(w447) -> ()
                n223 = global write "单体信息全局.vi" "充电均衡"(w447) -> ()
                n224 = global write "单体信息全局.vi" "放电均衡"(w447) -> ()
                n225 = global write "单体信息全局.vi" "位置"(w446) -> ()
                n226 = local write "1 5"(T7 {"第289串"=0.0, "第290串"=0.0, "第291串"=0.0, "第292串"=0.0, "第293串"=0.0, "第294串"=0.0, "第295串"=0.0, "第296串"=0.0, "第297串"=0.0, "第298串"=0.0, "第299串"=0.0, "第300串"=0.0, "第一串 2"=0.0, "第一串 4"=0.0, "第一串 6"=0.0, "第一串 8"=0.0, "第一串 10"=0.0, "第一串 12"=0.0, "第一串 14"=0.0, "第一串 16"=0.0, "第一串 18"=0.0, "第一串 20"=0.0, "第一串 22"=0.0, "第一串 24"=0.0} ("1 5")) -> ()
              }
              frame "单体温度" {
                w460 = T13 {"1 3"={"第13串"=0.0, "第14串"=0.0, "第15串"=0.0, "第16串"=0.0, "第17串"=0.0, "第18串"=0.0, "第19串"=0.0, "第20串"=0.0, "第21串"=0.0, "第22串"=0.0, "第23串"=0.0, "第24串"=0.0, "第一串 2"=0.0, "第一串 4"=0.0, "第一串 6"=0.0, "第一串 8"=0.0, "第一串 10"=0.0, "第一串 12"=0.0, "第一串 14"=0.0, "第一串 16"=0.0, "第一串 18"=0.0, "第一串 20"=0.0, "第一串 22"=0.0, "第一串 24"=0.0}, "1 4"={"第25串"=0.0, "第26串"=0.0, "第27串"=0.0, "第28串"=0.0, "第29串"=0.0, "第30串"=0.0, "第31串"=0.0, "第32串"=0.0, "第33串"=0.0, "第34串"=0.0, "第35串"=0.0, "第36串"=0.0, "第一串 2"=0.0, "第一串 4"=0.0, "第一串 6"=0.0, "第一串 8"=0.0, "第一串 10"=0.0, "第一串 12"=0.0, "第一串 14"=0.0, "第一串 16"=0.0, "第一串 18"=0.0, "第一串 20"=0.0, "第一串 22"=0.0, "第一串 24"=0.0}, "1 6"={"第37串"=0.0, "第38串"=0.0, "第39串"=0.0, "第40串"=0.0, "第41串"=0.0, "第42串"=0.0, "第43串"=0.0, "第44串"=0.0, "第45串"=0.0, "第46串"=0.0, "第47串"=0.0, "第48串"=0.0, "第一串 2"=0.0, "第一串 4"=0.0, "第一串 6"=0.0, "第一串 8"=0.0, "第一串 10"=0.0, "第一串 12"=0.0, "第一串 14"=0.0, "第一串 16"=0.0, "第一串 18"=0.0, "第一串 20"=0.0, "第一串 22"=0.0, "第一串 24"=0.0}, "1 7"={"第49串"=0.0, "第50串"=0.0, "第51串"=0.0, "第52串"=0.0, "第53串"=0.0, "第54串"=0.0, "第55串"=0.0, "第56串"=0.0, "第57串"=0.0, "第58串"=0.0, "第59串"=0.0, "第60串"=0.0, "第一串 2"=0.0, "第一串 4"=0.0, "第一串 6"=0.0, "第一串 8"=0.0, "第一串 10"=0.0, "第一串 12"=0.0, "第一串 14"=0.0, "第一串 16"=0.0, "第一串 18"=0.0, "第一串 20"=0.0, "第一串 22"=0.0, "第一串 24"=0.0}, "1 8"={"第61串"=0.0, "第62串"=0.0, "第63串"=0.0, "第64串"=0.0, "第65串"=0.0, "第66串"=0.0, "第67串"=0.0, "第68串"=0.0, "第69串"=0.0, "第70串"=0.0, "第71串"=0.0, "第72串"=0.0, "第一串 2"=0.0, "第一串 4"=0.0, "第一串 6"=0.0, "第一串 8"=0.0, "第一串 10"=0.0, "第一串 12"=0.0, "第一串 14"=0.0, "第一串 16"=0.0, "第一串 18"=0.0, "第一串 20"=0.0, "第一串 22"=0.0, "第一串 24"=0.0}, "1 9"={"第73串"=0.0, "第74串"=0.0, "第75串"=0.0, "第76串"=0.0, "第77串"=0.0, "第78串"=0.0, "第79串"=0.0, "第80串"=0.0, "第81串"=0.0, "第82串"=0.0, "第83串"=0.0, "第84串"=0.0, "第一串 2"=0.0, "第一串 4"=0.0, "第一串 6"=0.0, "第一串 8"=0.0, "第一串 10"=0.0, "第一串 12"=0.0, "第一串 14"=0.0, "第一串 16"=0.0, "第一串 18"=0.0, "第一串 20"=0.0, "第一串 22"=0.0, "第一串 24"=0.0}, "1 10"={"第85串"=0.0, "第86串"=0.0, "第87串"=0.0, "第88串"=0.0, "第89串"=0.0, "第90串"=0.0, "第91串"=0.0, "第92串"=0.0, "第93串"=0.0, "第94串"=0.0, "第95串"=0.0, "第96串"=0.0, "第一串 2"=0.0, "第一串 4"=0.0, "第一串 6"=0.0, "第一串 8"=0.0, "第一串 10"=0.0, "第一串 12"=0.0, "第一串 14"=0.0, "第一串 16"=0.0, "第一串 18"=0.0, "第一串 20"=0.0, "第一串 22"=0.0, "第一串 24"=0.0}, "1 102"={"第1串"=0.0, "第2串"=0.0, "第3串"=0.0, "第4串"=0.0, "第5串"=0.0, "第6串"=0.0, "第7串"=0.0, "第8串"=0.0, "第9串"=0.0, "第10串"=0.0, "第11串"=0.0, "第12串"=0.0, "第一串 2"=0.0, "第一串 4"=0.0, "第一串 6"=0.0, "第一串 8"=0.0, "第一串 10"=0.0, "第一串 12"=0.0, "第一串 14"=0.0, "第一串 16"=0.0, "第一串 18"=0.0, "第一串 20"=0.0, "第一串 22"=0.0, "第一串 24"=0.0}} ("1 108")
                n227 = Initialize Array(0.0 ("(hi.lo)"), 300 ("维数大小")) -> (w456:dbl[])
                n228 = Initialize Array(0 ("(hi.lo)"), 300 ("维数大小")) -> (w453:i32[])
                n229 = global write "单体信息全局.vi" "数据 2"(w456) -> ()
                n230 = global write "单体信息全局.vi" "位置 2"(w453) -> ()
                n231 = local write "1 6"(T7 {"第289串"=0.0, "第290串"=0.0, "第291串"=0.0, "第292串"=0.0, "第293串"=0.0, "第294串"=0.0, "第295串"=0.0, "第296串"=0.0, "第297串"=0.0, "第298串"=0.0, "第299串"=0.0, "第300串"=0.0, "第一串 2"=0.0, "第一串 4"=0.0, "第一串 6"=0.0, "第一串 8"=0.0, "第一串 10"=0.0, "第一串 12"=0.0, "第一串 14"=0.0, "第一串 16"=0.0, "第一串 18"=0.0, "第一串 20"=0.0, "第一串 22"=0.0, "第一串 24"=0.0} ("1 5")) -> ()
                n232 = local write "4"(w460) -> ()
                n233 = local write "5"(w460) -> ()
                n234 = local write "6"(w460) -> ()
              }
            }
            n235 = local write "213"(TRUE ("213")) -> ()
          }
        }
      }
      event "停止": Value Change {
        n236 = event-data() -> ("NewVal"=w462:bool)  [unwired: 6 out]
        n237 = disable-structure shown="启用" {
          disable-tunnel: w462 -> [_ w467]
          frame Enabled {
            n238 = property class="VI"("FP.State"=T14."Hidden" ("前面板窗口:状态")) -> (reference out=w464:refnum<vi>, error out=w463:errorcluster)  [unwired: 2 in]
            n239 = property class="VI"(reference=w464, error in=w463, "Front Panel.Open"=FALSE ("前面板窗口:打开")) -> ()  [unwired: 2 out]
          }
          frame Disabled {
            n240 = Stop(stop? (T)=w467) -> ()
          }
        }
        n241 = local write "停止"(TRUE ("停止")) -> ()
      }
      event Panel Close? {
        w468 = TRUE ("停止")
        n242 = event-data() -> ()  [unwired: 5 out]
        n243 = disable-structure shown="启用" {
          disable-tunnel: w468 -> [_ w474]
          frame Enabled {
            n244 = property class="VI"("FP.State"=T14."Hidden" ("前面板窗口:状态")) -> (reference out=w471:refnum<vi>, error out=w470:errorcluster)  [unwired: 2 in]
            n245 = property class="VI"(reference=w471, error in=w470, "Front Panel.Open"=FALSE ("前面板窗口:打开")) -> ()  [unwired: 2 out]
          }
          frame Disabled {
            n246 = Stop(stop? (T)=w474) -> ()
          }
        }
        n247 = local write "停止"(w468) -> ()
        n248 = event-data("Discard?"=FALSE ("放弃？")) -> ()  [unwired: 1 in, 1 out]
      }
    }
    n249 = local write "状态"(FALSE ("状态")) -> ()
  }
  n250 = while {
    stop <- w475 stop-if-true
    n251 = local read "停止"() -> (w475:bool)
    n252 = local read "选项卡控件"() -> (w477:enum32{"单体电压", "单体温度", "单体内阻", "单体SOC"})
    n253 = Wait Until Next ms Multiple(millisecond multiple=u32 500 ("毫秒倍数")) -> ()  [unwired: 1 out]
    n254 = case shown="\"单体电压\", 默认" w477 {
      frame "单体电压", Default {
        w479 = 0.0 ("新元素/子数组")
        n255 = global read "单体信息全局.vi" "位置"() -> (w485:i32[])
        n256 = global read "单体信息全局.vi" "充电均衡"() -> (w567:dbl[])
        n257 = global read "单体信息全局.vi" "放电均衡"() -> (w540:dbl[])
        n258 = global read "从板全局变量.vi" "均衡标记"() -> (w481:dbl[])
        n259 = global read "单体信息全局.vi" "均衡故障"() -> (w514:dbl[])
        n260 = global read "单体信息全局.vi" "数据"() -> (w568:dbl[])
        n261 = Insert Into Array(array=w481, index=w479, new element=w479) -> (w480:dbl[])
        n262 = for {
          N: 25 -> [_]
          tunnel: w540 -> [w620]
          tunnel: [w616] -> w539 mode=indexing
          tunnel: w480 -> [w612]
          tunnel: w485 -> [w613]
          i -> [w615]
          w619 = 12 ("y")
          n263 = Multiply(x=w615, y=w619) -> (x*y=w614:i32)
          n264 = Array Subset(array=w620, index=w614, length=w619) -> (w618:dbl[])
          n265 = for {
            tunnel: w618 -> [w629] mode=indexing
            tunnel: [w630] -> w617 mode=indexing
            tunnel: w614 -> [w628]
            tunnel: w613 -> [w626]
            tunnel: w612 -> [w624]
            i -> [w627]
            n266 = Add(x=w628, y=w627) -> (x+y=w625:i32)
            n267 = Equal To 0?(x=w629) -> (x = 0?=w621:bool)
            n268 = Index Array(array=w626, index=w625) -> (element=w623:i32)
            n269 = Index Array(array=w624, index=w623) -> (element=w622:dbl)
            n270 = case shown="假" w621 {
              tunnel: w621 -> [w641 _]
              tunnel: [w640 u32 13816530] -> w630
              tunnel: w622 -> [w631 _]
              frame False {
                n271 = Equal To 0?(x=w631) -> (x = 0?=w639:bool)
                n272 = Equal To 0?(x=w631) -> (x = 0?=w635:bool)
                n273 = Select(t=u32 13816530, s=w639, f=u32 16776770) -> (s? t:f=w636:u32)
                n274 = Select(t=u32 16776770, s=w635, f=u32 6618880) -> (s? t:f=w633:u32)
                n275 = Select(t=w636, s=w641, f=w633) -> (s? t:f=w640:u32)
              }
              frame True {
              }
            }
          }
          n276 = Array To Cluster(array=w617) -> (cluster=w616:T15)
        }
        n277 = for {
          N: 25 -> [_]
          tunnel: w567 -> [w651]
          tunnel: [w647] -> w566 mode=indexing
          tunnel: w480 -> [w643]
          tunnel: w485 -> [w644]
          i -> [w646]
          w650 = 12 ("y")
          n278 = Multiply(x=w646, y=w650) -> (x*y=w645:i32)
          n279 = Array Subset(array=w651, index=w645, length=w650) -> (w649:dbl[])
          n280 = for {
            tunnel: w649 -> [w660] mode=indexing
            tunnel: [w661] -> w648 mode=indexing
            tunnel: w645 -> [w659]
            tunnel: w644 -> [w656]
            tunnel: w643 -> [w653]
            i -> [w658]
            n281 = Add(x=w659, y=w658) -> (x+y=w657:i32)
            n282 = Equal To 0?(x=w660) -> (x = 0?=w652:bool)
            n283 = Index Array(array=w656, index=w657) -> (element=w655:i32)
            n284 = Index Array(array=w653, index=w655) -> (element=w654:dbl)
            n285 = case shown="假" w652 {
              tunnel: w652 -> [w672 _]
              tunnel: [w671 u32 13816530] -> w661
              tunnel: w654 -> [w662 _]
              frame False {
                n286 = Equal To 0?(x=w662) -> (x = 0?=w670:bool)
                n287 = Equal To 0?(x=w662) -> (x = 0?=w667:bool)
                n288 = Select(t=u32 13816530, s=w667, f=u32 16776770) -> (s? t:f=w665:u32)
                n289 = Select(t=u32 16776770, s=w670, f=u32 16860) -> (s? t:f=w669:u32)
                n290 = Select(t=w665, s=w672, f=w669) -> (s? t:f=w671:u32)
              }
              frame True {
              }
            }
          }
          n291 = Array To Cluster(array=w648) -> (cluster=w647:T15)
        }
        n292 = global read "单体信息全局.vi" "PF"() -> (w478:i32)
        n293 = for {
          N: 25 -> [_]
          tunnel: w514 -> [w611]
          tunnel: [w607] -> w513 mode=indexing
          i -> [w610]
          w608 = 12 ("y")
          n294 = Multiply(x=w610, y=w608) -> (x*y=w609:i32)
          n295 = Array Subset(array=w611, index=w609, length=w608) -> (w606:dbl[])
          n296 = Array To Cluster(array=w606) -> (cluster=w607:T16)
        }
        n297 = Quotient & Remainder(x=w478, y=12) -> (x-y*floor(x/y)=w572:i32, floor(x/y)=w570:i32)
        n298 = Equal To 0?(x=w572) -> (x = 0?=w571:bool)
        n299 = Increment(x=w570) -> (x+1=w569:i32)
        n300 = Select(t=w570, s=w571, f=w569) -> (s? t:f=w484:i32)
        n301 = for {
          N: w484 -> [_]
          tunnel: w568 -> [w682]
          tunnel: w485 -> [w674]
          tunnel: [w675] -> w604 mode=indexing
          i -> [w681]
          w679 = 12 ("y")
          n302 = Multiply(x=w681, y=w679) -> (x*y=w680:i32)
          n303 = Array Subset(array=w674, index=w680, length=w679) -> (w677:i32[])
          n304 = Array Subset(array=w682, index=w680, length=w679) -> (w678:dbl[])
          n305 = Insert Into Array(array=w678, new element=w677) -> (w676:dbl[])  [unwired: 1 in]
          n306 = Array To Cluster(array=w676) -> (cluster=w675:T17)
        }
        n307 = Index Array(array=w513) -> (element #1=w512:T16, element #2=w511:T16, element #3=w510:T16, element #4=w509:T16, element #5=w508:T16, element #6=w507:T16, element #7=w506:T16, element #8=w505:T16, element #9=w504:T16, element #10=w503:T16, element #11=w502:T16, element #12=w501:T16, element #13=w500:T16, element #14=w499:T16, element #15=w498:T16, element #16=w497:T16, element #17=w496:T16, element #18=w495:T16, element #19=w494:T16, element #20=w493:T16, element #21=w492:T16, element #22=w491:T16, element #23=w490:T16, element #24=w489:T16, element #25=w488:T16)  [unwired: 25 in]
        n308 = Index Array(array=w539) -> (element #1=w538:T15, element #2=w537:T15, element #3=w536:T15, element #4=w535:T15, element #5=w534:T15, element #6=w533:T15, element #7=w532:T15, element #8=w531:T15, element #9=w530:T15, element #10=w529:T15, element #11=w528:T15, element #12=w527:T15, element #13=w526:T15, element #14=w525:T15, element #15=w524:T15, element #16=w523:T15, element #17=w522:T15, element #18=w521:T15, element #19=w520:T15, element #20=w519:T15, element #21=w518:T15, element #22=w517:T15, element #23=w516:T15, element #24=w515:T15, element #25=w487:T15)  [unwired: 25 in]
        n309 = Index Array(array=w566) -> (element #1=w565:T15, element #2=w564:T15, element #3=w563:T15, element #4=w562:T15, element #5=w561:T15, element #6=w560:T15, element #7=w559:T15, element #8=w558:T15, element #9=w557:T15, element #10=w556:T15, element #11=w555:T15, element #12=w554:T15, element #13=w553:T15, element #14=w552:T15, element #15=w551:T15, element #16=w550:T15, element #17=w549:T15, element #18=w548:T15, element #19=w547:T15, element #20=w546:T15, element #21=w545:T15, element #22=w544:T15, element #23=w543:T15, element #24=w542:T15, element #25=w541:T15)  [unwired: 25 in]
        n310 = local write "1 13"(w488) -> ()
        n311 = local write "放电均衡"(w487) -> ()
        n312 = local write "充电均衡"(w541) -> ()
        n313 = Index Array(array=w604) -> (element #1=w603:T17, element #2=w602:T17, element #3=w601:T17, element #4=w600:T17, element #5=w599:T17, element #6=w598:T17, element #7=w597:T17, element #8=w596:T17, element #9=w592:T17, element #10=w591:T17, element #11=w590:T17, element #12=w589:T17, element #13=w588:T17, element #14=w587:T17, element #15=w586:T17, element #16=w585:T17, element #17=w582:T17, element #18=w581:T17, element #19=w580:T17, element #20=w579:T17, element #21=w578:T17, element #22=w577:T17, element #23=w576:T17, element #24=w575:T17, element #25=w574:T17)  [unwired: 25 in]
        n314 = local read "1"() -> (w605:T4)
        n315 = local write "1 5"(w574) -> ()
        n316 = local read "3"() -> (w583:T6)
        n317 = local read "2"() -> (w594:T5)
        n318 = Bundle(cluster=w605, "1 102"=w603, "1 3"=w602, "1 4"=w601, "1 6"=w600, "1 7"=w599, "1 8"=w598, "1 9"=w597, "1 10"=w596, "1 12"=w565, "1 28"=w564, "1 25"=w563, "1 31"=w562, "1 16"=w561, "1 19"=w560, "1 22"=w559, "1 34"=w558, "1 11"=w538, "1 27"=w537, "1 24"=w536, "1 30"=w535, "1 15"=w534, "1 18"=w533, "1 21"=w532, "1 33"=w531, "1 13"=w512, "1 26"=w511, "1 23"=w510, "1 29"=w509, "1 14"=w508, "1 17"=w507, "1 20"=w506, "1 32"=w505) -> (w595:T4)
        n319 = local write "1"(w595) -> ()
        n320 = Bundle(cluster=w594, "1 26"=w592, "1 27"=w591, "1 28"=w590, "1 29"=w589, "1 30"=w588, "1 31"=w587, "1 32"=w586, "1 33"=w585, "1 16"=w557, "1 44"=w556, "1 36"=w555, "1 47"=w554, "1 19"=w553, "1 38"=w552, "1 41"=w551, "1 50"=w550, "1 15"=w530, "1 43"=w529, "1 35"=w528, "1 46"=w527, "1 18"=w526, "1 37"=w525, "1 40"=w524, "1 49"=w523, "1 14"=w504, "1 42"=w503, "1 34"=w502, "1 45"=w501, "1 17"=w500, "1 20"=w499, "1 39"=w498, "1 48"=w497) -> (w593:T5)
        n321 = local write "2"(w593) -> ()
        n322 = Bundle(cluster=w583, "1 18"=w582, "1 19"=w581, "1 20"=w580, "1 21"=w579, "1 22"=w578, "1 23"=w577, "1 24"=w576, "1 25"=w575, "1 12"=w549, "1 39"=w548, "1 28"=w547, "1 42"=w546, "1 16"=w545, "1 30"=w544, "1 33"=w543, "1 36"=w542, "1 11"=w522, "1 38"=w521, "1 27"=w520, "1 41"=w519, "1 15"=w518, "1 29"=w517, "1 32"=w516, "1 35"=w515, "1 13"=w496, "1 37"=w495, "1 26"=w494, "1 40"=w493, "1 14"=w492, "1 17"=w491, "1 31"=w490, "1 34"=w489) -> (w584:T6)
        n323 = local write "3"(w584) -> ()
      }
      frame "单体温度" {
        n324 = Wait Until Next ms Multiple(millisecond multiple=u32 500 ("毫秒倍数")) -> ()  [unwired: 1 out]
        n325 = global read "单体信息全局.vi" "位置 2"() -> (w685:i32[])
        n326 = global read "单体信息全局.vi" "PF2"() -> (w683:i32)
        n327 = global read "单体信息全局.vi" "数据 2"() -> (w686:dbl[])
        n328 = Quotient & Remainder(x=w683, y=12) -> (x-y*floor(x/y)=w691:i32, floor(x/y)=w689:i32)
        n329 = Equal To 0?(x=w691) -> (x = 0?=w690:bool)
        n330 = Increment(x=w689) -> (x+1=w688:i32)
        n331 = Select(t=w689, s=w690, f=w688) -> (s? t:f=w687:i32)
        n332 = for {
          N: w687 -> [_]
          tunnel: w686 -> [w733]
          tunnel: w685 -> [w725]
          tunnel: [w726] -> w723 mode=indexing
          i -> [w732]
          w730 = 12 ("y")
          n333 = Multiply(x=w732, y=w730) -> (x*y=w731:i32)
          n334 = Array Subset(array=w725, index=w731, length=w730) -> (w728:i32[])
          n335 = Array Subset(array=w733, index=w731, length=w730) -> (w729:dbl[])
          n336 = Insert Into Array(array=w729, new element=w728) -> (w727:dbl[])  [unwired: 1 in]
          n337 = Array To Cluster(array=w727) -> (cluster=w726:T17)
        }
        n338 = Index Array(array=w723) -> (element #1=w722:T17, element #2=w721:T17, element #3=w720:T17, element #4=w719:T17, element #5=w718:T17, element #6=w717:T17, element #7=w716:T17, element #8=w715:T17, element #9=w711:T17, element #10=w710:T17, element #11=w709:T17, element #12=w708:T17, element #13=w707:T17, element #14=w706:T17, element #15=w705:T17, element #16=w704:T17, element #17=w701:T17, element #18=w700:T17, element #19=w699:T17, element #20=w698:T17, element #21=w697:T17, element #22=w696:T17, element #23=w695:T17, element #24=w694:T17, element #25=w693:T17)  [unwired: 25 in]
        n339 = local write "1 6"(w693) -> ()
        n340 = local read "4"() -> (w724:T10)
        n341 = Bundle(cluster=w724, "1 102"=w722, "1 3"=w721, "1 4"=w720, "1 6"=w719, "1 7"=w718, "1 8"=w717, "1 9"=w716, "1 10"=w715) -> (w714:T10)
        n342 = local read "6"() -> (w702:T12)
        n343 = local read "5"() -> (w713:T11)
        n344 = Bundle(cluster=w713, "1 26"=w711, "1 27"=w710, "1 28"=w709, "1 29"=w708, "1 30"=w707, "1 31"=w706, "1 32"=w705, "1 33"=w704) -> (w712:T11)
        n345 = Bundle(cluster=w702, "1 18"=w701, "1 19"=w700, "1 20"=w699, "1 21"=w698, "1 22"=w697, "1 23"=w696, "1 24"=w695, "1 25"=w694) -> (w703:T12)
        n346 = local write "4"(w714) -> ()
        n347 = local write "5"(w712) -> ()
        n348 = local write "6"(w703) -> ()
      }
    }
  }
  n349 = call "自适应屏幕分辨率.vi"() -> ()  [unwired: 16 in]
  n350 = while {
    stop <- w738 stop-if-true
    n351 = local read "选项卡控件"() -> (w737:enum32{"单体电压", "单体温度", "单体内阻", "单体SOC"})
    n352 = local read "停止"() -> (w738:bool)
    n353 = Wait Until Next ms Multiple(millisecond multiple=u32 500 ("毫秒倍数")) -> ()  [unwired: 1 out]
    n354 = Or(x="布尔", y="布尔 2") -> (x .or. y?=w736:bool)
    n355 = case shown="真" w736 {
      tunnel: w737 -> [w740 w1007]
      frame False {
        n356 = case shown="真" "一次置位" {
          tunnel: w740 -> [_ w742]
          frame False {
          }
          frame True {
            n357 = case shown="\"单体温度\"" w742 {
              frame "单体电压", Default {
                n358 = for {
                  N: 9 -> [_]
                  i -> [w828]
                  n359 = case shown="0" w828 {
                    tunnel: bool[] [FALSE, FALSE, FALSE, FALSE, FALSE, FALSE, FALSE, FALSE, FALSE, FALSE, FALSE, FALSE, FALSE] -> [w831 w836 w841 w846 w851 w856 w861 w866 w871 _]
                    frame 0 {
                      n360 = control-ref of="1 18"() -> (w830:refnum<vi>)
                      n361 = property class="Clust (严格)"(reference=w830) -> ("Controls[]"=w832:refnum<vi>[])  [unwired: 1 in, 2 out]
                      n362 = for {
                        tunnel: w832 -> [w833] mode=indexing
                        tunnel: w831 -> [w834] mode=indexing
                        n363 = property class="Ctl"(reference=w833, "Blinking"=w834) -> ()  [unwired: 1 in, 2 out]
                      }
                    }
                    frame 1 {
                      n364 = control-ref of="1 19"() -> (w835:refnum<vi>)
                      n365 = property class="Clust (严格)"(reference=w835) -> ("Controls[]"=w837:refnum<vi>[])  [unwired: 1 in, 2 out]
                      n366 = for {
                        tunnel: w837 -> [w838] mode=indexing
                        tunnel: w836 -> [w839] mode=indexing
                        n367 = property class="Ctl"(reference=w838, "Blinking"=w839) -> ()  [unwired: 1 in, 2 out]
                      }
                    }
                    frame 2 {
                      n368 = control-ref of="1 20"() -> (w840:refnum<vi>)
                      n369 = property class="Clust (严格)"(reference=w840) -> ("Controls[]"=w842:refnum<vi>[])  [unwired: 1 in, 2 out]
                      n370 = for {
                        tunnel: w842 -> [w843] mode=indexing
                        tunnel: w841 -> [w844] mode=indexing
                        n371 = property class="Ctl"(reference=w843, "Blinking"=w844) -> ()  [unwired: 1 in, 2 out]
                      }
                    }
                    frame 3 {
                      n372 = control-ref of="1 21"() -> (w845:refnum<vi>)
                      n373 = property class="Clust (严格)"(reference=w845) -> ("Controls[]"=w847:refnum<vi>[])  [unwired: 1 in, 2 out]
                      n374 = for {
                        tunnel: w847 -> [w848] mode=indexing
                        tunnel: w846 -> [w849] mode=indexing
                        n375 = property class="Ctl"(reference=w848, "Blinking"=w849) -> ()  [unwired: 1 in, 2 out]
                      }
                    }
                    frame 4 {
                      n376 = control-ref of="1 22"() -> (w850:refnum<vi>)
                      n377 = property class="Clust (严格)"(reference=w850) -> ("Controls[]"=w852:refnum<vi>[])  [unwired: 1 in, 2 out]
                      n378 = for {
                        tunnel: w852 -> [w853] mode=indexing
                        tunnel: w851 -> [w854] mode=indexing
                        n379 = property class="Ctl"(reference=w853, "Blinking"=w854) -> ()  [unwired: 1 in, 2 out]
                      }
                    }
                    frame 5 {
                      n380 = control-ref of="1 23"() -> (w855:refnum<vi>)
                      n381 = property class="Clust (严格)"(reference=w855) -> ("Controls[]"=w857:refnum<vi>[])  [unwired: 1 in, 2 out]
                      n382 = for {
                        tunnel: w857 -> [w858] mode=indexing
                        tunnel: w856 -> [w859] mode=indexing
                        n383 = property class="Ctl"(reference=w858, "Blinking"=w859) -> ()  [unwired: 1 in, 2 out]
                      }
                    }
                    frame 6 {
                      n384 = control-ref of="1 24"() -> (w860:refnum<vi>)
                      n385 = property class="Clust (严格)"(reference=w860) -> ("Controls[]"=w862:refnum<vi>[])  [unwired: 1 in, 2 out]
                      n386 = for {
                        tunnel: w862 -> [w863] mode=indexing
                        tunnel: w861 -> [w864] mode=indexing
                        n387 = property class="Ctl"(reference=w863, "Blinking"=w864) -> ()  [unwired: 1 in, 2 out]
                      }
                    }
                    frame 7 {
                      n388 = control-ref of="1 25"() -> (w865:refnum<vi>)
                      n389 = property class="Clust (严格)"(reference=w865) -> ("Controls[]"=w867:refnum<vi>[])  [unwired: 1 in, 2 out]
                      n390 = for {
                        tunnel: w867 -> [w868] mode=indexing
                        tunnel: w866 -> [w869] mode=indexing
                        n391 = property class="Ctl"(reference=w868, "Blinking"=w869) -> ()  [unwired: 1 in, 2 out]
                      }
                    }
                    frame 8 {
                      n392 = control-ref of="1 5"() -> (w870:refnum<vi>)
                      n393 = property class="Clust (严格)"(reference=w870) -> ("Controls[]"=w872:refnum<vi>[])  [unwired: 1 in, 2 out]
                      n394 = for {
                        tunnel: w872 -> [w873] mode=indexing
                        tunnel: w871 -> [w874] mode=indexing
                        n395 = property class="Ctl"(reference=w873, "Blinking"=w874) -> ()  [unwired: 1 in, 2 out]
                      }
                    }
                    frame 99, Default {
                    }
                  }
                }
                n396 = for {
                  N: 16 -> [_]
                  i -> [w747]
                  n397 = case shown="6" w747 {
                    tunnel: bool[] [FALSE, FALSE, FALSE, FALSE, FALSE, FALSE, FALSE, FALSE, FALSE, FALSE, FALSE, FALSE, FALSE] -> [w748 w754 w759 w764 w769 w774 w779 w784 w789 w794 w799 w804 w809 w814 w819 w824 _]
                    frame 0 {
                      n398 = control-ref of="1 102"() -> (w750:refnum<vi>)
                      n399 = property class="Clust (严格)"(reference=w750) -> ("Controls[]"=w749:refnum<vi>[])  [unwired: 1 in, 2 out]
                      n400 = for {
                        tunnel: w749 -> [w751] mode=indexing
                        tunnel: w748 -> [w752] mode=indexing
                        n401 = property class="Ctl"(reference=w751, "Blinking"=w752) -> ()  [unwired: 1 in, 2 out]
                      }
                    }
                    frame 1 {
                      n402 = control-ref of="1 3"() -> (w753:refnum<vi>)
                      n403 = property class="Clust (严格)"(reference=w753) -> ("Controls[]"=w755:refnum<vi>[])  [unwired: 1 in, 2 out]
                      n404 = for {
                        tunnel: w755 -> [w756] mode=indexing
                        tunnel: w754 -> [w757] mode=indexing
                        n405 = property class="Ctl"(reference=w756, "Blinking"=w757) -> ()  [unwired: 1 in, 2 out]
                      }
                    }
                    frame 2 {
                      n406 = control-ref of="1 4"() -> (w758:refnum<vi>)
                      n407 = property class="Clust (严格)"(reference=w758) -> ("Controls[]"=w760:refnum<vi>[])  [unwired: 1 in, 2 out]
                      n408 = for {
                        tunnel: w760 -> [w761] mode=indexing
                        tunnel: w759 -> [w762] mode=indexing
                        n409 = property class="Ctl"(reference=w761, "Blinking"=w762) -> ()  [unwired: 1 in, 2 out]
                      }
                    }
                    frame 3 {
                      n410 = control-ref of="1 6"() -> (w763:refnum<vi>)
                      n411 = property class="Clust (严格)"(reference=w763) -> ("Controls[]"=w765:refnum<vi>[])  [unwired: 1 in, 2 out]
                      n412 = for {
                        tunnel: w765 -> [w766] mode=indexing
                        tunnel: w764 -> [w767] mode=indexing
                        n413 = property class="Ctl"(reference=w766, "Blinking"=w767) -> ()  [unwired: 1 in, 2 out]
                      }
                    }
                    frame 4 {
                      n414 = control-ref of="1 7"() -> (w768:refnum<vi>)
                      n415 = property class="Clust (严格)"(reference=w768) -> ("Controls[]"=w770:refnum<vi>[])  [unwired: 1 in, 2 out]
                      n416 = for {
                        tunnel: w770 -> [w771] mode=indexing
                        tunnel: w769 -> [w772] mode=indexing
                        n417 = property class="Ctl"(reference=w771, "Blinking"=w772) -> ()  [unwired: 1 in, 2 out]
                      }
                    }
                    frame 5 {
                      n418 = control-ref of="1 8"() -> (w773:refnum<vi>)
                      n419 = property class="Clust (严格)"(reference=w773) -> ("Controls[]"=w775:refnum<vi>[])  [unwired: 1 in, 2 out]
                      n420 = for {
                        tunnel: w775 -> [w776] mode=indexing
                        tunnel: w774 -> [w777] mode=indexing
                        n421 = property class="Ctl"(reference=w776, "Blinking"=w777) -> ()  [unwired: 1 in, 2 out]
                      }
                    }
                    frame 6 {
                      n422 = control-ref of="1 9"() -> (w778:refnum<vi>)
                      n423 = property class="Clust (严格)"(reference=w778) -> ("Controls[]"=w780:refnum<vi>[])  [unwired: 1 in, 2 out]
                      n424 = for {
                        tunnel: w780 -> [w781] mode=indexing
                        tunnel: w779 -> [w782] mode=indexing
                        n425 = property class="Ctl"(reference=w781, "Blinking"=w782) -> ()  [unwired: 1 in, 2 out]
                      }
                    }
                    frame 7 {
                      n426 = control-ref of="1 10"() -> (w783:refnum<vi>)
                      n427 = property class="Clust (严格)"(reference=w783) -> ("Controls[]"=w785:refnum<vi>[])  [unwired: 1 in, 2 out]
                      n428 = for {
                        tunnel: w785 -> [w786] mode=indexing
                        tunnel: w784 -> [w787] mode=indexing
                        n429 = property class="Ctl"(reference=w786, "Blinking"=w787) -> ()  [unwired: 1 in, 2 out]
                      }
                    }
                    frame 8 {
                      n430 = control-ref of="1 26"() -> (w788:refnum<vi>)
                      n431 = property class="Clust (严格)"(reference=w788) -> ("Controls[]"=w790:refnum<vi>[])  [unwired: 1 in, 2 out]
                      n432 = for {
                        tunnel: w790 -> [w791] mode=indexing
                        tunnel: w789 -> [w792] mode=indexing
                        n433 = property class="Ctl"(reference=w791, "Blinking"=w792) -> ()  [unwired: 1 in, 2 out]
                      }
                    }
                    frame 9 {
                      n434 = control-ref of="1 27"() -> (w793:refnum<vi>)
                      n435 = property class="Clust (严格)"(reference=w793) -> ("Controls[]"=w795:refnum<vi>[])  [unwired: 1 in, 2 out]
                      n436 = for {
                        tunnel: w795 -> [w796] mode=indexing
                        tunnel: w794 -> [w797] mode=indexing
                        n437 = property class="Ctl"(reference=w796, "Blinking"=w797) -> ()  [unwired: 1 in, 2 out]
                      }
                    }
                    frame 10 {
                      n438 = control-ref of="1 28"() -> (w798:refnum<vi>)
                      n439 = property class="Clust (严格)"(reference=w798) -> ("Controls[]"=w800:refnum<vi>[])  [unwired: 1 in, 2 out]
                      n440 = for {
                        tunnel: w800 -> [w801] mode=indexing
                        tunnel: w799 -> [w802] mode=indexing
                        n441 = property class="Ctl"(reference=w801, "Blinking"=w802) -> ()  [unwired: 1 in, 2 out]
                      }
                    }
                    frame 11 {
                      n442 = control-ref of="1 29"() -> (w803:refnum<vi>)
                      n443 = property class="Clust (严格)"(reference=w803) -> ("Controls[]"=w805:refnum<vi>[])  [unwired: 1 in, 2 out]
                      n444 = for {
                        tunnel: w805 -> [w806] mode=indexing
                        tunnel: w804 -> [w807] mode=indexing
                        n445 = property class="Ctl"(reference=w806, "Blinking"=w807) -> ()  [unwired: 1 in, 2 out]
                      }
                    }
                    frame 12 {
                      n446 = control-ref of="1 30"() -> (w808:refnum<vi>)
                      n447 = property class="Clust (严格)"(reference=w808) -> ("Controls[]"=w810:refnum<vi>[])  [unwired: 1 in, 2 out]
                      n448 = for {
                        tunnel: w810 -> [w811] mode=indexing
                        tunnel: w809 -> [w812] mode=indexing
                        n449 = property class="Ctl"(reference=w811, "Blinking"=w812) -> ()  [unwired: 1 in, 2 out]
                      }
                    }
                    frame 13 {
                      n450 = control-ref of="1 31"() -> (w813:refnum<vi>)
                      n451 = property class="Clust (严格)"(reference=w813) -> ("Controls[]"=w815:refnum<vi>[])  [unwired: 1 in, 2 out]
                      n452 = for {
                        tunnel: w815 -> [w816] mode=indexing
                        tunnel: w814 -> [w817] mode=indexing
                        n453 = property class="Ctl"(reference=w816, "Blinking"=w817) -> ()  [unwired: 1 in, 2 out]
                      }
                    }
                    frame 14 {
                      n454 = control-ref of="1 32"() -> (w818:refnum<vi>)
                      n455 = property class="Clust (严格)"(reference=w818) -> ("Controls[]"=w820:refnum<vi>[])  [unwired: 1 in, 2 out]
                      n456 = for {
                        tunnel: w820 -> [w821] mode=indexing
                        tunnel: w819 -> [w822] mode=indexing
                        n457 = property class="Ctl"(reference=w821, "Blinking"=w822) -> ()  [unwired: 1 in, 2 out]
                      }
                    }
                    frame 15 {
                      n458 = control-ref of="1 33"() -> (w823:refnum<vi>)
                      n459 = property class="Clust (严格)"(reference=w823) -> ("Controls[]"=w825:refnum<vi>[])  [unwired: 1 in, 2 out]
                      n460 = for {
                        tunnel: w825 -> [w826] mode=indexing
                        tunnel: w824 -> [w827] mode=indexing
                        n461 = property class="Ctl"(reference=w826, "Blinking"=w827) -> ()  [unwired: 1 in, 2 out]
                      }
                    }
                    frame 99, Default {
                    }
                  }
                }
              }
              frame "单体温度" {
                n462 = for {
                  N: 16 -> [_]
                  i -> [w878]
                  n463 = case shown="4" w878 {
                    tunnel: bool[] [FALSE, FALSE, FALSE, FALSE, FALSE, FALSE, FALSE, FALSE, FALSE, FALSE, FALSE, FALSE, FALSE] -> [w880 w885 w890 w895 w900 w905 w910 w915 w920 w925 w930 w935 w940 w945 w950 w955 _]
                    frame 0 {
                      n464 = control-ref of="1 102"() -> (w879:refnum<vi>)
                      n465 = property class="Clust (严格)"(reference=w879) -> ("Controls[]"=w881:refnum<vi>[])  [unwired: 1 in, 2 out]
                      n466 = for {
                        tunnel: w881 -> [w882] mode=indexing
                        tunnel: w880 -> [w883] mode=indexing
                        n467 = property class="Ctl"(reference=w882, "Blinking"=w883) -> ()  [unwired: 1 in, 2 out]
                      }
                    }
                    frame 1 {
                      n468 = control-ref of="1 3"() -> (w884:refnum<vi>)
                      n469 = property class="Clust (严格)"(reference=w884) -> ("Controls[]"=w886:refnum<vi>[])  [unwired: 1 in, 2 out]
                      n470 = for {
                        tunnel: w886 -> [w887] mode=indexing
                        tunnel: w885 -> [w888] mode=indexing
                        n471 = property class="Ctl"(reference=w887, "Blinking"=w888) -> ()  [unwired: 1 in, 2 out]
                      }
                    }
                    frame 2 {
                      n472 = control-ref of="1 4"() -> (w889:refnum<vi>)
                      n473 = property class="Clust (严格)"(reference=w889) -> ("Controls[]"=w891:refnum<vi>[])  [unwired: 1 in, 2 out]
                      n474 = for {
                        tunnel: w891 -> [w892] mode=indexing
                        tunnel: w890 -> [w893] mode=indexing
                        n475 = property class="Ctl"(reference=w892, "Blinking"=w893) -> ()  [unwired: 1 in, 2 out]
                      }
                    }
                    frame 3 {
                      n476 = control-ref of="1 6"() -> (w894:refnum<vi>)
                      n477 = property class="Clust (严格)"(reference=w894) -> ("Controls[]"=w896:refnum<vi>[])  [unwired: 1 in, 2 out]
                      n478 = for {
                        tunnel: w896 -> [w897] mode=indexing
                        tunnel: w895 -> [w898] mode=indexing
                        n479 = property class="Ctl"(reference=w897, "Blinking"=w898) -> ()  [unwired: 1 in, 2 out]
                      }
                    }
                    frame 4 {
                      n480 = control-ref of="1 7"() -> (w899:refnum<vi>)
                      n481 = property class="Clust (严格)"(reference=w899) -> ("Controls[]"=w901:refnum<vi>[])  [unwired: 1 in, 2 out]
                      n482 = for {
                        tunnel: w901 -> [w902] mode=indexing
                        tunnel: w900 -> [w903] mode=indexing
                        n483 = property class="Ctl"(reference=w902, "Blinking"=w903) -> ()  [unwired: 1 in, 2 out]
                      }
                    }
                    frame 5 {
                      n484 = control-ref of="1 8"() -> (w904:refnum<vi>)
                      n485 = property class="Clust (严格)"(reference=w904) -> ("Controls[]"=w906:refnum<vi>[])  [unwired: 1 in, 2 out]
                      n486 = for {
                        tunnel: w906 -> [w907] mode=indexing
                        tunnel: w905 -> [w908] mode=indexing
                        n487 = property class="Ctl"(reference=w907, "Blinking"=w908) -> ()  [unwired: 1 in, 2 out]
                      }
                    }
                    frame 6 {
                      n488 = control-ref of="1 9"() -> (w909:refnum<vi>)
                      n489 = property class="Clust (严格)"(reference=w909) -> ("Controls[]"=w911:refnum<vi>[])  [unwired: 1 in, 2 out]
                      n490 = for {
                        tunnel: w911 -> [w912] mode=indexing
                        tunnel: w910 -> [w913] mode=indexing
                        n491 = property class="Ctl"(reference=w912, "Blinking"=w913) -> ()  [unwired: 1 in, 2 out]
                      }
                    }
                    frame 7 {
                      n492 = control-ref of="1 10"() -> (w914:refnum<vi>)
                      n493 = property class="Clust (严格)"(reference=w914) -> ("Controls[]"=w916:refnum<vi>[])  [unwired: 1 in, 2 out]
                      n494 = for {
                        tunnel: w916 -> [w917] mode=indexing
                        tunnel: w915 -> [w918] mode=indexing
                        n495 = property class="Ctl"(reference=w917, "Blinking"=w918) -> ()  [unwired: 1 in, 2 out]
                      }
                    }
                    frame 8 {
                      n496 = control-ref of="1 26"() -> (w919:refnum<vi>)
                      n497 = property class="Clust (严格)"(reference=w919) -> ("Controls[]"=w921:refnum<vi>[])  [unwired: 1 in, 2 out]
                      n498 = for {
                        tunnel: w921 -> [w922] mode=indexing
                        tunnel: w920 -> [w923] mode=indexing
                        n499 = property class="Ctl"(reference=w922, "Blinking"=w923) -> ()  [unwired: 1 in, 2 out]
                      }
                    }
                    frame 9 {
                      n500 = control-ref of="1 27"() -> (w924:refnum<vi>)
                      n501 = property class="Clust (严格)"(reference=w924) -> ("Controls[]"=w926:refnum<vi>[])  [unwired: 1 in, 2 out]
                      n502 = for {
                        tunnel: w926 -> [w927] mode=indexing
                        tunnel: w925 -> [w928] mode=indexing
                        n503 = property class="Ctl"(reference=w927, "Blinking"=w928) -> ()  [unwired: 1 in, 2 out]
                      }
                    }
                    frame 10 {
                      n504 = control-ref of="1 28"() -> (w929:refnum<vi>)
                      n505 = property class="Clust (严格)"(reference=w929) -> ("Controls[]"=w931:refnum<vi>[])  [unwired: 1 in, 2 out]
                      n506 = for {
                        tunnel: w931 -> [w932] mode=indexing
                        tunnel: w930 -> [w933] mode=indexing
                        n507 = property class="Ctl"(reference=w932, "Blinking"=w933) -> ()  [unwired: 1 in, 2 out]
                      }
                    }
                    frame 11 {
                      n508 = control-ref of="1 29"() -> (w934:refnum<vi>)
                      n509 = property class="Clust (严格)"(reference=w934) -> ("Controls[]"=w936:refnum<vi>[])  [unwired: 1 in, 2 out]
                      n510 = for {
                        tunnel: w936 -> [w937] mode=indexing
                        tunnel: w935 -> [w938] mode=indexing
                        n511 = property class="Ctl"(reference=w937, "Blinking"=w938) -> ()  [unwired: 1 in, 2 out]
                      }
                    }
                    frame 12 {
                      n512 = control-ref of="1 30"() -> (w939:refnum<vi>)
                      n513 = property class="Clust (严格)"(reference=w939) -> ("Controls[]"=w941:refnum<vi>[])  [unwired: 1 in, 2 out]
                      n514 = for {
                        tunnel: w941 -> [w942] mode=indexing
                        tunnel: w940 -> [w943] mode=indexing
                        n515 = property class="Ctl"(reference=w942, "Blinking"=w943) -> ()  [unwired: 1 in, 2 out]
                      }
                    }
                    frame 13 {
                      n516 = control-ref of="1 31"() -> (w944:refnum<vi>)
                      n517 = property class="Clust (严格)"(reference=w944) -> ("Controls[]"=w946:refnum<vi>[])  [unwired: 1 in, 2 out]
                      n518 = for {
                        tunnel: w946 -> [w947] mode=indexing
                        tunnel: w945 -> [w948] mode=indexing
                        n519 = property class="Ctl"(reference=w947, "Blinking"=w948) -> ()  [unwired: 1 in, 2 out]
                      }
                    }
                    frame 14 {
                      n520 = control-ref of="1 32"() -> (w949:refnum<vi>)
                      n521 = property class="Clust (严格)"(reference=w949) -> ("Controls[]"=w951:refnum<vi>[])  [unwired: 1 in, 2 out]
                      n522 = for {
                        tunnel: w951 -> [w952] mode=indexing
                        tunnel: w950 -> [w953] mode=indexing
                        n523 = property class="Ctl"(reference=w952, "Blinking"=w953) -> ()  [unwired: 1 in, 2 out]
                      }
                    }
                    frame 15 {
                      n524 = control-ref of="1 33"() -> (w954:refnum<vi>)
                      n525 = property class="Clust (严格)"(reference=w954) -> ("Controls[]"=w956:refnum<vi>[])  [unwired: 1 in, 2 out]
                      n526 = for {
                        tunnel: w956 -> [w957] mode=indexing
                        tunnel: w955 -> [w958] mode=indexing
                        n527 = property class="Ctl"(reference=w957, "Blinking"=w958) -> ()  [unwired: 1 in, 2 out]
                      }
                    }
                    frame 99, Default {
                    }
                  }
                }
                n528 = for {
                  N: 9 -> [_]
                  i -> [w960]
                  n529 = case shown="8" w960 {
                    tunnel: bool[] [FALSE, FALSE, FALSE, FALSE, FALSE, FALSE, FALSE, FALSE, FALSE, FALSE, FALSE, FALSE, FALSE] -> [w962 w967 w972 w977 w982 w987 w992 w997 w1002 _]
                    frame 0 {
                      n530 = control-ref of="1 18"() -> (w961:refnum<vi>)
                      n531 = property class="Clust (严格)"(reference=w961) -> ("Controls[]"=w963:refnum<vi>[])  [unwired: 1 in, 2 out]
                      n532 = for {
                        tunnel: w963 -> [w964] mode=indexing
                        tunnel: w962 -> [w965] mode=indexing
                        n533 = property class="Ctl"(reference=w964, "Blinking"=w965) -> ()  [unwired: 1 in, 2 out]
                      }
                    }
                    frame 1 {
                      n534 = control-ref of="1 19"() -> (w966:refnum<vi>)
                      n535 = property class="Clust (严格)"(reference=w966) -> ("Controls[]"=w968:refnum<vi>[])  [unwired: 1 in, 2 out]
                      n536 = for {
                        tunnel: w968 -> [w969] mode=indexing
                        tunnel: w967 -> [w970] mode=indexing
                        n537 = property class="Ctl"(reference=w969, "Blinking"=w970) -> ()  [unwired: 1 in, 2 out]
                      }
                    }
                    frame 2 {
                      n538 = control-ref of="1 20"() -> (w971:refnum<vi>)
                      n539 = property class="Clust (严格)"(reference=w971) -> ("Controls[]"=w973:refnum<vi>[])  [unwired: 1 in, 2 out]
                      n540 = for {
                        tunnel: w973 -> [w974] mode=indexing
                        tunnel: w972 -> [w975] mode=indexing
                        n541 = property class="Ctl"(reference=w974, "Blinking"=w975) -> ()  [unwired: 1 in, 2 out]
                      }
                    }
                    frame 3 {
                      n542 = control-ref of="1 21"() -> (w976:refnum<vi>)
                      n543 = property class="Clust (严格)"(reference=w976) -> ("Controls[]"=w978:refnum<vi>[])  [unwired: 1 in, 2 out]
                      n544 = for {
                        tunnel: w978 -> [w979] mode=indexing
                        tunnel: w977 -> [w980] mode=indexing
                        n545 = property class="Ctl"(reference=w979, "Blinking"=w980) -> ()  [unwired: 1 in, 2 out]
                      }
                    }
                    frame 4 {
                      n546 = control-ref of="1 22"() -> (w981:refnum<vi>)
                      n547 = property class="Clust (严格)"(reference=w981) -> ("Controls[]"=w983:refnum<vi>[])  [unwired: 1 in, 2 out]
                      n548 = for {
                        tunnel: w983 -> [w984] mode=indexing
                        tunnel: w982 -> [w985] mode=indexing
                        n549 = property class="Ctl"(reference=w984, "Blinking"=w985) -> ()  [unwired: 1 in, 2 out]
                      }
                    }
                    frame 5 {
                      n550 = control-ref of="1 23"() -> (w986:refnum<vi>)
                      n551 = property class="Clust (严格)"(reference=w986) -> ("Controls[]"=w988:refnum<vi>[])  [unwired: 1 in, 2 out]
                      n552 = for {
                        tunnel: w988 -> [w989] mode=indexing
                        tunnel: w987 -> [w990] mode=indexing
                        n553 = property class="Ctl"(reference=w989, "Blinking"=w990) -> ()  [unwired: 1 in, 2 out]
                      }
                    }
                    frame 6 {
                      n554 = control-ref of="1 24"() -> (w991:refnum<vi>)
                      n555 = property class="Clust (严格)"(reference=w991) -> ("Controls[]"=w993:refnum<vi>[])  [unwired: 1 in, 2 out]
                      n556 = for {
                        tunnel: w993 -> [w994] mode=indexing
                        tunnel: w992 -> [w995] mode=indexing
                        n557 = property class="Ctl"(reference=w994, "Blinking"=w995) -> ()  [unwired: 1 in, 2 out]
                      }
                    }
                    frame 7 {
                      n558 = control-ref of="1 25"() -> (w996:refnum<vi>)
                      n559 = property class="Clust (严格)"(reference=w996) -> ("Controls[]"=w998:refnum<vi>[])  [unwired: 1 in, 2 out]
                      n560 = for {
                        tunnel: w998 -> [w999] mode=indexing
                        tunnel: w997 -> [w1000] mode=indexing
                        n561 = property class="Ctl"(reference=w999, "Blinking"=w1000) -> ()  [unwired: 1 in, 2 out]
                      }
                    }
                    frame 8 {
                      n562 = control-ref of="1 6"() -> (w1001:refnum<vi>)
                      n563 = property class="Clust (严格)"(reference=w1001) -> ("Controls[]"=w1003:refnum<vi>[])  [unwired: 1 in, 2 out]
                      n564 = for {
                        tunnel: w1003 -> [w1004] mode=indexing
                        tunnel: w1002 -> [w1005] mode=indexing
                        n565 = property class="Ctl"(reference=w1004, "Blinking"=w1005) -> ()  [unwired: 1 in, 2 out]
                      }
                    }
                    frame 99, Default {
                    }
                  }
                }
              }
            }
            n566 = local write "一次置位"(FALSE ("一次置位")) -> ()
          }
        }
      }
      frame True {
        n567 = case shown="\"单体温度\"" w1007 {
          frame "单体电压", Default {
            w1011 = 17 ("y")
            n568 = global read "单体信息全局.vi" "数据"() -> (w1024:dbl[])
            n569 = global read "单体信息全局.vi" "PF"() -> (w1010:i32)
            n570 = Array Subset(array=w1024, length=w1010) -> (w1023:dbl[])  [unwired: 1 in]
            n571 = Subtract(x="基准", y="偏差") -> (x-y=w1020:dbl)
            n572 = Quotient & Remainder(x=w1010, y=12) -> (x-y*floor(x/y)=w1016:i32, floor(x/y)=w1014:i32)
            n573 = Add(x="基准", y="偏差") -> (x+y=w1019:dbl)
            n574 = Equal To 0?(x=w1016) -> (x = 0?=w1015:bool)
            n575 = In Range and Coerce(upper limit=w1019, x=w1023, lower limit=w1020) -> (In Range?=w1018:bool[])  [unwired: 1 out]
            n576 = Increment(x=w1014) -> (x+1=w1013:i32)
            n577 = Select(t=w1014, s=w1015, f=w1013) -> (s? t:f=w1009:i32)
            n578 = Not(x=w1018) -> (.not. x?=w1008:bool[])
            n579 = Greater Or Equal?(x=w1009, y=w1011) -> (x >= y?=w1012:bool)
            n580 = case shown="真" w1012 {
              tunnel: w1009 -> [w1114 _]
              tunnel: w1011 -> [w1111 _]
              tunnel: w1008 -> [w1112 _]
              frame True {
                n581 = Decrement(x=w1111) -> (x-1=w1110:i32)
                n582 = Subtract(x=w1114, y=w1110) -> (x-y=w1113:i32)
                n583 = for {
                  N: w1113 -> [_]
                  tunnel: w1112 -> [w1120]
                  tunnel: w1110 -> [w1115]
                  i -> [w1121]
                  w1118 = 12 ("y")
                  n584 = Add(x=w1115, y=w1121) -> (x+y=w1116:i32)
                  n585 = Multiply(x=w1116, y=w1118) -> (x*y=w1119:i32)
                  n586 = Array Subset(array=w1120, index=w1119, length=w1118) -> (w1117:bool[])
                  n587 = case shown="0" w1121 {
                    tunnel: w1117 -> [w1123 w1128 w1133 w1138 w1143 w1148 w1153 w1158 w1163 _]
                    frame 0 {
                      n588 = control-ref of="1 18"() -> (w1122:refnum<vi>)
                      n589 = property class="Clust (严格)"(reference=w1122) -> ("Controls[]"=w1124:refnum<vi>[])  [unwired: 1 in, 2 out]
                      n590 = for {
                        tunnel: w1124 -> [w1125] mode=indexing
                        tunnel: w1123 -> [w1126] mode=indexing
                        n591 = property class="Ctl"(reference=w1125, "Blinking"=w1126) -> ()  [unwired: 1 in, 2 out]
                      }
                    }
                    frame 1 {
                      n592 = control-ref of="1 19"() -> (w1127:refnum<vi>)
                      n593 = property class="Clust (严格)"(reference=w1127) -> ("Controls[]"=w1129:refnum<vi>[])  [unwired: 1 in, 2 out]
                      n594 = for {
                        tunnel: w1129 -> [w1130] mode=indexing
                        tunnel: w1128 -> [w1131] mode=indexing
                        n595 = property class="Ctl"(reference=w1130, "Blinking"=w1131) -> ()  [unwired: 1 in, 2 out]
                      }
                    }
                    frame 2 {
                      n596 = control-ref of="1 20"() -> (w1132:refnum<vi>)
                      n597 = property class="Clust (严格)"(reference=w1132) -> ("Controls[]"=w1134:refnum<vi>[])  [unwired: 1 in, 2 out]
                      n598 = for {
                        tunnel: w1134 -> [w1135] mode=indexing
                        tunnel: w1133 -> [w1136] mode=indexing
                        n599 = property class="Ctl"(reference=w1135, "Blinking"=w1136) -> ()  [unwired: 1 in, 2 out]
                      }
                    }
                    frame 3 {
                      n600 = control-ref of="1 21"() -> (w1137:refnum<vi>)
                      n601 = property class="Clust (严格)"(reference=w1137) -> ("Controls[]"=w1139:refnum<vi>[])  [unwired: 1 in, 2 out]
                      n602 = for {
                        tunnel: w1139 -> [w1140] mode=indexing
                        tunnel: w1138 -> [w1141] mode=indexing
                        n603 = property class="Ctl"(reference=w1140, "Blinking"=w1141) -> ()  [unwired: 1 in, 2 out]
                      }
                    }
                    frame 4 {
                      n604 = control-ref of="1 22"() -> (w1142:refnum<vi>)
                      n605 = property class="Clust (严格)"(reference=w1142) -> ("Controls[]"=w1144:refnum<vi>[])  [unwired: 1 in, 2 out]
                      n606 = for {
                        tunnel: w1144 -> [w1145] mode=indexing
                        tunnel: w1143 -> [w1146] mode=indexing
                        n607 = property class="Ctl"(reference=w1145, "Blinking"=w1146) -> ()  [unwired: 1 in, 2 out]
                      }
                    }
                    frame 5 {
                      n608 = control-ref of="1 23"() -> (w1147:refnum<vi>)
                      n609 = property class="Clust (严格)"(reference=w1147) -> ("Controls[]"=w1149:refnum<vi>[])  [unwired: 1 in, 2 out]
                      n610 = for {
                        tunnel: w1149 -> [w1150] mode=indexing
                        tunnel: w1148 -> [w1151] mode=indexing
                        n611 = property class="Ctl"(reference=w1150, "Blinking"=w1151) -> ()  [unwired: 1 in, 2 out]
                      }
                    }
                    frame 6 {
                      n612 = control-ref of="1 24"() -> (w1152:refnum<vi>)
                      n613 = property class="Clust (严格)"(reference=w1152) -> ("Controls[]"=w1154:refnum<vi>[])  [unwired: 1 in, 2 out]
                      n614 = for {
                        tunnel: w1154 -> [w1155] mode=indexing
                        tunnel: w1153 -> [w1156] mode=indexing
                        n615 = property class="Ctl"(reference=w1155, "Blinking"=w1156) -> ()  [unwired: 1 in, 2 out]
                      }
                    }
                    frame 7 {
                      n616 = control-ref of="1 25"() -> (w1157:refnum<vi>)
                      n617 = property class="Clust (严格)"(reference=w1157) -> ("Controls[]"=w1159:refnum<vi>[])  [unwired: 1 in, 2 out]
                      n618 = for {
                        tunnel: w1159 -> [w1160] mode=indexing
                        tunnel: w1158 -> [w1161] mode=indexing
                        n619 = property class="Ctl"(reference=w1160, "Blinking"=w1161) -> ()  [unwired: 1 in, 2 out]
                      }
                    }
                    frame 8 {
                      n620 = control-ref of="1 5"() -> (w1162:refnum<vi>)
                      n621 = property class="Clust (严格)"(reference=w1162) -> ("Controls[]"=w1164:refnum<vi>[])  [unwired: 1 in, 2 out]
                      n622 = for {
                        tunnel: w1164 -> [w1165] mode=indexing
                        tunnel: w1163 -> [w1166] mode=indexing
                        n623 = property class="Ctl"(reference=w1165, "Blinking"=w1166) -> ()  [unwired: 1 in, 2 out]
                      }
                    }
                    frame 99, Default {
                    }
                  }
                }
              }
              frame False {
              }
            }
            n624 = for {
              N: w1009 -> [_]
              tunnel: w1008 -> [w1028]
              i -> [w1029]
              w1026 = 12 ("y")
              n625 = Multiply(x=w1029, y=w1026) -> (x*y=w1027:i32)
              n626 = Array Subset(array=w1028, index=w1027, length=w1026) -> (w1025:bool[])
              n627 = case shown="7" w1029 {
                tunnel: w1025 -> [w1030 w1036 w1041 w1046 w1051 w1056 w1061 w1066 w1071 w1076 w1081 w1086 w1091 w1096 w1101 w1106 _]
                frame 0 {
                  n628 = control-ref of="1 102"() -> (w1032:refnum<vi>)
                  n629 = property class="Clust (严格)"(reference=w1032) -> ("Controls[]"=w1031:refnum<vi>[])  [unwired: 1 in, 2 out]
                  n630 = for {
                    tunnel: w1031 -> [w1033] mode=indexing
                    tunnel: w1030 -> [w1034] mode=indexing
                    n631 = property class="Ctl"(reference=w1033, "Blinking"=w1034) -> ()  [unwired: 1 in, 2 out]
                  }
                }
                frame 1 {
                  n632 = control-ref of="1 3"() -> (w1035:refnum<vi>)
                  n633 = property class="Clust (严格)"(reference=w1035) -> ("Controls[]"=w1037:refnum<vi>[])  [unwired: 1 in, 2 out]
                  n634 = for {
                    tunnel: w1037 -> [w1038] mode=indexing
                    tunnel: w1036 -> [w1039] mode=indexing
                    n635 = property class="Ctl"(reference=w1038, "Blinking"=w1039) -> ()  [unwired: 1 in, 2 out]
                  }
                }
                frame 2 {
                  n636 = control-ref of="1 4"() -> (w1040:refnum<vi>)
                  n637 = property class="Clust (严格)"(reference=w1040) -> ("Controls[]"=w1042:refnum<vi>[])  [unwired: 1 in, 2 out]
                  n638 = for {
                    tunnel: w1042 -> [w1043] mode=indexing
                    tunnel: w1041 -> [w1044] mode=indexing
                    n639 = property class="Ctl"(reference=w1043, "Blinking"=w1044) -> ()  [unwired: 1 in, 2 out]
                  }
                }
                frame 3 {
                  n640 = control-ref of="1 6"() -> (w1045:refnum<vi>)
                  n641 = property class="Clust (严格)"(reference=w1045) -> ("Controls[]"=w1047:refnum<vi>[])  [unwired: 1 in, 2 out]
                  n642 = for {
                    tunnel: w1047 -> [w1048] mode=indexing
                    tunnel: w1046 -> [w1049] mode=indexing
                    n643 = property class="Ctl"(reference=w1048, "Blinking"=w1049) -> ()  [unwired: 1 in, 2 out]
                  }
                }
                frame 4 {
                  n644 = control-ref of="1 7"() -> (w1050:refnum<vi>)
                  n645 = property class="Clust (严格)"(reference=w1050) -> ("Controls[]"=w1052:refnum<vi>[])  [unwired: 1 in, 2 out]
                  n646 = for {
                    tunnel: w1052 -> [w1053] mode=indexing
                    tunnel: w1051 -> [w1054] mode=indexing
                    n647 = property class="Ctl"(reference=w1053, "Blinking"=w1054) -> ()  [unwired: 1 in, 2 out]
                  }
                }
                frame 5 {
                  n648 = control-ref of="1 8"() -> (w1055:refnum<vi>)
                  n649 = property class="Clust (严格)"(reference=w1055) -> ("Controls[]"=w1057:refnum<vi>[])  [unwired: 1 in, 2 out]
                  n650 = for {
                    tunnel: w1057 -> [w1058] mode=indexing
                    tunnel: w1056 -> [w1059] mode=indexing
                    n651 = property class="Ctl"(reference=w1058, "Blinking"=w1059) -> ()  [unwired: 1 in, 2 out]
                  }
                }
                frame 6 {
                  n652 = control-ref of="1 9"() -> (w1060:refnum<vi>)
                  n653 = property class="Clust (严格)"(reference=w1060) -> ("Controls[]"=w1062:refnum<vi>[])  [unwired: 1 in, 2 out]
                  n654 = for {
                    tunnel: w1062 -> [w1063] mode=indexing
                    tunnel: w1061 -> [w1064] mode=indexing
                    n655 = property class="Ctl"(reference=w1063, "Blinking"=w1064) -> ()  [unwired: 1 in, 2 out]
                  }
                }
                frame 7 {
                  n656 = control-ref of="1 10"() -> (w1065:refnum<vi>)
                  n657 = property class="Clust (严格)"(reference=w1065) -> ("Controls[]"=w1067:refnum<vi>[])  [unwired: 1 in, 2 out]
                  n658 = for {
                    tunnel: w1067 -> [w1068] mode=indexing
                    tunnel: w1066 -> [w1069] mode=indexing
                    n659 = property class="Ctl"(reference=w1068, "Blinking"=w1069) -> ()  [unwired: 1 in, 2 out]
                  }
                }
                frame 8 {
                  n660 = control-ref of="1 26"() -> (w1070:refnum<vi>)
                  n661 = property class="Clust (严格)"(reference=w1070) -> ("Controls[]"=w1072:refnum<vi>[])  [unwired: 1 in, 2 out]
                  n662 = for {
                    tunnel: w1072 -> [w1073] mode=indexing
                    tunnel: w1071 -> [w1074] mode=indexing
                    n663 = property class="Ctl"(reference=w1073, "Blinking"=w1074) -> ()  [unwired: 1 in, 2 out]
                  }
                }
                frame 9 {
                  n664 = control-ref of="1 27"() -> (w1075:refnum<vi>)
                  n665 = property class="Clust (严格)"(reference=w1075) -> ("Controls[]"=w1077:refnum<vi>[])  [unwired: 1 in, 2 out]
                  n666 = for {
                    tunnel: w1077 -> [w1078] mode=indexing
                    tunnel: w1076 -> [w1079] mode=indexing
                    n667 = property class="Ctl"(reference=w1078, "Blinking"=w1079) -> ()  [unwired: 1 in, 2 out]
                  }
                }
                frame 10 {
                  n668 = control-ref of="1 28"() -> (w1080:refnum<vi>)
                  n669 = property class="Clust (严格)"(reference=w1080) -> ("Controls[]"=w1082:refnum<vi>[])  [unwired: 1 in, 2 out]
                  n670 = for {
                    tunnel: w1082 -> [w1083] mode=indexing
                    tunnel: w1081 -> [w1084] mode=indexing
                    n671 = property class="Ctl"(reference=w1083, "Blinking"=w1084) -> ()  [unwired: 1 in, 2 out]
                  }
                }
                frame 11 {
                  n672 = control-ref of="1 29"() -> (w1085:refnum<vi>)
                  n673 = property class="Clust (严格)"(reference=w1085) -> ("Controls[]"=w1087:refnum<vi>[])  [unwired: 1 in, 2 out]
                  n674 = for {
                    tunnel: w1087 -> [w1088] mode=indexing
                    tunnel: w1086 -> [w1089] mode=indexing
                    n675 = property class="Ctl"(reference=w1088, "Blinking"=w1089) -> ()  [unwired: 1 in, 2 out]
                  }
                }
                frame 12 {
                  n676 = control-ref of="1 30"() -> (w1090:refnum<vi>)
                  n677 = property class="Clust (严格)"(reference=w1090) -> ("Controls[]"=w1092:refnum<vi>[])  [unwired: 1 in, 2 out]
                  n678 = for {
                    tunnel: w1092 -> [w1093] mode=indexing
                    tunnel: w1091 -> [w1094] mode=indexing
                    n679 = property class="Ctl"(reference=w1093, "Blinking"=w1094) -> ()  [unwired: 1 in, 2 out]
                  }
                }
                frame 13 {
                  n680 = control-ref of="1 31"() -> (w1095:refnum<vi>)
                  n681 = property class="Clust (严格)"(reference=w1095) -> ("Controls[]"=w1097:refnum<vi>[])  [unwired: 1 in, 2 out]
                  n682 = for {
                    tunnel: w1097 -> [w1098] mode=indexing
                    tunnel: w1096 -> [w1099] mode=indexing
                    n683 = property class="Ctl"(reference=w1098, "Blinking"=w1099) -> ()  [unwired: 1 in, 2 out]
                  }
                }
                frame 14 {
                  n684 = control-ref of="1 32"() -> (w1100:refnum<vi>)
                  n685 = property class="Clust (严格)"(reference=w1100) -> ("Controls[]"=w1102:refnum<vi>[])  [unwired: 1 in, 2 out]
                  n686 = for {
                    tunnel: w1102 -> [w1103] mode=indexing
                    tunnel: w1101 -> [w1104] mode=indexing
                    n687 = property class="Ctl"(reference=w1103, "Blinking"=w1104) -> ()  [unwired: 1 in, 2 out]
                  }
                }
                frame 15 {
                  n688 = control-ref of="1 33"() -> (w1105:refnum<vi>)
                  n689 = property class="Clust (严格)"(reference=w1105) -> ("Controls[]"=w1107:refnum<vi>[])  [unwired: 1 in, 2 out]
                  n690 = for {
                    tunnel: w1107 -> [w1108] mode=indexing
                    tunnel: w1106 -> [w1109] mode=indexing
                    n691 = property class="Ctl"(reference=w1108, "Blinking"=w1109) -> ()  [unwired: 1 in, 2 out]
                  }
                }
                frame 99, Default {
                }
              }
            }
          }
          frame "单体温度" {
            w1170 = 17 ("y")
            n692 = global read "单体信息全局.vi" "PF2"() -> (w1169:i32)
            n693 = global read "单体信息全局.vi" "数据 2"() -> (w1183:dbl[])
            n694 = Array Subset(array=w1183, length=w1169) -> (w1182:dbl[])  [unwired: 1 in]
            n695 = Subtract(x="基准", y="偏差") -> (x-y=w1179:dbl)
            n696 = Quotient & Remainder(x=w1169, y=12) -> (x-y*floor(x/y)=w1175:i32, floor(x/y)=w1173:i32)
            n697 = Add(x="基准", y="偏差") -> (x+y=w1178:dbl)
            n698 = Equal To 0?(x=w1175) -> (x = 0?=w1174:bool)
            n699 = In Range and Coerce(upper limit=w1178, x=w1182, lower limit=w1179) -> (In Range?=w1177:bool[])  [unwired: 1 out]
            n700 = Increment(x=w1173) -> (x+1=w1172:i32)
            n701 = Select(t=w1173, s=w1174, f=w1172) -> (s? t:f=w1168:i32)
            n702 = Not(x=w1177) -> (.not. x?=w1167:bool[])
            n703 = Greater Or Equal?(x=w1168, y=w1170) -> (x >= y?=w1171:bool)
            n704 = case shown="真" w1171 {
              tunnel: w1168 -> [w1273 _]
              tunnel: w1170 -> [w1270 _]
              tunnel: w1167 -> [w1271 _]
              frame True {
                n705 = Decrement(x=w1270) -> (x-1=w1269:i32)
                n706 = Subtract(x=w1273, y=w1269) -> (x-y=w1272:i32)
                n707 = for {
                  N: w1272 -> [_]
                  tunnel: w1271 -> [w1279]
                  tunnel: w1269 -> [w1274]
                  i -> [w1280]
                  w1277 = 12 ("y")
                  n708 = Add(x=w1274, y=w1280) -> (x+y=w1275:i32)
                  n709 = Multiply(x=w1275, y=w1277) -> (x*y=w1278:i32)
                  n710 = Array Subset(array=w1279, index=w1278, length=w1277) -> (w1276:bool[])
                  n711 = case shown="0" w1280 {
                    tunnel: w1276 -> [w1282 w1287 w1292 w1297 w1302 w1307 w1312 w1317 w1322 _]
                    frame 0 {
                      n712 = control-ref of="1 18"() -> (w1281:refnum<vi>)
                      n713 = property class="Clust (严格)"(reference=w1281) -> ("Controls[]"=w1283:refnum<vi>[])  [unwired: 1 in, 2 out]
                      n714 = for {
                        tunnel: w1283 -> [w1284] mode=indexing
                        tunnel: w1282 -> [w1285] mode=indexing
                        n715 = property class="Ctl"(reference=w1284, "Blinking"=w1285) -> ()  [unwired: 1 in, 2 out]
                      }
                    }
                    frame 1 {
                      n716 = control-ref of="1 19"() -> (w1286:refnum<vi>)
                      n717 = property class="Clust (严格)"(reference=w1286) -> ("Controls[]"=w1288:refnum<vi>[])  [unwired: 1 in, 2 out]
                      n718 = for {
                        tunnel: w1288 -> [w1289] mode=indexing
                        tunnel: w1287 -> [w1290] mode=indexing
                        n719 = property class="Ctl"(reference=w1289, "Blinking"=w1290) -> ()  [unwired: 1 in, 2 out]
                      }
                    }
                    frame 2 {
                      n720 = control-ref of="1 20"() -> (w1291:refnum<vi>)
                      n721 = property class="Clust (严格)"(reference=w1291) -> ("Controls[]"=w1293:refnum<vi>[])  [unwired: 1 in, 2 out]
                      n722 = for {
                        tunnel: w1293 -> [w1294] mode=indexing
                        tunnel: w1292 -> [w1295] mode=indexing
                        n723 = property class="Ctl"(reference=w1294, "Blinking"=w1295) -> ()  [unwired: 1 in, 2 out]
                      }
                    }
                    frame 3 {
                      n724 = control-ref of="1 21"() -> (w1296:refnum<vi>)
                      n725 = property class="Clust (严格)"(reference=w1296) -> ("Controls[]"=w1298:refnum<vi>[])  [unwired: 1 in, 2 out]
                      n726 = for {
                        tunnel: w1298 -> [w1299] mode=indexing
                        tunnel: w1297 -> [w1300] mode=indexing
                        n727 = property class="Ctl"(reference=w1299, "Blinking"=w1300) -> ()  [unwired: 1 in, 2 out]
                      }
                    }
                    frame 4 {
                      n728 = control-ref of="1 22"() -> (w1301:refnum<vi>)
                      n729 = property class="Clust (严格)"(reference=w1301) -> ("Controls[]"=w1303:refnum<vi>[])  [unwired: 1 in, 2 out]
                      n730 = for {
                        tunnel: w1303 -> [w1304] mode=indexing
                        tunnel: w1302 -> [w1305] mode=indexing
                        n731 = property class="Ctl"(reference=w1304, "Blinking"=w1305) -> ()  [unwired: 1 in, 2 out]
                      }
                    }
                    frame 5 {
                      n732 = control-ref of="1 23"() -> (w1306:refnum<vi>)
                      n733 = property class="Clust (严格)"(reference=w1306) -> ("Controls[]"=w1308:refnum<vi>[])  [unwired: 1 in, 2 out]
                      n734 = for {
                        tunnel: w1308 -> [w1309] mode=indexing
                        tunnel: w1307 -> [w1310] mode=indexing
                        n735 = property class="Ctl"(reference=w1309, "Blinking"=w1310) -> ()  [unwired: 1 in, 2 out]
                      }
                    }
                    frame 6 {
                      n736 = control-ref of="1 24"() -> (w1311:refnum<vi>)
                      n737 = property class="Clust (严格)"(reference=w1311) -> ("Controls[]"=w1313:refnum<vi>[])  [unwired: 1 in, 2 out]
                      n738 = for {
                        tunnel: w1313 -> [w1314] mode=indexing
                        tunnel: w1312 -> [w1315] mode=indexing
                        n739 = property class="Ctl"(reference=w1314, "Blinking"=w1315) -> ()  [unwired: 1 in, 2 out]
                      }
                    }
                    frame 7 {
                      n740 = control-ref of="1 25"() -> (w1316:refnum<vi>)
                      n741 = property class="Clust (严格)"(reference=w1316) -> ("Controls[]"=w1318:refnum<vi>[])  [unwired: 1 in, 2 out]
                      n742 = for {
                        tunnel: w1318 -> [w1319] mode=indexing
                        tunnel: w1317 -> [w1320] mode=indexing
                        n743 = property class="Ctl"(reference=w1319, "Blinking"=w1320) -> ()  [unwired: 1 in, 2 out]
                      }
                    }
                    frame 8 {
                      n744 = control-ref of="1 6"() -> (w1321:refnum<vi>)
                      n745 = property class="Clust (严格)"(reference=w1321) -> ("Controls[]"=w1323:refnum<vi>[])  [unwired: 1 in, 2 out]
                      n746 = for {
                        tunnel: w1323 -> [w1324] mode=indexing
                        tunnel: w1322 -> [w1325] mode=indexing
                        n747 = property class="Ctl"(reference=w1324, "Blinking"=w1325) -> ()  [unwired: 1 in, 2 out]
                      }
                    }
                    frame 99, Default {
                    }
                  }
                }
              }
              frame False {
              }
            }
            n748 = for {
              N: w1168 -> [_]
              tunnel: w1167 -> [w1187]
              i -> [w1188]
              w1185 = 12 ("y")
              n749 = Multiply(x=w1188, y=w1185) -> (x*y=w1186:i32)
              n750 = Array Subset(array=w1187, index=w1186, length=w1185) -> (w1184:bool[])
              n751 = case shown="15" w1188 {
                tunnel: w1184 -> [w1190 w1195 w1200 w1205 w1210 w1215 w1220 w1225 w1230 w1235 w1240 w1245 w1250 w1255 w1260 w1265 _]
                frame 0 {
                  n752 = control-ref of="1 102"() -> (w1189:refnum<vi>)
                  n753 = property class="Clust (严格)"(reference=w1189) -> ("Controls[]"=w1191:refnum<vi>[])  [unwired: 1 in, 2 out]
                  n754 = for {
                    tunnel: w1191 -> [w1192] mode=indexing
                    tunnel: w1190 -> [w1193] mode=indexing
                    n755 = property class="Ctl"(reference=w1192, "Blinking"=w1193) -> ()  [unwired: 1 in, 2 out]
                  }
                }
                frame 1 {
                  n756 = control-ref of="1 3"() -> (w1194:refnum<vi>)
                  n757 = property class="Clust (严格)"(reference=w1194) -> ("Controls[]"=w1196:refnum<vi>[])  [unwired: 1 in, 2 out]
                  n758 = for {
                    tunnel: w1196 -> [w1197] mode=indexing
                    tunnel: w1195 -> [w1198] mode=indexing
                    n759 = property class="Ctl"(reference=w1197, "Blinking"=w1198) -> ()  [unwired: 1 in, 2 out]
                  }
                }
                frame 2 {
                  n760 = control-ref of="1 4"() -> (w1199:refnum<vi>)
                  n761 = property class="Clust (严格)"(reference=w1199) -> ("Controls[]"=w1201:refnum<vi>[])  [unwired: 1 in, 2 out]
                  n762 = for {
                    tunnel: w1201 -> [w1202] mode=indexing
                    tunnel: w1200 -> [w1203] mode=indexing
                    n763 = property class="Ctl"(reference=w1202, "Blinking"=w1203) -> ()  [unwired: 1 in, 2 out]
                  }
                }
                frame 3 {
                  n764 = control-ref of="1 6"() -> (w1204:refnum<vi>)
                  n765 = property class="Clust (严格)"(reference=w1204) -> ("Controls[]"=w1206:refnum<vi>[])  [unwired: 1 in, 2 out]
                  n766 = for {
                    tunnel: w1206 -> [w1207] mode=indexing
                    tunnel: w1205 -> [w1208] mode=indexing
                    n767 = property class="Ctl"(reference=w1207, "Blinking"=w1208) -> ()  [unwired: 1 in, 2 out]
                  }
                }
                frame 4 {
                  n768 = control-ref of="1 7"() -> (w1209:refnum<vi>)
                  n769 = property class="Clust (严格)"(reference=w1209) -> ("Controls[]"=w1211:refnum<vi>[])  [unwired: 1 in, 2 out]
                  n770 = for {
                    tunnel: w1211 -> [w1212] mode=indexing
                    tunnel: w1210 -> [w1213] mode=indexing
                    n771 = property class="Ctl"(reference=w1212, "Blinking"=w1213) -> ()  [unwired: 1 in, 2 out]
                  }
                }
                frame 5 {
                  n772 = control-ref of="1 8"() -> (w1214:refnum<vi>)
                  n773 = property class="Clust (严格)"(reference=w1214) -> ("Controls[]"=w1216:refnum<vi>[])  [unwired: 1 in, 2 out]
                  n774 = for {
                    tunnel: w1216 -> [w1217] mode=indexing
                    tunnel: w1215 -> [w1218] mode=indexing
                    n775 = property class="Ctl"(reference=w1217, "Blinking"=w1218) -> ()  [unwired: 1 in, 2 out]
                  }
                }
                frame 6 {
                  n776 = control-ref of="1 9"() -> (w1219:refnum<vi>)
                  n777 = property class="Clust (严格)"(reference=w1219) -> ("Controls[]"=w1221:refnum<vi>[])  [unwired: 1 in, 2 out]
                  n778 = for {
                    tunnel: w1221 -> [w1222] mode=indexing
                    tunnel: w1220 -> [w1223] mode=indexing
                    n779 = property class="Ctl"(reference=w1222, "Blinking"=w1223) -> ()  [unwired: 1 in, 2 out]
                  }
                }
                frame 7 {
                  n780 = control-ref of="1 10"() -> (w1224:refnum<vi>)
                  n781 = property class="Clust (严格)"(reference=w1224) -> ("Controls[]"=w1226:refnum<vi>[])  [unwired: 1 in, 2 out]
                  n782 = for {
                    tunnel: w1226 -> [w1227] mode=indexing
                    tunnel: w1225 -> [w1228] mode=indexing
                    n783 = property class="Ctl"(reference=w1227, "Blinking"=w1228) -> ()  [unwired: 1 in, 2 out]
                  }
                }
                frame 8 {
                  n784 = control-ref of="1 26"() -> (w1229:refnum<vi>)
                  n785 = property class="Clust (严格)"(reference=w1229) -> ("Controls[]"=w1231:refnum<vi>[])  [unwired: 1 in, 2 out]
                  n786 = for {
                    tunnel: w1231 -> [w1232] mode=indexing
                    tunnel: w1230 -> [w1233] mode=indexing
                    n787 = property class="Ctl"(reference=w1232, "Blinking"=w1233) -> ()  [unwired: 1 in, 2 out]
                  }
                }
                frame 9 {
                  n788 = control-ref of="1 27"() -> (w1234:refnum<vi>)
                  n789 = property class="Clust (严格)"(reference=w1234) -> ("Controls[]"=w1236:refnum<vi>[])  [unwired: 1 in, 2 out]
                  n790 = for {
                    tunnel: w1236 -> [w1237] mode=indexing
                    tunnel: w1235 -> [w1238] mode=indexing
                    n791 = property class="Ctl"(reference=w1237, "Blinking"=w1238) -> ()  [unwired: 1 in, 2 out]
                  }
                }
                frame 10 {
                  n792 = control-ref of="1 28"() -> (w1239:refnum<vi>)
                  n793 = property class="Clust (严格)"(reference=w1239) -> ("Controls[]"=w1241:refnum<vi>[])  [unwired: 1 in, 2 out]
                  n794 = for {
                    tunnel: w1241 -> [w1242] mode=indexing
                    tunnel: w1240 -> [w1243] mode=indexing
                    n795 = property class="Ctl"(reference=w1242, "Blinking"=w1243) -> ()  [unwired: 1 in, 2 out]
                  }
                }
                frame 11 {
                  n796 = control-ref of="1 29"() -> (w1244:refnum<vi>)
                  n797 = property class="Clust (严格)"(reference=w1244) -> ("Controls[]"=w1246:refnum<vi>[])  [unwired: 1 in, 2 out]
                  n798 = for {
                    tunnel: w1246 -> [w1247] mode=indexing
                    tunnel: w1245 -> [w1248] mode=indexing
                    n799 = property class="Ctl"(reference=w1247, "Blinking"=w1248) -> ()  [unwired: 1 in, 2 out]
                  }
                }
                frame 12 {
                  n800 = control-ref of="1 30"() -> (w1249:refnum<vi>)
                  n801 = property class="Clust (严格)"(reference=w1249) -> ("Controls[]"=w1251:refnum<vi>[])  [unwired: 1 in, 2 out]
                  n802 = for {
                    tunnel: w1251 -> [w1252] mode=indexing
                    tunnel: w1250 -> [w1253] mode=indexing
                    n803 = property class="Ctl"(reference=w1252, "Blinking"=w1253) -> ()  [unwired: 1 in, 2 out]
                  }
                }
                frame 13 {
                  n804 = control-ref of="1 31"() -> (w1254:refnum<vi>)
                  n805 = property class="Clust (严格)"(reference=w1254) -> ("Controls[]"=w1256:refnum<vi>[])  [unwired: 1 in, 2 out]
                  n806 = for {
                    tunnel: w1256 -> [w1257] mode=indexing
                    tunnel: w1255 -> [w1258] mode=indexing
                    n807 = property class="Ctl"(reference=w1257, "Blinking"=w1258) -> ()  [unwired: 1 in, 2 out]
                  }
                }
                frame 14 {
                  n808 = control-ref of="1 32"() -> (w1259:refnum<vi>)
                  n809 = property class="Clust (严格)"(reference=w1259) -> ("Controls[]"=w1261:refnum<vi>[])  [unwired: 1 in, 2 out]
                  n810 = for {
                    tunnel: w1261 -> [w1262] mode=indexing
                    tunnel: w1260 -> [w1263] mode=indexing
                    n811 = property class="Ctl"(reference=w1262, "Blinking"=w1263) -> ()  [unwired: 1 in, 2 out]
                  }
                }
                frame 15 {
                  n812 = control-ref of="1 33"() -> (w1264:refnum<vi>)
                  n813 = property class="Clust (严格)"(reference=w1264) -> ("Controls[]"=w1266:refnum<vi>[])  [unwired: 1 in, 2 out]
                  n814 = for {
                    tunnel: w1266 -> [w1267] mode=indexing
                    tunnel: w1265 -> [w1268] mode=indexing
                    n815 = property class="Ctl"(reference=w1267, "Blinking"=w1268) -> ()  [unwired: 1 in, 2 out]
                  }
                }
                frame 99, Default {
                }
              }
            }
          }
        }
        n816 = local write "一次置位"(TRUE ("一次置位")) -> ()
      }
    }
  }
  n817 = while {
    stop <- w1327 stop-if-true
    n818 = local read "停止"() -> (w1327:bool)
    n819 = Wait Until Next ms Multiple(millisecond multiple=u32 500 ("毫秒倍数")) -> ()  [unwired: 1 out]
    n820 = case shown="真" "213" {
      frame False {
      }
      frame True {
        n821 = local read "选项卡控件"() -> (w1330:enum32{"单体电压", "单体温度", "单体内阻", "单体SOC"})
        n822 = local write "213"(FALSE ("213")) -> ()
        n823 = case shown="\"单体电压\", 默认" w1330 {
          frame "单体电压", Default {
            n824 = global read "单体信息全局.vi" "PF"() -> (w1331:i32)
            n825 = for {
              N: w1331 -> [_]
              tunnel: [TRUE] -> w1332 mode=indexing
            }
            n826 = for {
              N: 16 -> [_]
              tunnel: w1332 -> [w1339]
              i -> [w1340]
              w1337 = 12 ("y")
              n827 = Multiply(x=w1340, y=w1337) -> (x*y=w1338:i32)
              n828 = Array Subset(array=w1339, index=w1338, length=w1337) -> (w1336:bool[])
              n829 = case shown="0" w1340 {
                tunnel: w1336 -> [w1342 w1352 w1363 w1374 w1385 w1396 w1407 w1418 w1429 w1440 w1451 w1462 w1473 w1484 w1495 w1506 _]
                frame 0 {
                  n830 = control-ref of="1 102"() -> (w1344:refnum<vi>)
                  n831 = property class="Clust (严格)"(reference=w1344) -> ("Controls[]"=w1343:refnum<vi>[])  [unwired: 1 in, 2 out]
                  n832 = for {
                    N: 12 -> [_]
                    tunnel: w1343 -> [w1350] mode=indexing
                    tunnel: w1342 -> [w1351]
                    i -> [w1348]
                    n833 = Index Array(array=w1351, index=w1348) -> (element=w1349:bool)
                    n834 = Select(t=0, s=w1349, f=2) -> (s? t:f=w1347:i32)
                    n835 = property class="Ctl"(reference=w1350, "DisabledEnum"=w1347) -> ()  [unwired: 1 in, 2 out]
                  }
                }
                frame 1 {
                  n836 = control-ref of="1 3"() -> (w1355:refnum<vi>)
                  n837 = property class="Clust (严格)"(reference=w1355) -> ("Controls[]"=w1353:refnum<vi>[])  [unwired: 1 in, 2 out]
                  n838 = for {
                    N: 12 -> [_]
                    tunnel: w1353 -> [w1361] mode=indexing
                    tunnel: w1352 -> [w1362]
                    i -> [w1359]
                    n839 = Index Array(array=w1362, index=w1359) -> (element=w1360:bool)
                    n840 = Select(t=0, s=w1360, f=2) -> (s? t:f=w1358:i32)
                    n841 = property class="Ctl"(reference=w1361, "DisabledEnum"=w1358) -> ()  [unwired: 1 in, 2 out]
                  }
                }
                frame 2 {
                  n842 = control-ref of="1 4"() -> (w1366:refnum<vi>)
                  n843 = property class="Clust (严格)"(reference=w1366) -> ("Controls[]"=w1364:refnum<vi>[])  [unwired: 1 in, 2 out]
                  n844 = for {
                    N: 12 -> [_]
                    tunnel: w1364 -> [w1372] mode=indexing
                    tunnel: w1363 -> [w1373]
                    i -> [w1370]
                    n845 = Index Array(array=w1373, index=w1370) -> (element=w1371:bool)
                    n846 = Select(t=0, s=w1371, f=2) -> (s? t:f=w1369:i32)
                    n847 = property class="Ctl"(reference=w1372, "DisabledEnum"=w1369) -> ()  [unwired: 1 in, 2 out]
                  }
                }
                frame 3 {
                  n848 = control-ref of="1 6"() -> (w1377:refnum<vi>)
                  n849 = property class="Clust (严格)"(reference=w1377) -> ("Controls[]"=w1375:refnum<vi>[])  [unwired: 1 in, 2 out]
                  n850 = for {
                    N: 12 -> [_]
                    tunnel: w1375 -> [w1383] mode=indexing
                    tunnel: w1374 -> [w1384]
                    i -> [w1381]
                    n851 = Index Array(array=w1384, index=w1381) -> (element=w1382:bool)
                    n852 = Select(t=0, s=w1382, f=2) -> (s? t:f=w1380:i32)
                    n853 = property class="Ctl"(reference=w1383, "DisabledEnum"=w1380) -> ()  [unwired: 1 in, 2 out]
                  }
                }
                frame 4 {
                  n854 = control-ref of="1 7"() -> (w1388:refnum<vi>)
                  n855 = property class="Clust (严格)"(reference=w1388) -> ("Controls[]"=w1386:refnum<vi>[])  [unwired: 1 in, 2 out]
                  n856 = for {
                    N: 12 -> [_]
                    tunnel: w1386 -> [w1394] mode=indexing
                    tunnel: w1385 -> [w1395]
                    i -> [w1392]
                    n857 = Index Array(array=w1395, index=w1392) -> (element=w1393:bool)
                    n858 = Select(t=0, s=w1393, f=2) -> (s? t:f=w1391:i32)
                    n859 = property class="Ctl"(reference=w1394, "DisabledEnum"=w1391) -> ()  [unwired: 1 in, 2 out]
                  }
                }
                frame 5 {
                  n860 = control-ref of="1 8"() -> (w1399:refnum<vi>)
                  n861 = property class="Clust (严格)"(reference=w1399) -> ("Controls[]"=w1397:refnum<vi>[])  [unwired: 1 in, 2 out]
                  n862 = for {
                    N: 12 -> [_]
                    tunnel: w1397 -> [w1405] mode=indexing
                    tunnel: w1396 -> [w1406]
                    i -> [w1403]
                    n863 = Index Array(array=w1406, index=w1403) -> (element=w1404:bool)
                    n864 = Select(t=0, s=w1404, f=2) -> (s? t:f=w1402:i32)
                    n865 = property class="Ctl"(reference=w1405, "DisabledEnum"=w1402) -> ()  [unwired: 1 in, 2 out]
                  }
                }
                frame 6 {
                  n866 = control-ref of="1 9"() -> (w1410:refnum<vi>)
                  n867 = property class="Clust (严格)"(reference=w1410) -> ("Controls[]"=w1408:refnum<vi>[])  [unwired: 1 in, 2 out]
                  n868 = for {
                    N: 12 -> [_]
                    tunnel: w1408 -> [w1416] mode=indexing
                    tunnel: w1407 -> [w1417]
                    i -> [w1414]
                    n869 = Index Array(array=w1417, index=w1414) -> (element=w1415:bool)
                    n870 = Select(t=0, s=w1415, f=2) -> (s? t:f=w1413:i32)
                    n871 = property class="Ctl"(reference=w1416, "DisabledEnum"=w1413) -> ()  [unwired: 1 in, 2 out]
                  }
                }
                frame 7 {
                  n872 = control-ref of="1 10"() -> (w1421:refnum<vi>)
                  n873 = property class="Clust (严格)"(reference=w1421) -> ("Controls[]"=w1419:refnum<vi>[])  [unwired: 1 in, 2 out]
                  n874 = for {
                    N: 12 -> [_]
                    tunnel: w1419 -> [w1427] mode=indexing
                    tunnel: w1418 -> [w1428]
                    i -> [w1425]
                    n875 = Index Array(array=w1428, index=w1425) -> (element=w1426:bool)
                    n876 = Select(t=0, s=w1426, f=2) -> (s? t:f=w1424:i32)
                    n877 = property class="Ctl"(reference=w1427, "DisabledEnum"=w1424) -> ()  [unwired: 1 in, 2 out]
                  }
                }
                frame 8 {
                  n878 = control-ref of="1 26"() -> (w1432:refnum<vi>)
                  n879 = property class="Clust (严格)"(reference=w1432) -> ("Controls[]"=w1430:refnum<vi>[])  [unwired: 1 in, 2 out]
                  n880 = for {
                    N: 12 -> [_]
                    tunnel: w1430 -> [w1438] mode=indexing
                    tunnel: w1429 -> [w1439]
                    i -> [w1436]
                    n881 = Index Array(array=w1439, index=w1436) -> (element=w1437:bool)
                    n882 = Select(t=0, s=w1437, f=2) -> (s? t:f=w1435:i32)
                    n883 = property class="Ctl"(reference=w1438, "DisabledEnum"=w1435) -> ()  [unwired: 1 in, 2 out]
                  }
                }
                frame 9 {
                  n884 = control-ref of="1 27"() -> (w1443:refnum<vi>)
                  n885 = property class="Clust (严格)"(reference=w1443) -> ("Controls[]"=w1441:refnum<vi>[])  [unwired: 1 in, 2 out]
                  n886 = for {
                    N: 12 -> [_]
                    tunnel: w1441 -> [w1449] mode=indexing
                    tunnel: w1440 -> [w1450]
                    i -> [w1447]
                    n887 = Index Array(array=w1450, index=w1447) -> (element=w1448:bool)
                    n888 = Select(t=0, s=w1448, f=2) -> (s? t:f=w1446:i32)
                    n889 = property class="Ctl"(reference=w1449, "DisabledEnum"=w1446) -> ()  [unwired: 1 in, 2 out]
                  }
                }
                frame 10 {
                  n890 = control-ref of="1 28"() -> (w1454:refnum<vi>)
                  n891 = property class="Clust (严格)"(reference=w1454) -> ("Controls[]"=w1452:refnum<vi>[])  [unwired: 1 in, 2 out]
                  n892 = for {
                    N: 12 -> [_]
                    tunnel: w1452 -> [w1460] mode=indexing
                    tunnel: w1451 -> [w1461]
                    i -> [w1458]
                    n893 = Index Array(array=w1461, index=w1458) -> (element=w1459:bool)
                    n894 = Select(t=0, s=w1459, f=2) -> (s? t:f=w1457:i32)
                    n895 = property class="Ctl"(reference=w1460, "DisabledEnum"=w1457) -> ()  [unwired: 1 in, 2 out]
                  }
                }
                frame 11 {
                  n896 = control-ref of="1 29"() -> (w1465:refnum<vi>)
                  n897 = property class="Clust (严格)"(reference=w1465) -> ("Controls[]"=w1463:refnum<vi>[])  [unwired: 1 in, 2 out]
                  n898 = for {
                    N: 12 -> [_]
                    tunnel: w1463 -> [w1471] mode=indexing
                    tunnel: w1462 -> [w1472]
                    i -> [w1469]
                    n899 = Index Array(array=w1472, index=w1469) -> (element=w1470:bool)
                    n900 = Select(t=0, s=w1470, f=2) -> (s? t:f=w1468:i32)
                    n901 = property class="Ctl"(reference=w1471, "DisabledEnum"=w1468) -> ()  [unwired: 1 in, 2 out]
                  }
                }
                frame 12 {
                  n902 = control-ref of="1 30"() -> (w1476:refnum<vi>)
                  n903 = property class="Clust (严格)"(reference=w1476) -> ("Controls[]"=w1474:refnum<vi>[])  [unwired: 1 in, 2 out]
                  n904 = for {
                    N: 12 -> [_]
                    tunnel: w1474 -> [w1482] mode=indexing
                    tunnel: w1473 -> [w1483]
                    i -> [w1480]
                    n905 = Index Array(array=w1483, index=w1480) -> (element=w1481:bool)
                    n906 = Select(t=0, s=w1481, f=2) -> (s? t:f=w1479:i32)
                    n907 = property class="Ctl"(reference=w1482, "DisabledEnum"=w1479) -> ()  [unwired: 1 in, 2 out]
                  }
                }
                frame 13 {
                  n908 = control-ref of="1 31"() -> (w1487:refnum<vi>)
                  n909 = property class="Clust (严格)"(reference=w1487) -> ("Controls[]"=w1485:refnum<vi>[])  [unwired: 1 in, 2 out]
                  n910 = for {
                    N: 12 -> [_]
                    tunnel: w1485 -> [w1493] mode=indexing
                    tunnel: w1484 -> [w1494]
                    i -> [w1491]
                    n911 = Index Array(array=w1494, index=w1491) -> (element=w1492:bool)
                    n912 = Select(t=0, s=w1492, f=2) -> (s? t:f=w1490:i32)
                    n913 = property class="Ctl"(reference=w1493, "DisabledEnum"=w1490) -> ()  [unwired: 1 in, 2 out]
                  }
                }
                frame 14 {
                  n914 = control-ref of="1 32"() -> (w1498:refnum<vi>)
                  n915 = property class="Clust (严格)"(reference=w1498) -> ("Controls[]"=w1496:refnum<vi>[])  [unwired: 1 in, 2 out]
                  n916 = for {
                    N: 12 -> [_]
                    tunnel: w1496 -> [w1504] mode=indexing
                    tunnel: w1495 -> [w1505]
                    i -> [w1502]
                    n917 = Index Array(array=w1505, index=w1502) -> (element=w1503:bool)
                    n918 = Select(t=0, s=w1503, f=2) -> (s? t:f=w1501:i32)
                    n919 = property class="Ctl"(reference=w1504, "DisabledEnum"=w1501) -> ()  [unwired: 1 in, 2 out]
                  }
                }
                frame 15 {
                  n920 = control-ref of="1 33"() -> (w1509:refnum<vi>)
                  n921 = property class="Clust (严格)"(reference=w1509) -> ("Controls[]"=w1507:refnum<vi>[])  [unwired: 1 in, 2 out]
                  n922 = for {
                    N: 12 -> [_]
                    tunnel: w1507 -> [w1515] mode=indexing
                    tunnel: w1506 -> [w1516]
                    i -> [w1513]
                    n923 = Index Array(array=w1516, index=w1513) -> (element=w1514:bool)
                    n924 = Select(t=0, s=w1514, f=2) -> (s? t:f=w1512:i32)
                    n925 = property class="Ctl"(reference=w1515, "DisabledEnum"=w1512) -> ()  [unwired: 1 in, 2 out]
                  }
                }
                frame 99, Default {
                }
              }
            }
            n926 = for {
              N: 9 -> [_]
              tunnel: w1332 -> [w1522]
              i -> [w1523]
              w1520 = 12 ("y")
              n927 = Add(x=16, y=w1523) -> (x+y=w1518:i32)
              n928 = Multiply(x=w1518, y=w1520) -> (x*y=w1521:i32)
              n929 = Array Subset(array=w1522, index=w1521, length=w1520) -> (w1519:bool[])
              n930 = case shown="8" w1523 {
                tunnel: w1519 -> [w1524 w1535 w1546 w1557 w1568 w1579 w1590 w1601 w1612 _]
                frame 0 {
                  n931 = control-ref of="1 18"() -> (w1527:refnum<vi>)
                  n932 = property class="Clust (严格)"(reference=w1527) -> ("Controls[]"=w1525:refnum<vi>[])  [unwired: 1 in, 2 out]
                  n933 = for {
                    N: 12 -> [_]
                    tunnel: w1525 -> [w1533] mode=indexing
                    tunnel: w1524 -> [w1534]
                    i -> [w1531]
                    n934 = Index Array(array=w1534, index=w1531) -> (element=w1532:bool)
                    n935 = Select(t=0, s=w1532, f=2) -> (s? t:f=w1530:i32)
                    n936 = property class="Ctl"(reference=w1533, "DisabledEnum"=w1530) -> ()  [unwired: 1 in, 2 out]
                  }
                }
                frame 1 {
                  n937 = control-ref of="1 19"() -> (w1538:refnum<vi>)
                  n938 = property class="Clust (严格)"(reference=w1538) -> ("Controls[]"=w1536:refnum<vi>[])  [unwired: 1 in, 2 out]
                  n939 = for {
                    N: 12 -> [_]
                    tunnel: w1536 -> [w1544] mode=indexing
                    tunnel: w1535 -> [w1545]
                    i -> [w1542]
                    n940 = Index Array(array=w1545, index=w1542) -> (element=w1543:bool)
                    n941 = Select(t=0, s=w1543, f=2) -> (s? t:f=w1541:i32)
                    n942 = property class="Ctl"(reference=w1544, "DisabledEnum"=w1541) -> ()  [unwired: 1 in, 2 out]
                  }
                }
                frame 2 {
                  n943 = control-ref of="1 20"() -> (w1549:refnum<vi>)
                  n944 = property class="Clust (严格)"(reference=w1549) -> ("Controls[]"=w1547:refnum<vi>[])  [unwired: 1 in, 2 out]
                  n945 = for {
                    N: 12 -> [_]
                    tunnel: w1547 -> [w1555] mode=indexing
                    tunnel: w1546 -> [w1556]
                    i -> [w1553]
                    n946 = Index Array(array=w1556, index=w1553) -> (element=w1554:bool)
                    n947 = Select(t=0, s=w1554, f=2) -> (s? t:f=w1552:i32)
                    n948 = property class="Ctl"(reference=w1555, "DisabledEnum"=w1552) -> ()  [unwired: 1 in, 2 out]
                  }
                }
                frame 3 {
                  n949 = control-ref of="1 21"() -> (w1560:refnum<vi>)
                  n950 = property class="Clust (严格)"(reference=w1560) -> ("Controls[]"=w1558:refnum<vi>[])  [unwired: 1 in, 2 out]
                  n951 = for {
                    N: 12 -> [_]
                    tunnel: w1558 -> [w1566] mode=indexing
                    tunnel: w1557 -> [w1567]
                    i -> [w1564]
                    n952 = Index Array(array=w1567, index=w1564) -> (element=w1565:bool)
                    n953 = Select(t=0, s=w1565, f=2) -> (s? t:f=w1563:i32)
                    n954 = property class="Ctl"(reference=w1566, "DisabledEnum"=w1563) -> ()  [unwired: 1 in, 2 out]
                  }
                }
                frame 4 {
                  n955 = control-ref of="1 22"() -> (w1571:refnum<vi>)
                  n956 = property class="Clust (严格)"(reference=w1571) -> ("Controls[]"=w1569:refnum<vi>[])  [unwired: 1 in, 2 out]
                  n957 = for {
                    N: 12 -> [_]
                    tunnel: w1569 -> [w1577] mode=indexing
                    tunnel: w1568 -> [w1578]
                    i -> [w1575]
                    n958 = Index Array(array=w1578, index=w1575) -> (element=w1576:bool)
                    n959 = Select(t=0, s=w1576, f=2) -> (s? t:f=w1574:i32)
                    n960 = property class="Ctl"(reference=w1577, "DisabledEnum"=w1574) -> ()  [unwired: 1 in, 2 out]
                  }
                }
                frame 5 {
                  n961 = control-ref of="1 23"() -> (w1582:refnum<vi>)
                  n962 = property class="Clust (严格)"(reference=w1582) -> ("Controls[]"=w1580:refnum<vi>[])  [unwired: 1 in, 2 out]
                  n963 = for {
                    N: 12 -> [_]
                    tunnel: w1580 -> [w1588] mode=indexing
                    tunnel: w1579 -> [w1589]
                    i -> [w1586]
                    n964 = Index Array(array=w1589, index=w1586) -> (element=w1587:bool)
                    n965 = Select(t=0, s=w1587, f=2) -> (s? t:f=w1585:i32)
                    n966 = property class="Ctl"(reference=w1588, "DisabledEnum"=w1585) -> ()  [unwired: 1 in, 2 out]
                  }
                }
                frame 6 {
                  n967 = control-ref of="1 24"() -> (w1593:refnum<vi>)
                  n968 = property class="Clust (严格)"(reference=w1593) -> ("Controls[]"=w1591:refnum<vi>[])  [unwired: 1 in, 2 out]
                  n969 = for {
                    N: 12 -> [_]
                    tunnel: w1591 -> [w1599] mode=indexing
                    tunnel: w1590 -> [w1600]
                    i -> [w1597]
                    n970 = Index Array(array=w1600, index=w1597) -> (element=w1598:bool)
                    n971 = Select(t=0, s=w1598, f=2) -> (s? t:f=w1596:i32)
                    n972 = property class="Ctl"(reference=w1599, "DisabledEnum"=w1596) -> ()  [unwired: 1 in, 2 out]
                  }
                }
                frame 7 {
                  n973 = control-ref of="1 25"() -> (w1604:refnum<vi>)
                  n974 = property class="Clust (严格)"(reference=w1604) -> ("Controls[]"=w1602:refnum<vi>[])  [unwired: 1 in, 2 out]
                  n975 = for {
                    N: 12 -> [_]
                    tunnel: w1602 -> [w1610] mode=indexing
                    tunnel: w1601 -> [w1611]
                    i -> [w1608]
                    n976 = Index Array(array=w1611, index=w1608) -> (element=w1609:bool)
                    n977 = Select(t=0, s=w1609, f=2) -> (s? t:f=w1607:i32)
                    n978 = property class="Ctl"(reference=w1610, "DisabledEnum"=w1607) -> ()  [unwired: 1 in, 2 out]
                  }
                }
                frame 8 {
                  n979 = control-ref of="1 5"() -> (w1615:refnum<vi>)
                  n980 = property class="Clust (严格)"(reference=w1615) -> ("Controls[]"=w1613:refnum<vi>[])  [unwired: 1 in, 2 out]
                  n981 = for {
                    N: 12 -> [_]
                    tunnel: w1613 -> [w1621] mode=indexing
                    tunnel: w1612 -> [w1622]
                    i -> [w1619]
                    n982 = Index Array(array=w1622, index=w1619) -> (element=w1620:bool)
                    n983 = Select(t=0, s=w1620, f=2) -> (s? t:f=w1618:i32)
                    n984 = property class="Ctl"(reference=w1621, "DisabledEnum"=w1618) -> ()  [unwired: 1 in, 2 out]
                  }
                }
                frame 99, Default {
                }
              }
            }
          }
          frame "单体温度" {
            n985 = global read "单体信息全局.vi" "PF2"() -> (w1623:i32)
            n986 = for {
              N: w1623 -> [_]
              tunnel: [TRUE] -> w1624 mode=indexing
            }
            n987 = for {
              N: 9 -> [_]
              tunnel: w1624 -> [w1814]
              i -> [w1815]
              w1812 = 12 ("y")
              n988 = Add(x=16, y=w1815) -> (x+y=w1810:i32)
              n989 = Multiply(x=w1810, y=w1812) -> (x*y=w1813:i32)
              n990 = Array Subset(array=w1814, index=w1813, length=w1812) -> (w1811:bool[])
              n991 = case shown="0" w1815 {
                tunnel: w1811 -> [w1816 w1827 w1838 w1849 w1860 w1871 w1882 w1893 w1904 _]
                frame 0 {
                  n992 = control-ref of="1 18"() -> (w1819:refnum<vi>)
                  n993 = property class="Clust (严格)"(reference=w1819) -> ("Controls[]"=w1817:refnum<vi>[])  [unwired: 1 in, 2 out]
                  n994 = for {
                    N: 12 -> [_]
                    tunnel: w1817 -> [w1825] mode=indexing
                    tunnel: w1816 -> [w1826]
                    i -> [w1823]
                    n995 = Index Array(array=w1826, index=w1823) -> (element=w1824:bool)
                    n996 = Select(t=0, s=w1824, f=2) -> (s? t:f=w1822:i32)
                    n997 = property class="Ctl"(reference=w1825, "DisabledEnum"=w1822) -> ()  [unwired: 1 in, 2 out]
                  }
                }
                frame 1 {
                  n998 = control-ref of="1 19"() -> (w1830:refnum<vi>)
                  n999 = property class="Clust (严格)"(reference=w1830) -> ("Controls[]"=w1828:refnum<vi>[])  [unwired: 1 in, 2 out]
                  n1000 = for {
                    N: 12 -> [_]
                    tunnel: w1828 -> [w1836] mode=indexing
                    tunnel: w1827 -> [w1837]
                    i -> [w1834]
                    n1001 = Index Array(array=w1837, index=w1834) -> (element=w1835:bool)
                    n1002 = Select(t=0, s=w1835, f=2) -> (s? t:f=w1833:i32)
                    n1003 = property class="Ctl"(reference=w1836, "DisabledEnum"=w1833) -> ()  [unwired: 1 in, 2 out]
                  }
                }
                frame 2 {
                  n1004 = control-ref of="1 20"() -> (w1841:refnum<vi>)
                  n1005 = property class="Clust (严格)"(reference=w1841) -> ("Controls[]"=w1839:refnum<vi>[])  [unwired: 1 in, 2 out]
                  n1006 = for {
                    N: 12 -> [_]
                    tunnel: w1839 -> [w1847] mode=indexing
                    tunnel: w1838 -> [w1848]
                    i -> [w1845]
                    n1007 = Index Array(array=w1848, index=w1845) -> (element=w1846:bool)
                    n1008 = Select(t=0, s=w1846, f=2) -> (s? t:f=w1844:i32)
                    n1009 = property class="Ctl"(reference=w1847, "DisabledEnum"=w1844) -> ()  [unwired: 1 in, 2 out]
                  }
                }
                frame 3 {
                  n1010 = control-ref of="1 21"() -> (w1852:refnum<vi>)
                  n1011 = property class="Clust (严格)"(reference=w1852) -> ("Controls[]"=w1850:refnum<vi>[])  [unwired: 1 in, 2 out]
                  n1012 = for {
                    N: 12 -> [_]
                    tunnel: w1850 -> [w1858] mode=indexing
                    tunnel: w1849 -> [w1859]
                    i -> [w1856]
                    n1013 = Index Array(array=w1859, index=w1856) -> (element=w1857:bool)
                    n1014 = Select(t=0, s=w1857, f=2) -> (s? t:f=w1855:i32)
                    n1015 = property class="Ctl"(reference=w1858, "DisabledEnum"=w1855) -> ()  [unwired: 1 in, 2 out]
                  }
                }
                frame 4 {
                  n1016 = control-ref of="1 22"() -> (w1863:refnum<vi>)
                  n1017 = property class="Clust (严格)"(reference=w1863) -> ("Controls[]"=w1861:refnum<vi>[])  [unwired: 1 in, 2 out]
                  n1018 = for {
                    N: 12 -> [_]
                    tunnel: w1861 -> [w1869] mode=indexing
                    tunnel: w1860 -> [w1870]
                    i -> [w1867]
                    n1019 = Index Array(array=w1870, index=w1867) -> (element=w1868:bool)
                    n1020 = Select(t=0, s=w1868, f=2) -> (s? t:f=w1866:i32)
                    n1021 = property class="Ctl"(reference=w1869, "DisabledEnum"=w1866) -> ()  [unwired: 1 in, 2 out]
                  }
                }
                frame 5 {
                  n1022 = control-ref of="1 23"() -> (w1874:refnum<vi>)
                  n1023 = property class="Clust (严格)"(reference=w1874) -> ("Controls[]"=w1872:refnum<vi>[])  [unwired: 1 in, 2 out]
                  n1024 = for {
                    N: 12 -> [_]
                    tunnel: w1872 -> [w1880] mode=indexing
                    tunnel: w1871 -> [w1881]
                    i -> [w1878]
                    n1025 = Index Array(array=w1881, index=w1878) -> (element=w1879:bool)
                    n1026 = Select(t=0, s=w1879, f=2) -> (s? t:f=w1877:i32)
                    n1027 = property class="Ctl"(reference=w1880, "DisabledEnum"=w1877) -> ()  [unwired: 1 in, 2 out]
                  }
                }
                frame 6 {
                  n1028 = control-ref of="1 24"() -> (w1885:refnum<vi>)
                  n1029 = property class="Clust (严格)"(reference=w1885) -> ("Controls[]"=w1883:refnum<vi>[])  [unwired: 1 in, 2 out]
                  n1030 = for {
                    N: 12 -> [_]
                    tunnel: w1883 -> [w1891] mode=indexing
                    tunnel: w1882 -> [w1892]
                    i -> [w1889]
                    n1031 = Index Array(array=w1892, index=w1889) -> (element=w1890:bool)
                    n1032 = Select(t=0, s=w1890, f=2) -> (s? t:f=w1888:i32)
                    n1033 = property class="Ctl"(reference=w1891, "DisabledEnum"=w1888) -> ()  [unwired: 1 in, 2 out]
                  }
                }
                frame 7 {
                  n1034 = control-ref of="1 25"() -> (w1896:refnum<vi>)
                  n1035 = property class="Clust (严格)"(reference=w1896) -> ("Controls[]"=w1894:refnum<vi>[])  [unwired: 1 in, 2 out]
                  n1036 = for {
                    N: 12 -> [_]
                    tunnel: w1894 -> [w1902] mode=indexing
                    tunnel: w1893 -> [w1903]
                    i -> [w1900]
                    n1037 = Index Array(array=w1903, index=w1900) -> (element=w1901:bool)
                    n1038 = Select(t=0, s=w1901, f=2) -> (s? t:f=w1899:i32)
                    n1039 = property class="Ctl"(reference=w1902, "DisabledEnum"=w1899) -> ()  [unwired: 1 in, 2 out]
                  }
                }
                frame 8 {
                  n1040 = control-ref of="1 6"() -> (w1907:refnum<vi>)
                  n1041 = property class="Clust (严格)"(reference=w1907) -> ("Controls[]"=w1905:refnum<vi>[])  [unwired: 1 in, 2 out]
                  n1042 = for {
                    N: 12 -> [_]
                    tunnel: w1905 -> [w1913] mode=indexing
                    tunnel: w1904 -> [w1914]
                    i -> [w1911]
                    n1043 = Index Array(array=w1914, index=w1911) -> (element=w1912:bool)
                    n1044 = Select(t=0, s=w1912, f=2) -> (s? t:f=w1910:i32)
                    n1045 = property class="Ctl"(reference=w1913, "DisabledEnum"=w1910) -> ()  [unwired: 1 in, 2 out]
                  }
                }
                frame 99, Default {
                }
              }
            }
            n1046 = for {
              N: 16 -> [_]
              tunnel: w1624 -> [w1631]
              i -> [w1632]
              w1629 = 12 ("y")
              n1047 = Multiply(x=w1632, y=w1629) -> (x*y=w1630:i32)
              n1048 = Array Subset(array=w1631, index=w1630, length=w1629) -> (w1628:bool[])
              n1049 = case shown="15" w1632 {
                tunnel: w1628 -> [w1633 w1644 w1655 w1666 w1677 w1688 w1699 w1710 w1721 w1732 w1743 w1754 w1765 w1776 w1787 w1798 _]
                frame 0 {
                  n1050 = control-ref of="1 102"() -> (w1636:refnum<vi>)
                  n1051 = property class="Clust (严格)"(reference=w1636) -> ("Controls[]"=w1634:refnum<vi>[])  [unwired: 1 in, 2 out]
                  n1052 = for {
                    N: 12 -> [_]
                    tunnel: w1634 -> [w1642] mode=indexing
                    tunnel: w1633 -> [w1643]
                    i -> [w1640]
                    n1053 = Index Array(array=w1643, index=w1640) -> (element=w1641:bool)
                    n1054 = Select(t=0, s=w1641, f=2) -> (s? t:f=w1639:i32)
                    n1055 = property class="Ctl"(reference=w1642, "DisabledEnum"=w1639) -> ()  [unwired: 1 in, 2 out]
                  }
                }
                frame 1 {
                  n1056 = control-ref of="1 3"() -> (w1647:refnum<vi>)
                  n1057 = property class="Clust (严格)"(reference=w1647) -> ("Controls[]"=w1645:refnum<vi>[])  [unwired: 1 in, 2 out]
                  n1058 = for {
                    N: 12 -> [_]
                    tunnel: w1645 -> [w1653] mode=indexing
                    tunnel: w1644 -> [w1654]
                    i -> [w1651]
                    n1059 = Index Array(array=w1654, index=w1651) -> (element=w1652:bool)
                    n1060 = Select(t=0, s=w1652, f=2) -> (s? t:f=w1650:i32)
                    n1061 = property class="Ctl"(reference=w1653, "DisabledEnum"=w1650) -> ()  [unwired: 1 in, 2 out]
                  }
                }
                frame 2 {
                  n1062 = control-ref of="1 4"() -> (w1658:refnum<vi>)
                  n1063 = property class="Clust (严格)"(reference=w1658) -> ("Controls[]"=w1656:refnum<vi>[])  [unwired: 1 in, 2 out]
                  n1064 = for {
                    N: 12 -> [_]
                    tunnel: w1656 -> [w1664] mode=indexing
                    tunnel: w1655 -> [w1665]
                    i -> [w1662]
                    n1065 = Index Array(array=w1665, index=w1662) -> (element=w1663:bool)
                    n1066 = Select(t=0, s=w1663, f=2) -> (s? t:f=w1661:i32)
                    n1067 = property class="Ctl"(reference=w1664, "DisabledEnum"=w1661) -> ()  [unwired: 1 in, 2 out]
                  }
                }
                frame 3 {
                  n1068 = control-ref of="1 6"() -> (w1669:refnum<vi>)
                  n1069 = property class="Clust (严格)"(reference=w1669) -> ("Controls[]"=w1667:refnum<vi>[])  [unwired: 1 in, 2 out]
                  n1070 = for {
                    N: 12 -> [_]
                    tunnel: w1667 -> [w1675] mode=indexing
                    tunnel: w1666 -> [w1676]
                    i -> [w1673]
                    n1071 = Index Array(array=w1676, index=w1673) -> (element=w1674:bool)
                    n1072 = Select(t=0, s=w1674, f=2) -> (s? t:f=w1672:i32)
                    n1073 = property class="Ctl"(reference=w1675, "DisabledEnum"=w1672) -> ()  [unwired: 1 in, 2 out]
                  }
                }
                frame 4 {
                  n1074 = control-ref of="1 7"() -> (w1680:refnum<vi>)
                  n1075 = property class="Clust (严格)"(reference=w1680) -> ("Controls[]"=w1678:refnum<vi>[])  [unwired: 1 in, 2 out]
                  n1076 = for {
                    N: 12 -> [_]
                    tunnel: w1678 -> [w1686] mode=indexing
                    tunnel: w1677 -> [w1687]
                    i -> [w1684]
                    n1077 = Index Array(array=w1687, index=w1684) -> (element=w1685:bool)
                    n1078 = Select(t=0, s=w1685, f=2) -> (s? t:f=w1683:i32)
                    n1079 = property class="Ctl"(reference=w1686, "DisabledEnum"=w1683) -> ()  [unwired: 1 in, 2 out]
                  }
                }
                frame 5 {
                  n1080 = control-ref of="1 8"() -> (w1691:refnum<vi>)
                  n1081 = property class="Clust (严格)"(reference=w1691) -> ("Controls[]"=w1689:refnum<vi>[])  [unwired: 1 in, 2 out]
                  n1082 = for {
                    N: 12 -> [_]
                    tunnel: w1689 -> [w1697] mode=indexing
                    tunnel: w1688 -> [w1698]
                    i -> [w1695]
                    n1083 = Index Array(array=w1698, index=w1695) -> (element=w1696:bool)
                    n1084 = Select(t=0, s=w1696, f=2) -> (s? t:f=w1694:i32)
                    n1085 = property class="Ctl"(reference=w1697, "DisabledEnum"=w1694) -> ()  [unwired: 1 in, 2 out]
                  }
                }
                frame 6 {
                  n1086 = control-ref of="1 9"() -> (w1702:refnum<vi>)
                  n1087 = property class="Clust (严格)"(reference=w1702) -> ("Controls[]"=w1700:refnum<vi>[])  [unwired: 1 in, 2 out]
                  n1088 = for {
                    N: 12 -> [_]
                    tunnel: w1700 -> [w1708] mode=indexing
                    tunnel: w1699 -> [w1709]
                    i -> [w1706]
                    n1089 = Index Array(array=w1709, index=w1706) -> (element=w1707:bool)
                    n1090 = Select(t=0, s=w1707, f=2) -> (s? t:f=w1705:i32)
                    n1091 = property class="Ctl"(reference=w1708, "DisabledEnum"=w1705) -> ()  [unwired: 1 in, 2 out]
                  }
                }
                frame 7 {
                  n1092 = control-ref of="1 10"() -> (w1713:refnum<vi>)
                  n1093 = property class="Clust (严格)"(reference=w1713) -> ("Controls[]"=w1711:refnum<vi>[])  [unwired: 1 in, 2 out]
                  n1094 = for {
                    N: 12 -> [_]
                    tunnel: w1711 -> [w1719] mode=indexing
                    tunnel: w1710 -> [w1720]
                    i -> [w1717]
                    n1095 = Index Array(array=w1720, index=w1717) -> (element=w1718:bool)
                    n1096 = Select(t=0, s=w1718, f=2) -> (s? t:f=w1716:i32)
                    n1097 = property class="Ctl"(reference=w1719, "DisabledEnum"=w1716) -> ()  [unwired: 1 in, 2 out]
                  }
                }
                frame 8 {
                  n1098 = control-ref of="1 26"() -> (w1724:refnum<vi>)
                  n1099 = property class="Clust (严格)"(reference=w1724) -> ("Controls[]"=w1722:refnum<vi>[])  [unwired: 1 in, 2 out]
                  n1100 = for {
                    N: 12 -> [_]
                    tunnel: w1722 -> [w1730] mode=indexing
                    tunnel: w1721 -> [w1731]
                    i -> [w1728]
                    n1101 = Index Array(array=w1731, index=w1728) -> (element=w1729:bool)
                    n1102 = Select(t=0, s=w1729, f=2) -> (s? t:f=w1727:i32)
                    n1103 = property class="Ctl"(reference=w1730, "DisabledEnum"=w1727) -> ()  [unwired: 1 in, 2 out]
                  }
                }
                frame 9 {
                  n1104 = control-ref of="1 27"() -> (w1735:refnum<vi>)
                  n1105 = property class="Clust (严格)"(reference=w1735) -> ("Controls[]"=w1733:refnum<vi>[])  [unwired: 1 in, 2 out]
                  n1106 = for {
                    N: 12 -> [_]
                    tunnel: w1733 -> [w1741] mode=indexing
                    tunnel: w1732 -> [w1742]
                    i -> [w1739]
                    n1107 = Index Array(array=w1742, index=w1739) -> (element=w1740:bool)
                    n1108 = Select(t=0, s=w1740, f=2) -> (s? t:f=w1738:i32)
                    n1109 = property class="Ctl"(reference=w1741, "DisabledEnum"=w1738) -> ()  [unwired: 1 in, 2 out]
                  }
                }
                frame 10 {
                  n1110 = control-ref of="1 28"() -> (w1746:refnum<vi>)
                  n1111 = property class="Clust (严格)"(reference=w1746) -> ("Controls[]"=w1744:refnum<vi>[])  [unwired: 1 in, 2 out]
                  n1112 = for {
                    N: 12 -> [_]
                    tunnel: w1744 -> [w1752] mode=indexing
                    tunnel: w1743 -> [w1753]
                    i -> [w1750]
                    n1113 = Index Array(array=w1753, index=w1750) -> (element=w1751:bool)
                    n1114 = Select(t=0, s=w1751, f=2) -> (s? t:f=w1749:i32)
                    n1115 = property class="Ctl"(reference=w1752, "DisabledEnum"=w1749) -> ()  [unwired: 1 in, 2 out]
                  }
                }
                frame 11 {
                  n1116 = control-ref of="1 29"() -> (w1757:refnum<vi>)
                  n1117 = property class="Clust (严格)"(reference=w1757) -> ("Controls[]"=w1755:refnum<vi>[])  [unwired: 1 in, 2 out]
                  n1118 = for {
                    N: 12 -> [_]
                    tunnel: w1755 -> [w1763] mode=indexing
                    tunnel: w1754 -> [w1764]
                    i -> [w1761]
                    n1119 = Index Array(array=w1764, index=w1761) -> (element=w1762:bool)
                    n1120 = Select(t=0, s=w1762, f=2) -> (s? t:f=w1760:i32)
                    n1121 = property class="Ctl"(reference=w1763, "DisabledEnum"=w1760) -> ()  [unwired: 1 in, 2 out]
                  }
                }
                frame 12 {
                  n1122 = control-ref of="1 30"() -> (w1768:refnum<vi>)
                  n1123 = property class="Clust (严格)"(reference=w1768) -> ("Controls[]"=w1766:refnum<vi>[])  [unwired: 1 in, 2 out]
                  n1124 = for {
                    N: 12 -> [_]
                    tunnel: w1766 -> [w1774] mode=indexing
                    tunnel: w1765 -> [w1775]
                    i -> [w1772]
                    n1125 = Index Array(array=w1775, index=w1772) -> (element=w1773:bool)
                    n1126 = Select(t=0, s=w1773, f=2) -> (s? t:f=w1771:i32)
                    n1127 = property class="Ctl"(reference=w1774, "DisabledEnum"=w1771) -> ()  [unwired: 1 in, 2 out]
                  }
                }
                frame 13 {
                  n1128 = control-ref of="1 31"() -> (w1779:refnum<vi>)
                  n1129 = property class="Clust (严格)"(reference=w1779) -> ("Controls[]"=w1777:refnum<vi>[])  [unwired: 1 in, 2 out]
                  n1130 = for {
                    N: 12 -> [_]
                    tunnel: w1777 -> [w1785] mode=indexing
                    tunnel: w1776 -> [w1786]
                    i -> [w1783]
                    n1131 = Index Array(array=w1786, index=w1783) -> (element=w1784:bool)
                    n1132 = Select(t=0, s=w1784, f=2) -> (s? t:f=w1782:i32)
                    n1133 = property class="Ctl"(reference=w1785, "DisabledEnum"=w1782) -> ()  [unwired: 1 in, 2 out]
                  }
                }
                frame 14 {
                  n1134 = control-ref of="1 32"() -> (w1790:refnum<vi>)
                  n1135 = property class="Clust (严格)"(reference=w1790) -> ("Controls[]"=w1788:refnum<vi>[])  [unwired: 1 in, 2 out]
                  n1136 = for {
                    N: 12 -> [_]
                    tunnel: w1788 -> [w1796] mode=indexing
                    tunnel: w1787 -> [w1797]
                    i -> [w1794]
                    n1137 = Index Array(array=w1797, index=w1794) -> (element=w1795:bool)
                    n1138 = Select(t=0, s=w1795, f=2) -> (s? t:f=w1793:i32)
                    n1139 = property class="Ctl"(reference=w1796, "DisabledEnum"=w1793) -> ()  [unwired: 1 in, 2 out]
                  }
                }
                frame 15 {
                  n1140 = control-ref of="1 33"() -> (w1801:refnum<vi>)
                  n1141 = property class="Clust (严格)"(reference=w1801) -> ("Controls[]"=w1799:refnum<vi>[])  [unwired: 1 in, 2 out]
                  n1142 = for {
                    N: 12 -> [_]
                    tunnel: w1799 -> [w1807] mode=indexing
                    tunnel: w1798 -> [w1808]
                    i -> [w1805]
                    n1143 = Index Array(array=w1808, index=w1805) -> (element=w1806:bool)
                    n1144 = Select(t=0, s=w1806, f=2) -> (s? t:f=w1804:i32)
                    n1145 = property class="Ctl"(reference=w1807, "DisabledEnum"=w1804) -> ()  [unwired: 1 in, 2 out]
                  }
                }
                frame 99, Default {
                }
              }
            }
          }
        }
      }
    }
  }
  n1146 = local write "213"(TRUE ("213")) -> ()
  n1147 = disable-structure shown="禁用" {
    frame Disabled {
      n1148 = control-ref of="选项卡控件"() -> (w1915:refnum<vi>)
      n1149 = control-ref of="均衡信息"() -> (w1916:refnum<vi>)
      n1150 = call "单数据解析_new.vi"(8:w1915) -> ("PF"=w1918:i32, "均衡标记"=w1917:i32[][])  [unwired: 1 in, 8 out]
      n1151 = call "均衡解析.vi"("位置"=w1918, "均衡标记"=w1917, "均衡引用"=w1916) -> ()  [unwired: 9 out]
    }
    frame Enabled {
    }
  }
  n1152 = local write "一次置位"(TRUE ("一次置位")) -> ()
  n1153 = for {
    N: 16 -> [_]
    i -> [w1920]
    n1154 = case shown="15" w1920 {
      tunnel: bool[] [FALSE, FALSE, FALSE, FALSE, FALSE, FALSE, FALSE, FALSE, FALSE, FALSE, FALSE, FALSE, FALSE] -> [w1922 w1927 w1932 w1937 w1942 w1947 w1952 w1957 w1962 w1967 w1972 w1977 w1982 w1987 w1992 w1997 _]
      frame 0 {
        n1155 = control-ref of="1 102"() -> (w1921:refnum<vi>)
        n1156 = property class="Clust (严格)"(reference=w1921) -> ("Controls[]"=w1923:refnum<vi>[])  [unwired: 1 in, 2 out]
        n1157 = for {
          tunnel: w1923 -> [w1924] mode=indexing
          tunnel: w1922 -> [w1925] mode=indexing
          n1158 = property class="Ctl"(reference=w1924, "Blinking"=w1925) -> ()  [unwired: 1 in, 2 out]
        }
      }
      frame 1 {
        n1159 = control-ref of="1 3"() -> (w1926:refnum<vi>)
        n1160 = property class="Clust (严格)"(reference=w1926) -> ("Controls[]"=w1928:refnum<vi>[])  [unwired: 1 in, 2 out]
        n1161 = for {
          tunnel: w1928 -> [w1929] mode=indexing
          tunnel: w1927 -> [w1930] mode=indexing
          n1162 = property class="Ctl"(reference=w1929, "Blinking"=w1930) -> ()  [unwired: 1 in, 2 out]
        }
      }
      frame 2 {
        n1163 = control-ref of="1 4"() -> (w1931:refnum<vi>)
        n1164 = property class="Clust (严格)"(reference=w1931) -> ("Controls[]"=w1933:refnum<vi>[])  [unwired: 1 in, 2 out]
        n1165 = for {
          tunnel: w1933 -> [w1934] mode=indexing
          tunnel: w1932 -> [w1935] mode=indexing
          n1166 = property class="Ctl"(reference=w1934, "Blinking"=w1935) -> ()  [unwired: 1 in, 2 out]
        }
      }
      frame 3 {
        n1167 = control-ref of="1 6"() -> (w1936:refnum<vi>)
        n1168 = property class="Clust (严格)"(reference=w1936) -> ("Controls[]"=w1938:refnum<vi>[])  [unwired: 1 in, 2 out]
        n1169 = for {
          tunnel: w1938 -> [w1939] mode=indexing
          tunnel: w1937 -> [w1940] mode=indexing
          n1170 = property class="Ctl"(reference=w1939, "Blinking"=w1940) -> ()  [unwired: 1 in, 2 out]
        }
      }
      frame 4 {
        n1171 = control-ref of="1 7"() -> (w1941:refnum<vi>)
        n1172 = property class="Clust (严格)"(reference=w1941) -> ("Controls[]"=w1943:refnum<vi>[])  [unwired: 1 in, 2 out]
        n1173 = for {
          tunnel: w1943 -> [w1944] mode=indexing
          tunnel: w1942 -> [w1945] mode=indexing
          n1174 = property class="Ctl"(reference=w1944, "Blinking"=w1945) -> ()  [unwired: 1 in, 2 out]
        }
      }
      frame 5 {
        n1175 = control-ref of="1 8"() -> (w1946:refnum<vi>)
        n1176 = property class="Clust (严格)"(reference=w1946) -> ("Controls[]"=w1948:refnum<vi>[])  [unwired: 1 in, 2 out]
        n1177 = for {
          tunnel: w1948 -> [w1949] mode=indexing
          tunnel: w1947 -> [w1950] mode=indexing
          n1178 = property class="Ctl"(reference=w1949, "Blinking"=w1950) -> ()  [unwired: 1 in, 2 out]
        }
      }
      frame 6 {
        n1179 = control-ref of="1 9"() -> (w1951:refnum<vi>)
        n1180 = property class="Clust (严格)"(reference=w1951) -> ("Controls[]"=w1953:refnum<vi>[])  [unwired: 1 in, 2 out]
        n1181 = for {
          tunnel: w1953 -> [w1954] mode=indexing
          tunnel: w1952 -> [w1955] mode=indexing
          n1182 = property class="Ctl"(reference=w1954, "Blinking"=w1955) -> ()  [unwired: 1 in, 2 out]
        }
      }
      frame 7 {
        n1183 = control-ref of="1 10"() -> (w1956:refnum<vi>)
        n1184 = property class="Clust (严格)"(reference=w1956) -> ("Controls[]"=w1958:refnum<vi>[])  [unwired: 1 in, 2 out]
        n1185 = for {
          tunnel: w1958 -> [w1959] mode=indexing
          tunnel: w1957 -> [w1960] mode=indexing
          n1186 = property class="Ctl"(reference=w1959, "Blinking"=w1960) -> ()  [unwired: 1 in, 2 out]
        }
      }
      frame 8 {
        n1187 = control-ref of="1 26"() -> (w1961:refnum<vi>)
        n1188 = property class="Clust (严格)"(reference=w1961) -> ("Controls[]"=w1963:refnum<vi>[])  [unwired: 1 in, 2 out]
        n1189 = for {
          tunnel: w1963 -> [w1964] mode=indexing
          tunnel: w1962 -> [w1965] mode=indexing
          n1190 = property class="Ctl"(reference=w1964, "Blinking"=w1965) -> ()  [unwired: 1 in, 2 out]
        }
      }
      frame 9 {
        n1191 = control-ref of="1 27"() -> (w1966:refnum<vi>)
        n1192 = property class="Clust (严格)"(reference=w1966) -> ("Controls[]"=w1968:refnum<vi>[])  [unwired: 1 in, 2 out]
        n1193 = for {
          tunnel: w1968 -> [w1969] mode=indexing
          tunnel: w1967 -> [w1970] mode=indexing
          n1194 = property class="Ctl"(reference=w1969, "Blinking"=w1970) -> ()  [unwired: 1 in, 2 out]
        }
      }
      frame 10 {
        n1195 = control-ref of="1 28"() -> (w1971:refnum<vi>)
        n1196 = property class="Clust (严格)"(reference=w1971) -> ("Controls[]"=w1973:refnum<vi>[])  [unwired: 1 in, 2 out]
        n1197 = for {
          tunnel: w1973 -> [w1974] mode=indexing
          tunnel: w1972 -> [w1975] mode=indexing
          n1198 = property class="Ctl"(reference=w1974, "Blinking"=w1975) -> ()  [unwired: 1 in, 2 out]
        }
      }
      frame 11 {
        n1199 = control-ref of="1 29"() -> (w1976:refnum<vi>)
        n1200 = property class="Clust (严格)"(reference=w1976) -> ("Controls[]"=w1978:refnum<vi>[])  [unwired: 1 in, 2 out]
        n1201 = for {
          tunnel: w1978 -> [w1979] mode=indexing
          tunnel: w1977 -> [w1980] mode=indexing
          n1202 = property class="Ctl"(reference=w1979, "Blinking"=w1980) -> ()  [unwired: 1 in, 2 out]
        }
      }
      frame 12 {
        n1203 = control-ref of="1 30"() -> (w1981:refnum<vi>)
        n1204 = property class="Clust (严格)"(reference=w1981) -> ("Controls[]"=w1983:refnum<vi>[])  [unwired: 1 in, 2 out]
        n1205 = for {
          tunnel: w1983 -> [w1984] mode=indexing
          tunnel: w1982 -> [w1985] mode=indexing
          n1206 = property class="Ctl"(reference=w1984, "Blinking"=w1985) -> ()  [unwired: 1 in, 2 out]
        }
      }
      frame 13 {
        n1207 = control-ref of="1 31"() -> (w1986:refnum<vi>)
        n1208 = property class="Clust (严格)"(reference=w1986) -> ("Controls[]"=w1988:refnum<vi>[])  [unwired: 1 in, 2 out]
        n1209 = for {
          tunnel: w1988 -> [w1989] mode=indexing
          tunnel: w1987 -> [w1990] mode=indexing
          n1210 = property class="Ctl"(reference=w1989, "Blinking"=w1990) -> ()  [unwired: 1 in, 2 out]
        }
      }
      frame 14 {
        n1211 = control-ref of="1 32"() -> (w1991:refnum<vi>)
        n1212 = property class="Clust (严格)"(reference=w1991) -> ("Controls[]"=w1993:refnum<vi>[])  [unwired: 1 in, 2 out]
        n1213 = for {
          tunnel: w1993 -> [w1994] mode=indexing
          tunnel: w1992 -> [w1995] mode=indexing
          n1214 = property class="Ctl"(reference=w1994, "Blinking"=w1995) -> ()  [unwired: 1 in, 2 out]
        }
      }
      frame 15 {
        n1215 = control-ref of="1 33"() -> (w1996:refnum<vi>)
        n1216 = property class="Clust (严格)"(reference=w1996) -> ("Controls[]"=w1998:refnum<vi>[])  [unwired: 1 in, 2 out]
        n1217 = for {
          tunnel: w1998 -> [w1999] mode=indexing
          tunnel: w1997 -> [w2000] mode=indexing
          n1218 = property class="Ctl"(reference=w1999, "Blinking"=w2000) -> ()  [unwired: 1 in, 2 out]
        }
      }
      frame 99, Default {
      }
    }
  }
  n1219 = for {
    N: 9 -> [_]
    i -> [w2002]
    n1220 = case shown="8" w2002 {
      tunnel: bool[] [FALSE, FALSE, FALSE, FALSE, FALSE, FALSE, FALSE, FALSE, FALSE, FALSE, FALSE, FALSE, FALSE] -> [w2004 w2009 w2014 w2019 w2024 w2029 w2034 w2039 w2044 _]
      frame 0 {
        n1221 = control-ref of="1 18"() -> (w2003:refnum<vi>)
        n1222 = property class="Clust (严格)"(reference=w2003) -> ("Controls[]"=w2005:refnum<vi>[])  [unwired: 1 in, 2 out]
        n1223 = for {
          tunnel: w2005 -> [w2006] mode=indexing
          tunnel: w2004 -> [w2007] mode=indexing
          n1224 = property class="Ctl"(reference=w2006, "Blinking"=w2007) -> ()  [unwired: 1 in, 2 out]
        }
      }
      frame 1 {
        n1225 = control-ref of="1 19"() -> (w2008:refnum<vi>)
        n1226 = property class="Clust (严格)"(reference=w2008) -> ("Controls[]"=w2010:refnum<vi>[])  [unwired: 1 in, 2 out]
        n1227 = for {
          tunnel: w2010 -> [w2011] mode=indexing
          tunnel: w2009 -> [w2012] mode=indexing
          n1228 = property class="Ctl"(reference=w2011, "Blinking"=w2012) -> ()  [unwired: 1 in, 2 out]
        }
      }
      frame 2 {
        n1229 = control-ref of="1 20"() -> (w2013:refnum<vi>)
        n1230 = property class="Clust (严格)"(reference=w2013) -> ("Controls[]"=w2015:refnum<vi>[])  [unwired: 1 in, 2 out]
        n1231 = for {
          tunnel: w2015 -> [w2016] mode=indexing
          tunnel: w2014 -> [w2017] mode=indexing
          n1232 = property class="Ctl"(reference=w2016, "Blinking"=w2017) -> ()  [unwired: 1 in, 2 out]
        }
      }
      frame 3 {
        n1233 = control-ref of="1 21"() -> (w2018:refnum<vi>)
        n1234 = property class="Clust (严格)"(reference=w2018) -> ("Controls[]"=w2020:refnum<vi>[])  [unwired: 1 in, 2 out]
        n1235 = for {
          tunnel: w2020 -> [w2021] mode=indexing
          tunnel: w2019 -> [w2022] mode=indexing
          n1236 = property class="Ctl"(reference=w2021, "Blinking"=w2022) -> ()  [unwired: 1 in, 2 out]
        }
      }
      frame 4 {
        n1237 = control-ref of="1 22"() -> (w2023:refnum<vi>)
        n1238 = property class="Clust (严格)"(reference=w2023) -> ("Controls[]"=w2025:refnum<vi>[])  [unwired: 1 in, 2 out]
        n1239 = for {
          tunnel: w2025 -> [w2026] mode=indexing
          tunnel: w2024 -> [w2027] mode=indexing
          n1240 = property class="Ctl"(reference=w2026, "Blinking"=w2027) -> ()  [unwired: 1 in, 2 out]
        }
      }
      frame 5 {
        n1241 = control-ref of="1 23"() -> (w2028:refnum<vi>)
        n1242 = property class="Clust (严格)"(reference=w2028) -> ("Controls[]"=w2030:refnum<vi>[])  [unwired: 1 in, 2 out]
        n1243 = for {
          tunnel: w2030 -> [w2031] mode=indexing
          tunnel: w2029 -> [w2032] mode=indexing
          n1244 = property class="Ctl"(reference=w2031, "Blinking"=w2032) -> ()  [unwired: 1 in, 2 out]
        }
      }
      frame 6 {
        n1245 = control-ref of="1 24"() -> (w2033:refnum<vi>)
        n1246 = property class="Clust (严格)"(reference=w2033) -> ("Controls[]"=w2035:refnum<vi>[])  [unwired: 1 in, 2 out]
        n1247 = for {
          tunnel: w2035 -> [w2036] mode=indexing
          tunnel: w2034 -> [w2037] mode=indexing
          n1248 = property class="Ctl"(reference=w2036, "Blinking"=w2037) -> ()  [unwired: 1 in, 2 out]
        }
      }
      frame 7 {
        n1249 = control-ref of="1 25"() -> (w2038:refnum<vi>)
        n1250 = property class="Clust (严格)"(reference=w2038) -> ("Controls[]"=w2040:refnum<vi>[])  [unwired: 1 in, 2 out]
        n1251 = for {
          tunnel: w2040 -> [w2041] mode=indexing
          tunnel: w2039 -> [w2042] mode=indexing
          n1252 = property class="Ctl"(reference=w2041, "Blinking"=w2042) -> ()  [unwired: 1 in, 2 out]
        }
      }
      frame 8 {
        n1253 = control-ref of="1 6"() -> (w2043:refnum<vi>)
        n1254 = property class="Clust (严格)"(reference=w2043) -> ("Controls[]"=w2045:refnum<vi>[])  [unwired: 1 in, 2 out]
        n1255 = for {
          tunnel: w2045 -> [w2046] mode=indexing
          tunnel: w2044 -> [w2047] mode=indexing
          n1256 = property class="Ctl"(reference=w2046, "Blinking"=w2047) -> ()  [unwired: 1 in, 2 out]
        }
      }
      frame 99, Default {
      }
    }
  }
  n1257 = local write "充电均衡"(T9 {"充电1"=13816530, "充电1"=13816530, "充电1"=13816530, "充电1"=13816530, "充电1"=13816530, "充电1"=13816530, "充电1"=13816530, "充电1"=13816530, "充电1"=13816530, "充电1"=13816530, "充电1"=13816530, "充电1"=13816530} ("充电均衡")) -> ()
  n1258 = disable-structure shown="禁用" {
    frame Disabled {
      n1259 = Not A Number/Path/Refnum?(number/path/refnum="数据") -> (NaN/Path/Refnum?=w2052:bool)
      n1260 = Not A Number/Path/Refnum?(number/path/refnum="数据位置") -> (NaN/Path/Refnum?=w2051:bool)
      n1261 = Or(x=w2052, y=w2051) -> (x .or. y?=w2050:bool)
      n1262 = case shown="假" w2050 {
        tunnel: "数据位置" -> [w2056 _]
        tunnel: "数据" -> [w2054 _]
        frame False {
          n1263 = property class="Arr (严格)"(reference=w2056) -> ("Value"=w2055:dbl[])  [unwired: 1 in, 2 out]
          n1264 = property class="Arr (严格)"(reference=w2054) -> ("Value"=w2053:dbl[])  [unwired: 1 in, 2 out]
          n1265 = call "数组去零.vi"("输入"=w2055) -> ("输出"=w2057:dbl[])
          n1266 = Array Size(array=w2057) -> (size(s)=w2058:i32)
          n1267 = Quotient & Remainder(x=w2058, y=24) -> (x-y*floor(x/y)=w2064:i32, floor(x/y)=w2061:i32)
          n1268 = Equal To 0?(x=w2064) -> (x = 0?=w2063:bool)
          n1269 = Increment(x=w2061) -> (x+1=w2060:i32)
          n1270 = Select(t=w2061, s=w2063, f=w2060) -> (s? t:f=w2062:i32)
          n1271 = Array Subset(array=w2053, length=w2058) -> (w2066:dbl[])  [unwired: 1 in]
          n1272 = for {
            N: w2062 -> [_]
            tunnel: w2066 -> [w2079]
            tunnel: [w2070] -> w2059
            tunnel: w2057 -> [w2073]
            i -> [w2076]
            w2071 = 24 ("y")
            n1273 = Multiply(x=w2076, y=w2071) -> (x*y=w2072:i32)
            n1274 = Increment(x=w2076) -> (x+1=w2074:i32)
            n1275 = Array Subset(array=w2079, index=w2072, length=w2071) -> (w2075:dbl[])
            n1276 = Array Subset(array=w2073, index=w2072, length=w2071) -> (w2069:dbl[])
            n1277 = Multiply(x=w2074, y=3) -> (x*y=w2077:i32)
            n1278 = Decrement(x=w2077) -> (x-1=w2068:i32)
            n1279 = Decrement(x=w2068) -> (x-1=w2067:i32)
            n1280 = call "表格数据输入(数值)-8.6.vi"("列数"=w2067, "数值数组"=w2069, "表格引用"=w2070) -> ()  [unwired: 9 out]
            n1281 = call "表格数据输入(数值)-8.6.vi"("列数"=w2068, "数值数组"=w2075, "表格引用"=w2070) -> ()  [unwired: 9 out]
          }
        }
        frame True {
        }
      }
    }
    frame Enabled {
    }
  }
  n1282 = disable-structure shown="禁用" {
    frame Disabled {
      n1283 = Multiply(x=12, y=24) -> (x*y=w2086:i32)
      n1284 = for {
        N: 12 -> [_]
        tunnel: [w2091] -> w2088 mode=indexing
        tunnel: [w2090] -> _
        tunnel: w2086 -> [w2090]
        i -> [w2097]
        n1285 = Increment(x=w2097) -> (x+1=w2096:i32)
        n1286 = Add(x=w2090, y=w2096) -> (x+y=w2092:i32)
        n1287 = Number To Decimal String(number=w2092) -> (decimal integer string=w2095:string)  [unwired: 1 out]
        n1288 = Concatenate Strings("第" ("字符串"), w2095, "串" ("字符串")) -> (w2091:string)
      }
      n1289 = Multiply(x=12, y=3) -> (x*y=w2083:i32)
      n1290 = call "表格数据输入-8.6.vi"("行数"=u32 0, "列数"=w2083, "字符串数组"=w2088) -> ("表格引用"=w2089:refnum<vi>)  [unwired: 8 out]
    }
    frame Enabled {
    }
  }
  n1291 = local write "停止"(FALSE ("停止")) -> ()
  "单选选项2" <- FALSE ("单选选项2")
